vi "mainIRTesting.vi"() -> ()   [LabVIEW 2024]
doc: "Main VI for FLS imaging system."
uses:
  <userlib>/_OpenG.lib/file/file.llb/openg_file.lvlib
  <vilib>/event_ctls.llb/usereventprio.ctl
  <instrlib>/niScope/Acquire/Fetch/niScope Multi Fetch Binary 16.vi
  <instrlib>/niScope/Controls/niScope trigger source.ctl
  <userlib>/_OpenG.lib/time/time.llb/openg_time.lvlib
  LaguerreDeconLib/DeconEngineClass/LaguerreDeconEngineClass.lvclass
  SubVI/GlobalVariables.vi
  SubVI/LabJack/LJ Pin Setting.ctl
  <vilib>/Utility/error.llb/DialogType.ctl
  <vilib>/Analysis/NI_AALBase.lvlib
  <vilib>/Utility/miscctls.llb/LVMinMaxIncTypeDef.ctl
  <vilib>/Analysis/baseanly.llb/Mean (DBL).vi
  <vilib>/Utility/miscctls.llb/LVPointTypeDef.ctl
  <vilib>/addons/_JKI.lib/Serialization/JSON/JKI JSON Serialization.lvlib
  SubVI/APD/APDClass.lvclass
  ConfigFiles/AimingBeamVideoConfig.ctl
  <vilib>/addons/control/pid/NI_PID_pid.lvlib
  <vilib>/addons/control/pid/pid.llb/PID (DBL).vi
  <vilib>/Instr/_visa.llb/VISA Configure Serial Port (Instr).vi
  SubVI/DigitizerConfiguration/FLImDAQ.ctl
panel:
  in  "Square Wave?":bool
  in  "aimplitude":dbl=0.5 format="%#_13g"
  in  "aplitude":dbl=0.5 format="%#_13g"
  in  "amplitude":dbl=0.4
  in  "Modulation?":bool
  in  "f (Hz)":dbl=1.0
  in  "Gain DC 3":dbl
  in  "f (Hz)":dbl=1.0
  in  "Gain DC":dbl
  in  "Modulation?":bool
  in  "f (Hz)":dbl=1.0
  out "Peak3":dbl
  out "Peak2":dbl
  out "Peak1":dbl
  out "DC3":dbl format="%0.2f"
  out "DC2":dbl format="%0.2f"
  out "DC1":dbl format="%0.2f"
  in  "Gain DC":dbl
  in  "Modulation?":bool
  in  "V target(1.0)":dbl=1.0 caption="V target(1.5)" min=0.3 max=1.5 step=0.1 format="%#_4g"
  out "SNR3":dbl format="%#_3g"
  out "SNR2":dbl format="%#_3g"
  out "SNR1":dbl format="%#_3g"
  in  "Show BG removed?":bool
  out "IntR3":dbl format="%#_2g"
  out "IntR2":dbl format="%#_2g"
  out "IntR1":dbl format="%#_2g"
  in  "Video Display":bool
  out "Gain3":dbl
  out "Gain2":dbl
  out "Gain1":dbl
  in  "Skip Data Save?":bool
  out "Aq Loop?":bool
  out "ML?":bool
  out "aquisition loop Error Out":errorcluster
  out "Laser f (Hz)":dbl
  out "remote address":string
  out "Record Backlog":i32
  out "Fetch Record #":i32
  out "Sync Success?":bool
  out "Disclamer":picture
  out "Calibration #":i8
  out "BG #":i8
  in  "TCP Connect":bool
  out "Help":string
  in  "355nm Laser toggle":bool caption="355nm 460Hz"
  in  "Cali&iRF alignment":bool
  in  "Background":bool
  in  "Aiming beam toggle":bool caption="445nm 2Hz 22mA"
  out "Lifetime 3":dbl
  out "Lifetime 2":dbl
  in  "Auto gain ch3":bool=TRUE
  in  "Auto gain ch2":bool=TRUE
  in  "Auto gain ch1":bool=TRUE
  out "Run #":i8
  in  "StopButton":bool caption="Stop"
  out "Aquisition Status:":bool
  in  "StartButton":bool caption="Start"
  in  "V 3":dbl caption="Gain 3" min=0.0 max=4.65 step=0.1
  in  "V 2":dbl caption="Gain 2" min=0.0 max=4.59 step=0.1
  out "Lifetime 1":dbl
  in  "V 1":dbl caption="Gain 1" min=0.0 max=4.63 step=0.1 format="%#_4g"
  in  "Video Source":enum32{"Camera", "FrameGrabber"}(radio)
  out "Case #":string
  out "System Hardware Connection Status":T1
  out "Channel 3":dbl[][](graph)
  out "Channel 2":dbl[][](graph)
  out "Channel 1":dbl[][](graph)
  in  "Tab Control":T2(tab)
  out "display loop timing(ms)":u32
  out "Aquisition loop timing(ms)":u32 format="%.2f"
  out "DisplayLoop":i32
  out "PID loop":i32 caption="processing loop"
  out "PID loop timing(ms)":u32 caption="processing loop timing(ms)"
  out "Communication loop(ms)":u32
  out "laser EM lamp V":dbl format="%0.6f"
  out "Decon Loop timing (ms)":dbl
  in  "Show BG":bool
  out "iRF length":i32
  out "data length":i32
  out "BG length":i32
  out "SysConfigCluster":T3
  out "LJ Pinout":T4={"Ch1 Bias"="DAC0", "Ch2 Bias"="DAC1", "Ch3 Bias"="DAC2", "Ch4 Bias"="DAC0", "355 PWM"="FIO0", "AimingBeam PWM"="FIO2", "Laser Ready"="FIO3", "Interlock"="FIO1", "Laser Start/Stop"="FIO1", "Red LED"="FIO1", "Green LED"="DIO3", "Foot Pedal"="DIO15"}
  out "FLImDAQ":T5={"Digitizer 1"="", "Digitizer 2"="", "Channel"=enum."Channel 0", "trigger source"="VAL_EXTERNAL", "trigger level"=0.5, "trigger delay"=1.35e-07, "min sample rate"=12500000000.0, "min record length"=2500, "vertical range"=1.0, "vertical offset"=-0.25, "Waveform to Avg"=2000} caption="FLIm DAQ Configuration" {"trigger delay" format="%^#.4e"; "trigger level" min=0.0 max=3.5 step=0.5 format="%.2f"; "vertical offset" format="%.4f"; "vertical range" format="%.2f"; "min sample rate" format="%#.2p"}
  out "Dig1 Temp":dbl
  out "Dig2 Temp":dbl
  in  "Sys Reconfig":bool
  out "data out(communcation loop)":string
  out "syctimer data out":string
  out "PID loop error out":errorcluster caption="processing Error Out"
  out "decon error out":errorcluster
  out "Laser Rep Rate":dbl
  in  "Data Class":enum16{"Data", "BG", "Cali"}(ring)
  out "V1 Size":i32
  out "V2 Size":i32
  out "V3 Size":i32
  out "data Size":i32[](array[numeric])
  out "State log":string
  in  "Ch3 PID gains":T7={"proportional gain (Kc)"=30.0, "integral time (Ti, min)"=0.0003, "derivative time (Td, min)"=1e-05}
  in  "Ch2 PID gains":T7={"proportional gain (Kc)"=30.0, "integral time (Ti, min)"=0.0003, "derivative time (Td, min)"=1e-05}
  in  "Ch1 PID gains":T7={"proportional gain (Kc)"=30.0, "integral time (Ti, min)"=0.0003, "derivative time (Td, min)"=1e-05}
  in  "Quit":bool
  in  "Radio Buttons":enum32{"No Selection", "Ch1", "Ch2", "Ch3"}(radio)=enum."Ch1" caption="DeCon Chan"
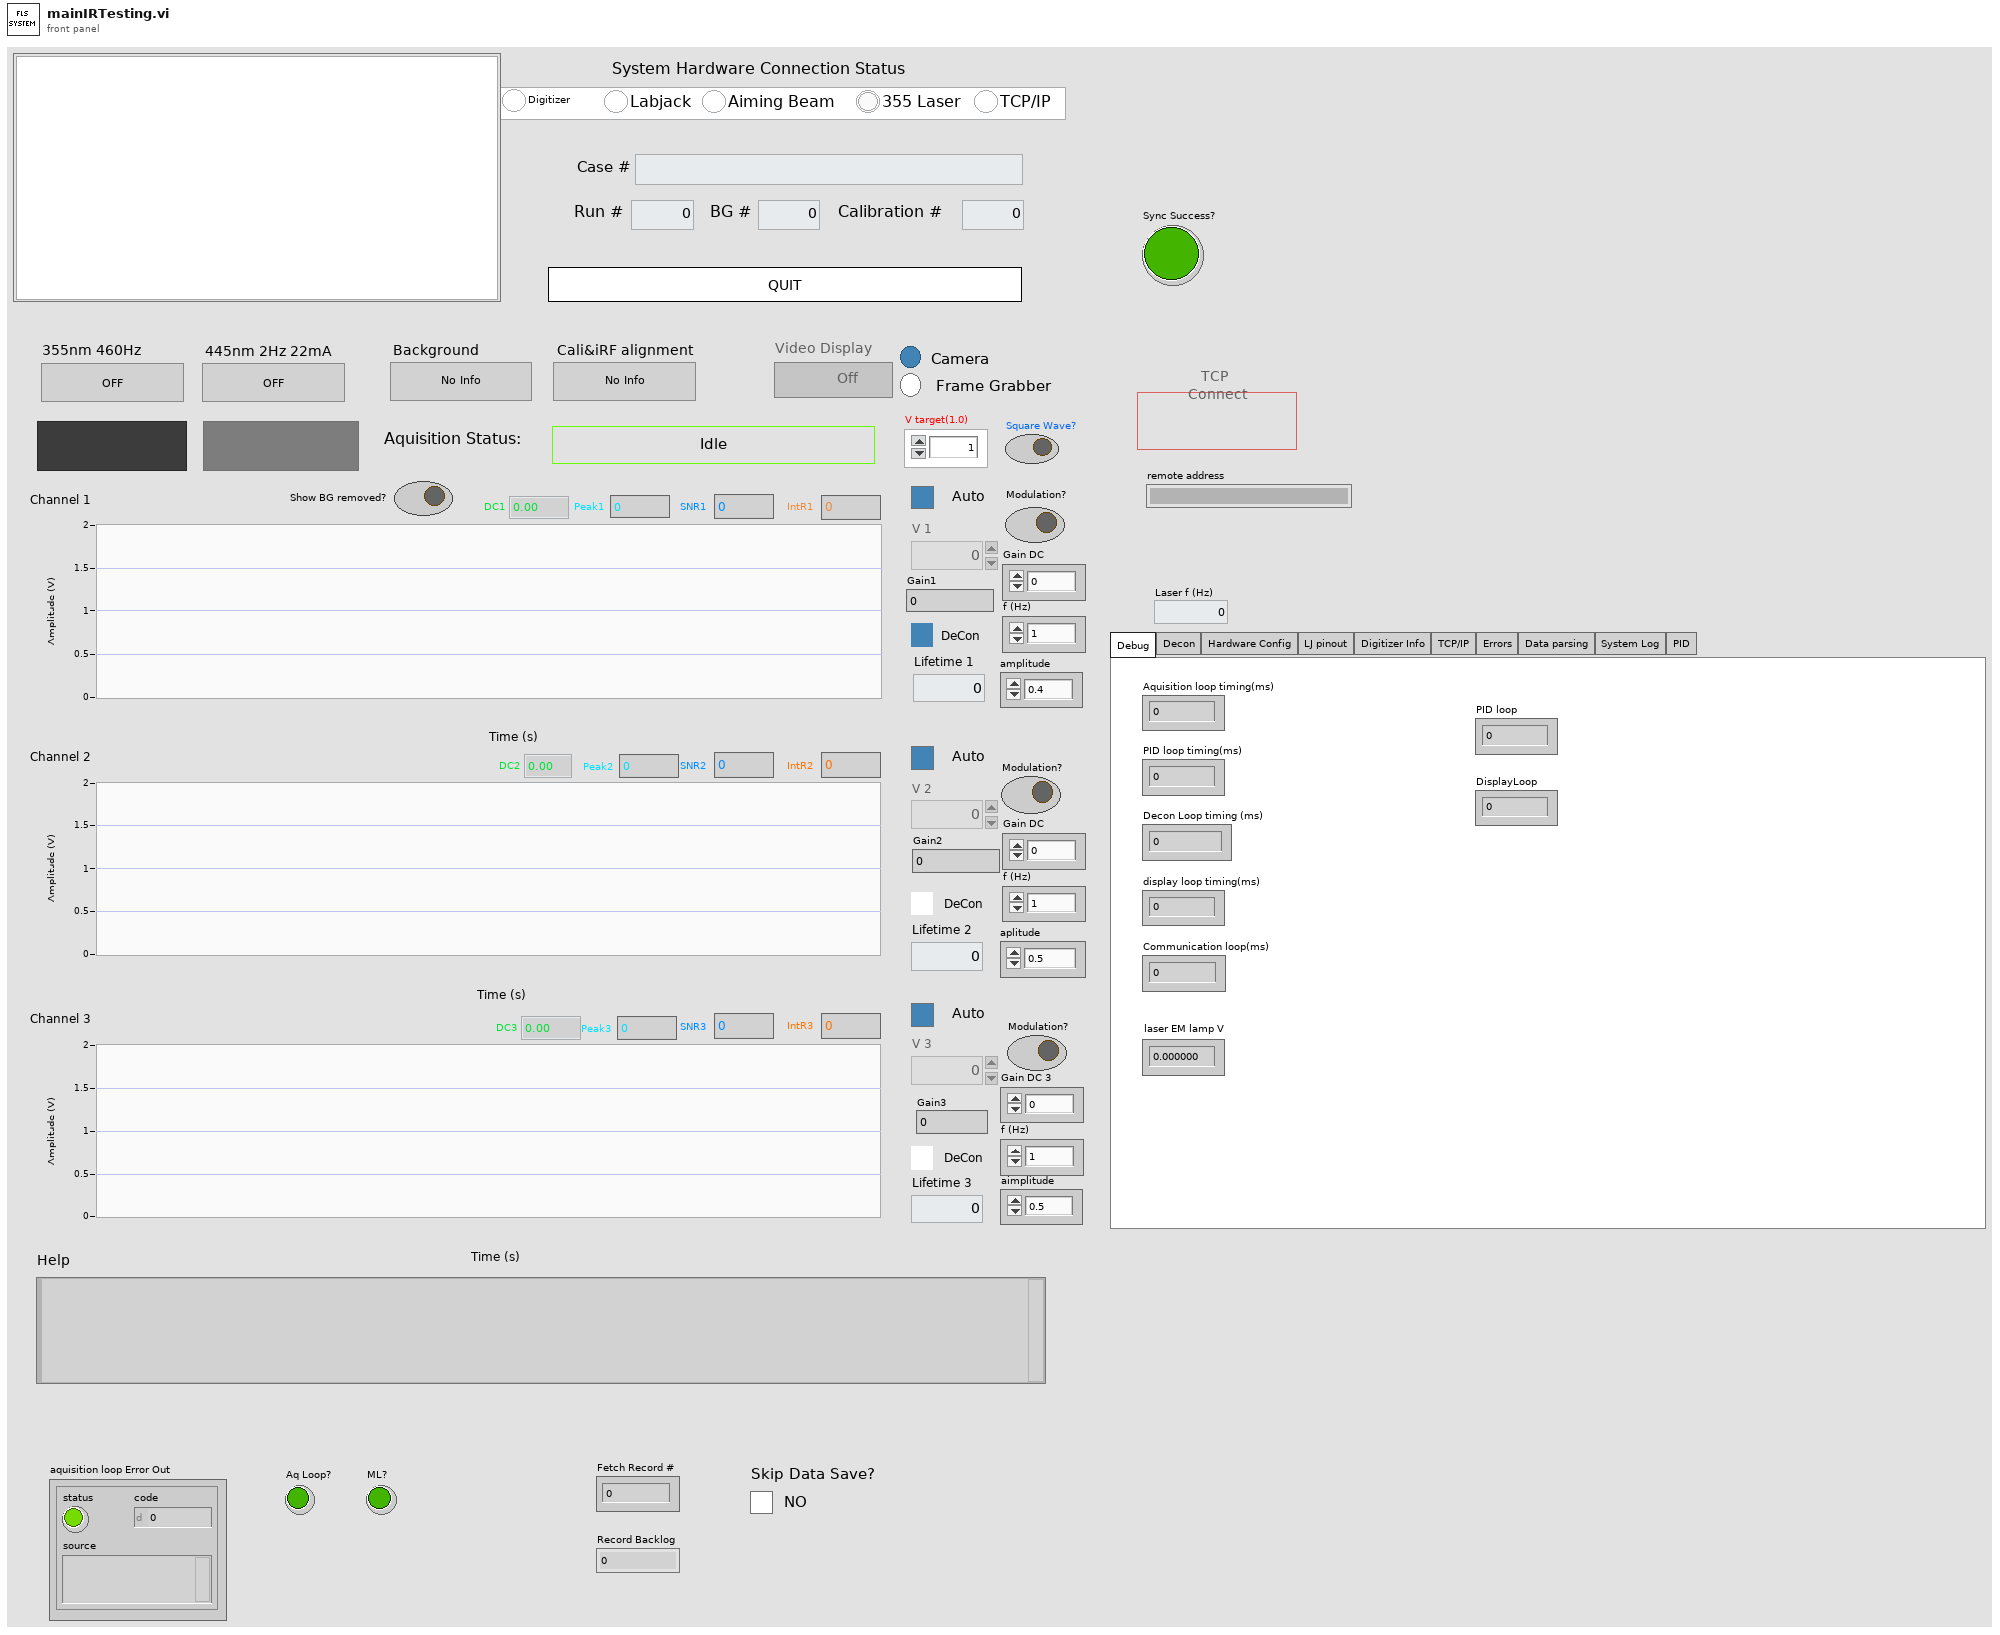
[diagram p1: front panel]
types:
  T1 = cluster{"Digitizer":bool, "Labjack":bool, "Aiming Beam":bool, "355 Laser":bool, "TCP/IP":bool}
  T2 = enum32{"Debug", "Decon", "Hardware Config", "LJ pinout", "Digitizer Info", "TCP/IP", "Errors", "Data parsing", "System Log", "PID"}
  T3 = cluster{"Ch1Enable?":bool, "Ch2Enable?":bool, "Ch3Enable?":bool, "Ch1AutoGain?":bool, "Ch2AutoGain?":bool, "Ch3AutoGain?":bool, "AimingBeamEnable?":bool}
  T4 = typedef "LJ Pin Setting.ctl" = cluster{"Ch1 Bias":string, "Ch2 Bias":string, "Ch3 Bias":string, "Ch4 Bias":string, "355 PWM":string, "AimingBeam PWM":string, "Laser Ready":string, "Interlock":string, "Laser Start/Stop":string, "Red LED":string, "Green LED":string, "Foot Pedal":string}
  T5 = typedef "FLImDAQ.ctl" = cluster{"Digitizer 1":refnum<k15>, "Digitizer 2":refnum<k15>, "Channel":enum16{"Channel 0", "Channel 1", "Channel 0&1"}, "trigger source":T6, "trigger level":dbl, "trigger delay":dbl, "min sample rate":dbl, "min record length":i32, "vertical range":dbl, "vertical offset":dbl, "Waveform to Avg":i16}
  T6 = typedef "niScope trigger source.ctl" = string
  T7 = cluster{"proportional gain (Kc)":dbl, "integral time (Ti, min)":dbl, "derivative time (Td, min)":dbl}
  T8 = enum8{"Enabled", "Disabled", "Disabled and Grayed Out"}
  T9 = enum16{"open", "replace", "create", "open or create", "replace or create", "replace or create with confirmation"}
  T10 = cluster{"CH1":dbl[][], "CH2":dbl[][], "CH3":dbl[][], "Gain cluster":cluster{"V1":dbl, "V2":dbl, "V3":dbl}}
  T11 = cluster{"idx":i32, "CH1&2":dbl[][], "CH3":dbl[][], "V cluster":cluster{"V1":dbl, "V2":dbl, "V3":dbl}}
  T12 = cluster{"Ch1 WF":dbl[], "Ch2 WF":dbl[], "Ch3 WF":dbl[], "V1":dbl, "V2":dbl, "V3":dbl}
  T13 = enum16{"open", "open or create", "create or replace", "create", "open (read-only)"}
  T14 = enum32{"Invalid", "Standard", "Closed", "Hidden", "Minimized", "Maximized"}
  T15 = enum32{"invalid app kind", "Development System", "Run Time System", "Student Edition", "Embedded LabVIEW", "Evaluation", "Custom"}
  T16 = typedef "usereventprio.ctl" = enum32{"high priority", "normal priority"}
  T17 = enum32{"Bad", "Idle", "Run top level", "Running"}
  T18 = enum16{"Standard", "Buffered", "CRLF", "Immediate"}
  T19 = typedef "AimingBeamVideoConfig.ctl" = cluster{"DeCon Channel":enum16{"1", "2", "3"}, "Scale Bar":bool, "Scale Low":dbl, "Scale High":dbl, "ANSI":dbl, "Radius":dbl, "3D?":bool, "Firefly?":bool, "Pentero?":bool}
  T20 = cluster{"Core":cluster{"Current VI Reference":refnum<vi>, "Close Panel on Exit?":bool}, "SysConfigCluster":cluster{"Ch1Enable?":bool, "Ch2Enable?":bool, "Ch3Enable?":bool, "Ch1AutoGain?":bool, "Ch2AutoGain?":bool, "Ch3AutoGain?":bool, "AimingBeamEnable?":bool}, "System Status":cluster{"Digitizer":bool, "Labjack":bool, "Aiming Beam":bool, "355 Laser":bool, "TCP/IP":bool}, "IDs":cluster{"RunID":i8, "BG ID":i8, "Cali ID":i8}, "CaseID":string, "DefaultPath":path, "Pathes":cluster{"DataPath":path, "BG Path":path, "iRFPath":path, "CaliPath":path}, "FLImDAQ":cluster{"resource name":refnum<k15>, "resource name 2":refnum<k15>, "Channel":enum16{"Channel 0", "Channel 1", "Channel 0&1"}, "trigger source":T6, "trigger level":dbl, "trigger delay":dbl, "min sample rate":dbl, "min record length":i32, "vertical range":dbl, "vertical offset":dbl, "Waveform to Avg":i32}, "SysRunning?":bool, "AB Cluster":cluster{"Aiming Beam COM Port":refnum<visa-resource-name>, "Min Current":dbl, "Max Current":dbl, "Default Current":dbl, "Freq":i32}, "LJ Pinout":T4, "355 PWM setting":cluster{"DIO_EF_CLOCK1_DIVISOR":i16, "DIO_EF_CLOCK1_ROLL_VALUE":i32, "DIO#_EF_INDEX":i16, "DIO#_EF_OPTIONS":i16, "DIO#_EF_CONFIG_A":i32}, "AB PWM setting":cluster{"DIO_EF_CLOCK1_DIVISOR":i16, "DIO_EF_CLOCK1_ROLL_VALUE":i32, "DIO#_EF_INDEX":i16, "DIO#_EF_OPTIONS":i16, "DIO#_EF_CONFIG_A":i32}, "Last Trigger":u32, "niTClk sessions":refnum<k20>[], "Laser start tic":u32, "TCP attempt count":i32, "Ch1Data":dbl[][], "Ch2Data":dbl[][], "Ch3Data":dbl[][], "V1":dbl[], "V2":dbl[], "V3":dbl[], "SlowTimer":u32, "FastTimer":u32, "listener ID":refnum<k5>, "TempPath":path, "LED vi reference":refnum<vi>, "Aquisition Timer":u32, "APDSerialNum":cluster{"Ch1APDSerial#":string, "Ch2APDSerial#":string, "Ch3APDSerial#":string}, "VideoConfig":T19, "CaliPath":path}
  T21 = typedef "LVCursorListTypeDef.ctl" = cluster{"Name":string, "Color":u32, "Style":u8, "Point Style":u8, "Name Visible":bool, "Allow Drag":bool, "Cursor Mode":u32, "Plot":i32, "Index":i32, "Position":cluster{"X":dbl, "Y":dbl}, "X Scale":u32, "Y Scale":u32, "Watch Plots":i32[], "Watch All Plots":bool, "Plot Area":i32, "Label Offset":cluster{"X":dbl, "Y":dbl}}[]
  T22 = cluster{"Name":string, "Color":u32, "Style":u8, "Point Style":u8, "Name Visible":bool, "Allow Drag":bool, "Cursor Mode":u32, "Plot":i32, "Index":i32, "Position":cluster{"X":dbl, "Y":dbl}, "X Scale":u32, "Y Scale":u32, "Watch Plots":i32[], "Watch All Plots":bool, "Plot Area":i32, "Label Offset":cluster{"X":dbl, "Y":dbl}}
  T23 = cluster{"Ch1APDSerial#":string, "Ch2APDSerial#":string, "Ch3APDSerial#":string}
  T24 = cluster{"DataPath":path, "BG Path":path, "iRFPath":path, "CaliPath":path}
  T25 = cluster{"DIO_EF_CLOCK1_DIVISOR":i16, "DIO_EF_CLOCK1_ROLL_VALUE":i32, "DIO#_EF_INDEX":i16, "DIO#_EF_OPTIONS":i16, "DIO#_EF_CONFIG_A":i32}
  T26 = cluster{"Aiming Beam COM Port":refnum<visa-resource-name>, "Min Current":dbl, "Max Current":dbl, "Default Current":dbl, "Freq":i32}
  T27 = cluster{"resource name":refnum<k15>, "resource name 2":refnum<k15>, "Channel":enum16{"Channel 0", "Channel 1", "Channel 0&1"}, "trigger source":T6, "trigger level":dbl, "trigger delay":dbl, "min sample rate":dbl, "min record length":i32, "vertical range":dbl, "vertical offset":dbl, "Waveform to Avg":i32}
  T28 = cluster{"Current VI Reference":refnum<vi>, "Close Panel on Exit?":bool}
  T29 = typedef "iRFData.ctl" = cluster{"dt":dbl, "NumOfWFs":i32, "WFLength":i32, "iRFCtrlV":dbl[], "iRFWFsAvg":dbl[][], "iRFRaw":dbl[][]}
  T30 = cluster{"iRFWFsAvg":dbl[], "iRFWFsAvg":dbl[], "iRFWFsAvg":dbl[]}
  T31 = cluster{"V 1":dbl[], "V 2":dbl[], "V 3":dbl[], "V 4":dbl[]}
  T32 = cluster{"Channel 1":dbl[], "Channel 2":dbl[], "Channel 3":dbl[], "Channel 4":dbl[]}
  T33 = cluster{"DataPath":path, "CaseID":string, "RunID":i16, "Ch1Data":dbl[][], "Ch2Data":dbl[][], "Ch3Data":dbl[][], "V1":dbl[], "V2":dbl[], "V3":dbl[], "LaserRepRate":i16, "WFAverage":i16}
  T34 = typedef "DialogType.ctl" = u16
  T35 = cluster{"Ch1 iRF":dbl[], "Ch2 iRF":dbl[], "Ch3 iRF":dbl[], "Ch4 iRF":dbl[]}
  T36 = typedef "LJ PWM Setting.ctl" = cluster{"DIO_EF_CLOCK1_DIVISOR":i16, "DIO_EF_CLOCK1_ROLL_VALUE":i32, "DIO#_EF_INDEX":i16, "DIO#_EF_OPTIONS":i16, "DIO#_EF_CONFIG_A":i32}
  T37 = typedef "AimingBeam.ctl" = cluster{"Aiming Beam COM Port":refnum<visa-resource-name>, "Min Current":dbl, "Max Current":dbl, "Default Current":dbl, "Frequency(Hz)":u32}
  T38 = cluster{"DC1":i32, "DC2":i32, "BG1":i32, "BG2":i32}
  T39 = typedef "LVMinMaxIncTypeDef.ctl" = cluster{"Minimum":dbl, "Maximum":dbl, "Increment":dbl}
  T40 = typedef "LVBoundsTypeDef.ctl" = cluster{"Width":u32, "Height":u32}
  T41 = typedef "imagedata.ctl" = cluster{"image type":i32, "image depth":i32, "image":u8[], "mask":u8[], "colors":u32[], "Rectangle":cluster{"left":i16, "top":i16, "right":i16, "bottom":i16}}
  T42 = enum32{"No Selection", "Ch1", "Ch2", "Ch3", "Ch4"}
  T43 = cluster{"DC Idx1":i32, "DC Idx2":i32, "BG Idx1":i32, "BG Idx2":i32}
  T44 = cluster{"Ch1APDSerial#":string, "Ch2APDSerial#":string, "Ch3APDSerial#":string, "Ch4APDSerial#":string}
  T45 = cluster{dbl[][], dbl[][], dbl[][], "V cluster":cluster{"V1":dbl, "V2":dbl, "V3":dbl}}
  T46 = typedef "LVPointTypeDef.ctl" = cluster{"Horizontal":i16, "Vertical":i16}
  T47 = cluster{"actualSamples":i32, "absoluteInitialX":dbl, "relativeInitialX":dbl, "xIncrement":dbl, "offset":dbl, "gain":dbl, "reserved1":dbl, "reserved2":dbl}[]
  T48 = cluster{"V1 out":dbl, "V2 out":dbl, "V3 out":dbl}
  T49 = cluster{i32, dbl[][], dbl[][], cluster{"V1 out":dbl, "V2 out":dbl, "V3 out":dbl}}
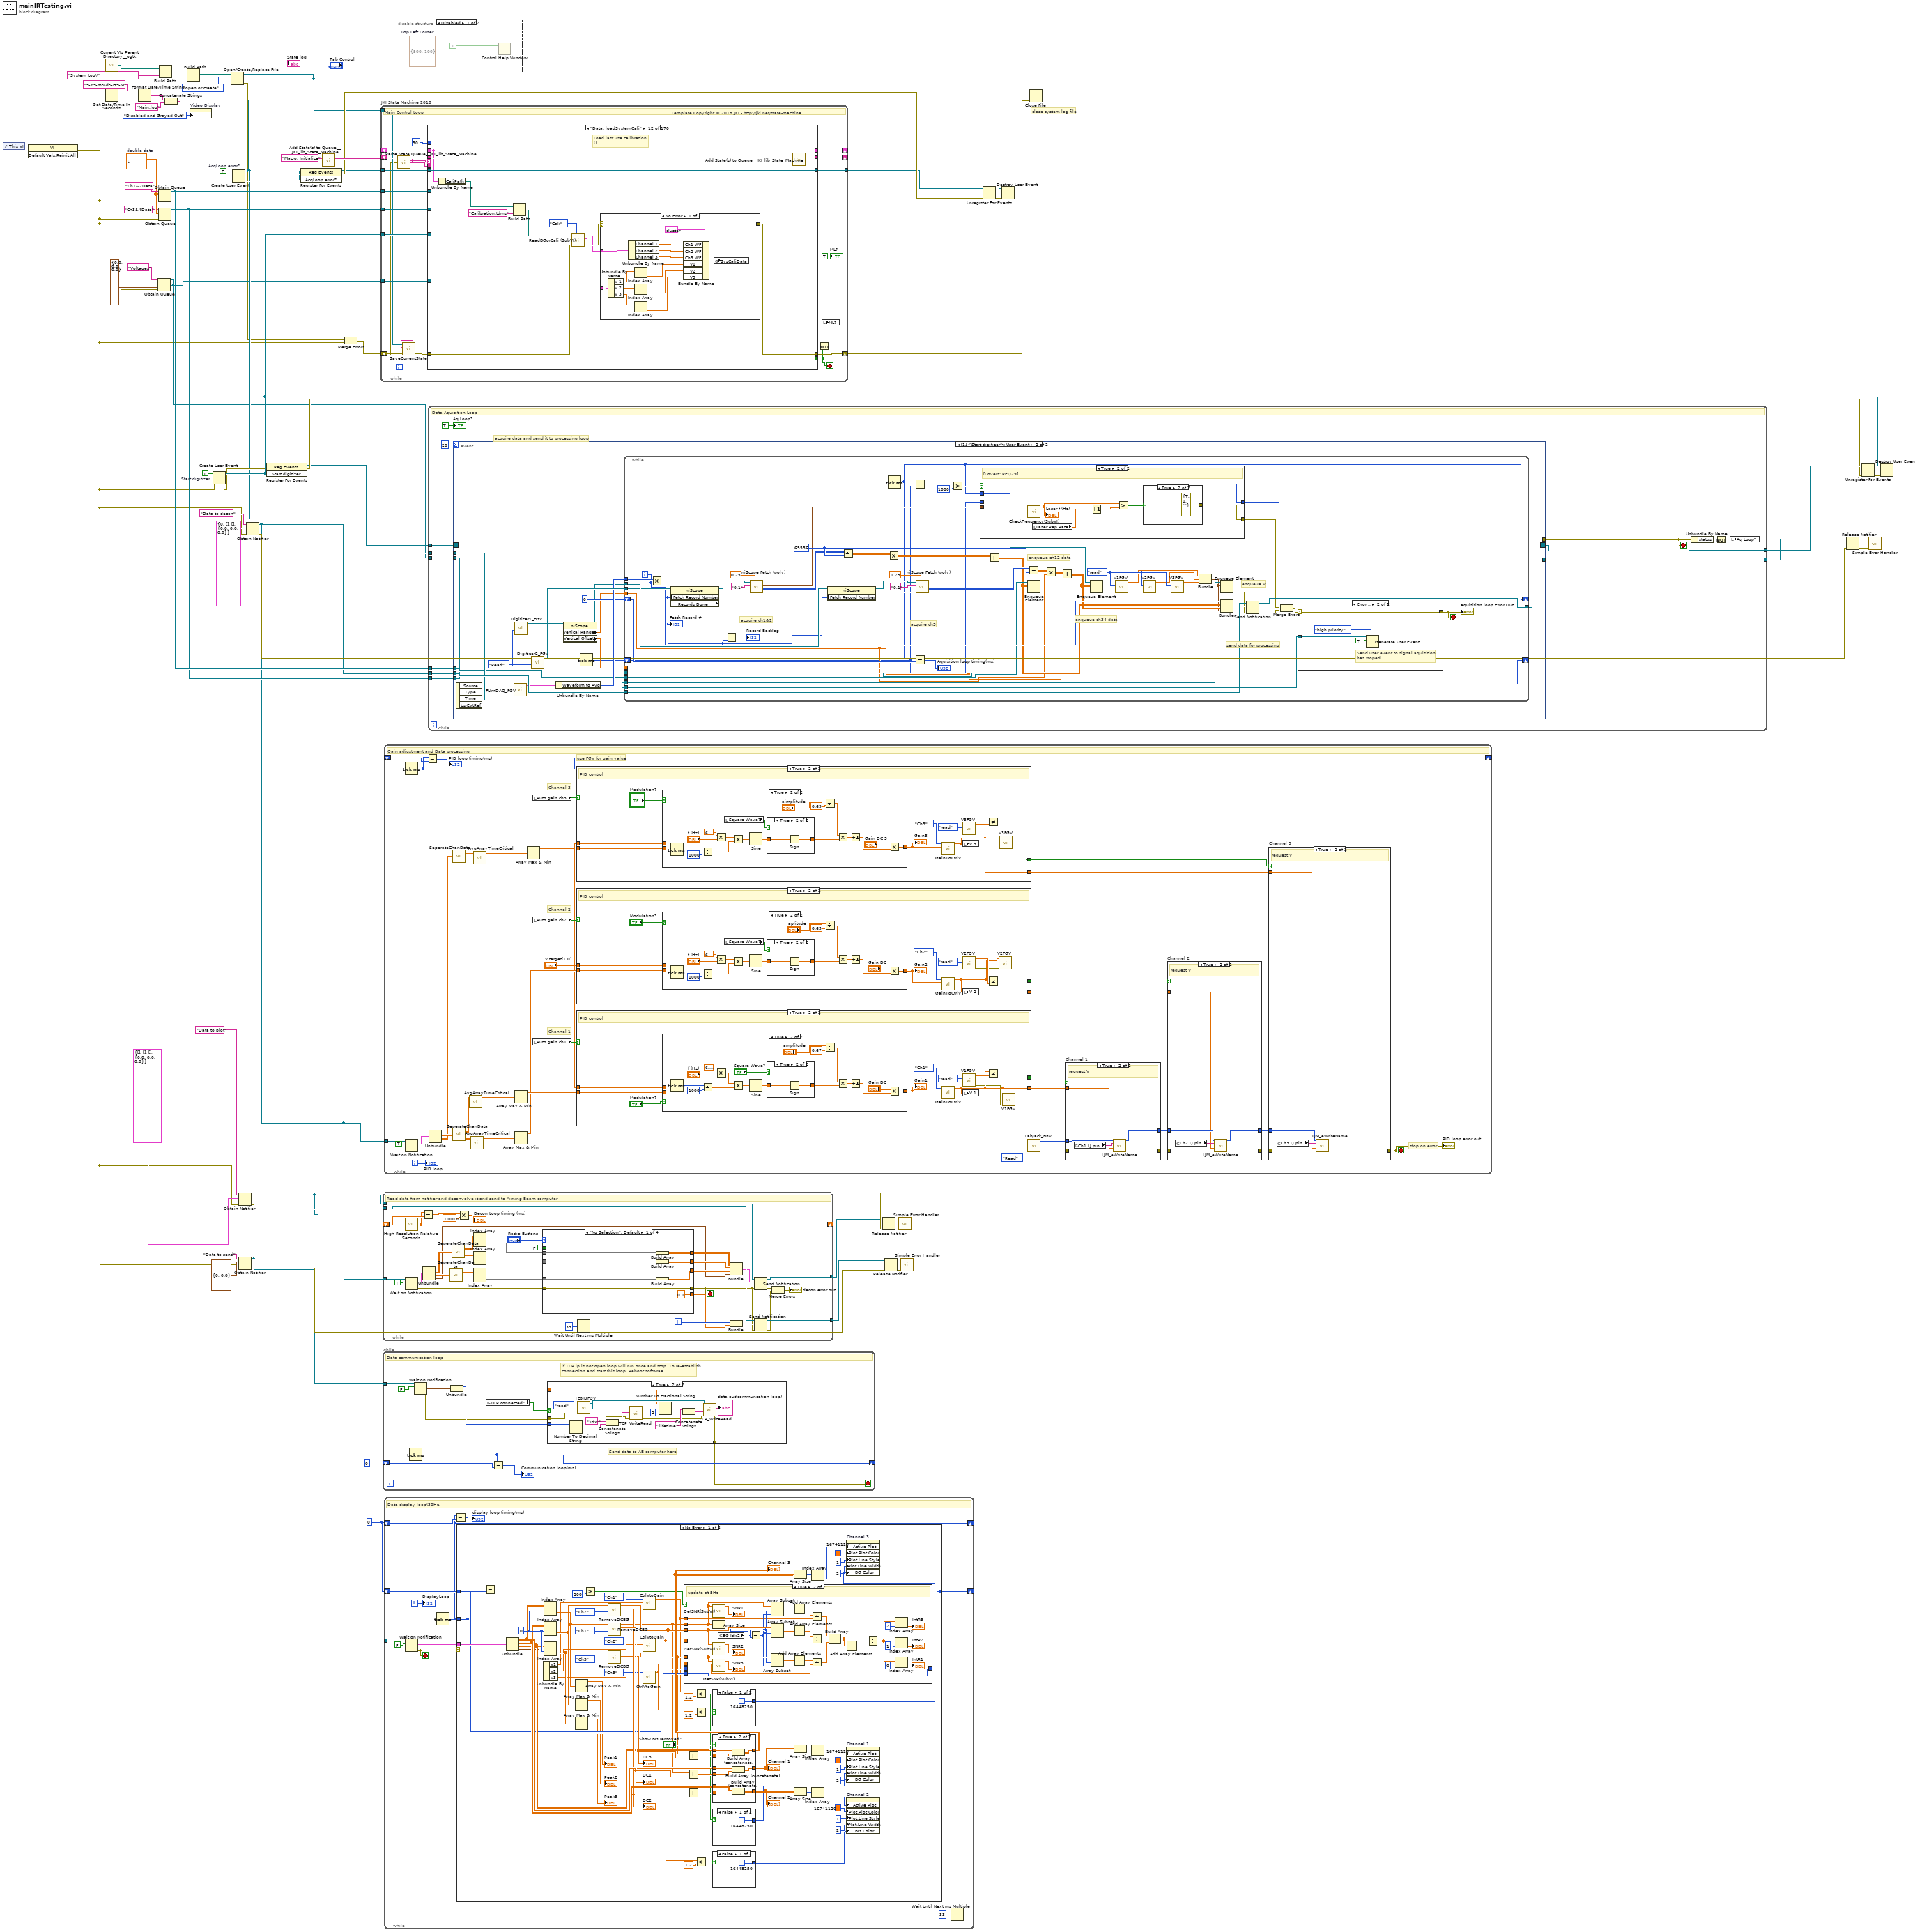
[diagram p0: block diagram]
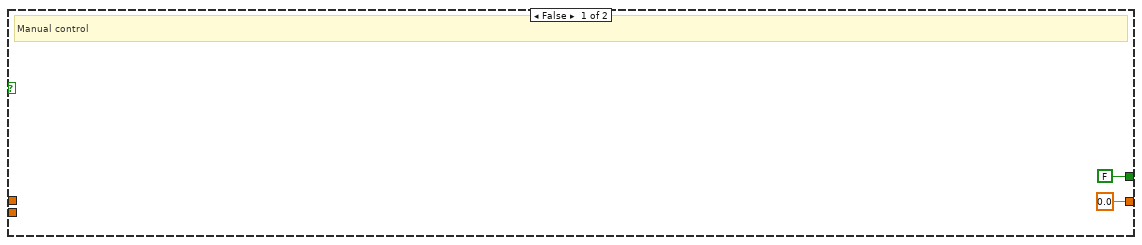
[diagram p2: hidden frame]
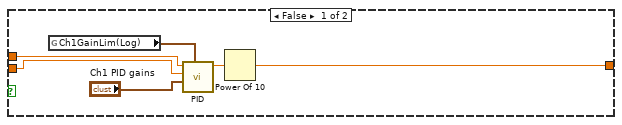
[diagram p3: hidden frame]
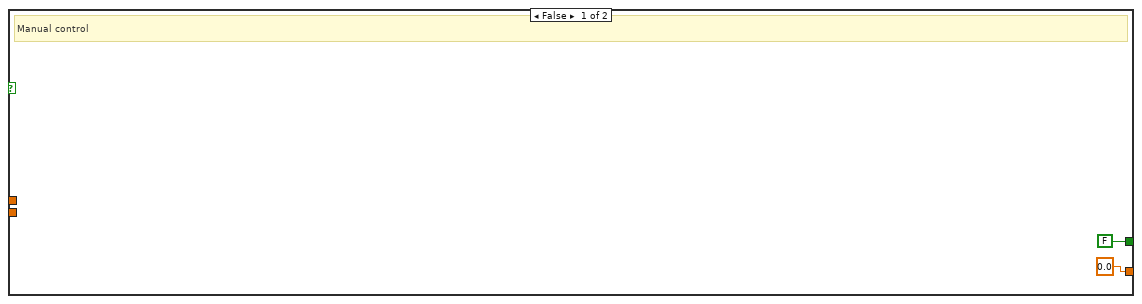
[diagram p8: hidden frame]
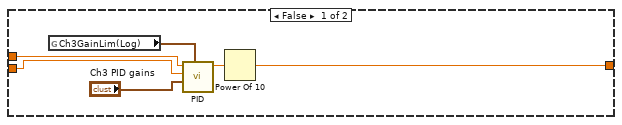
[diagram p9: hidden frame]
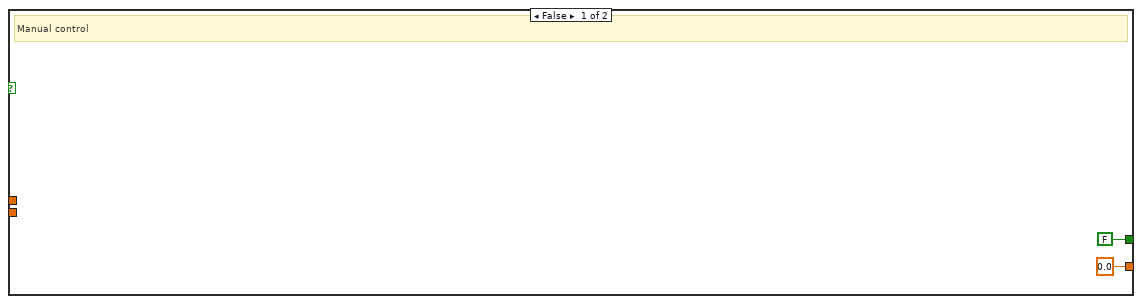
[diagram p11: hidden frame]
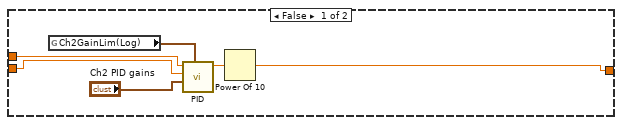
[diagram p12: hidden frame]
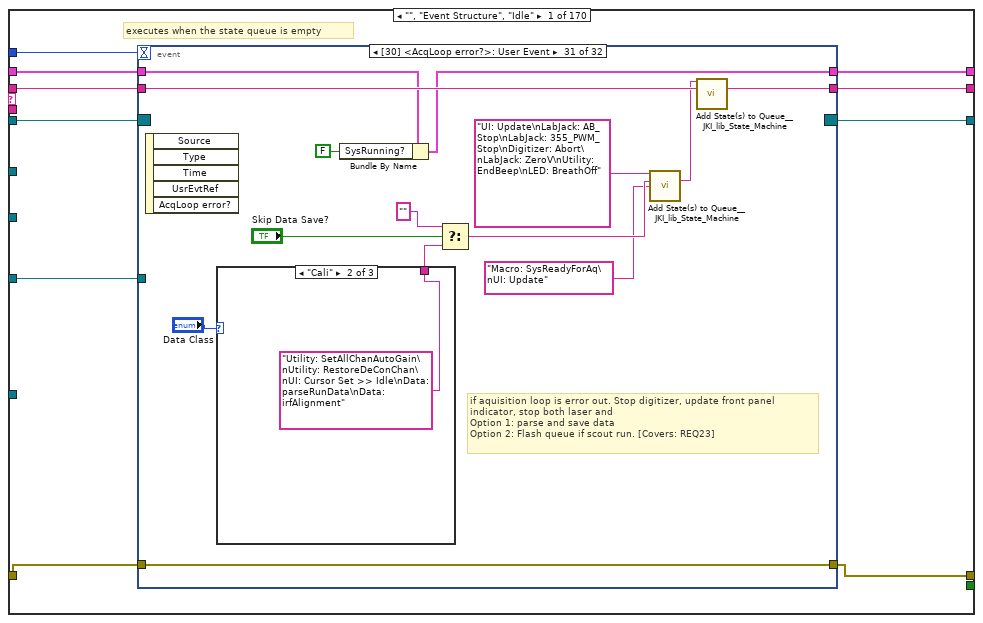
[diagram p14: hidden frame]
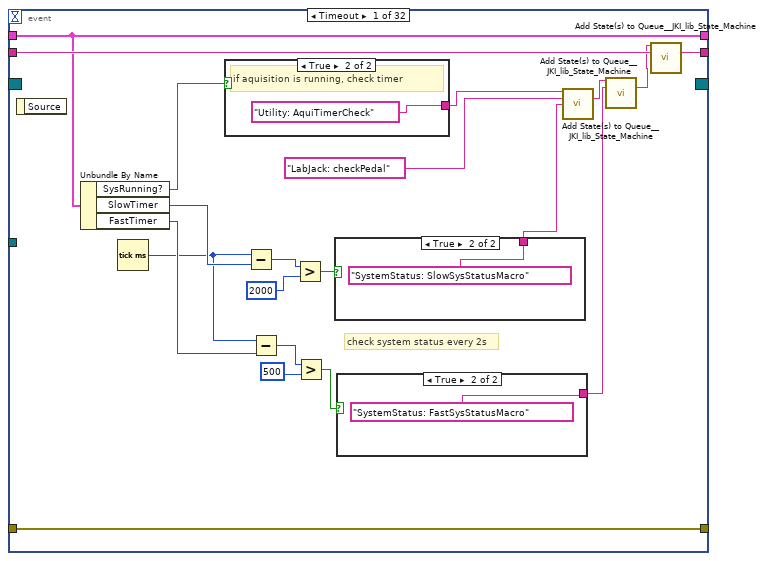
[diagram p15: hidden frame]
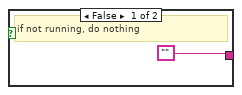
[diagram p16: hidden frame]
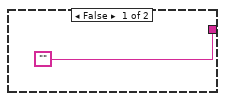
[diagram p17: hidden frame]
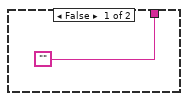
[diagram p18: hidden frame]
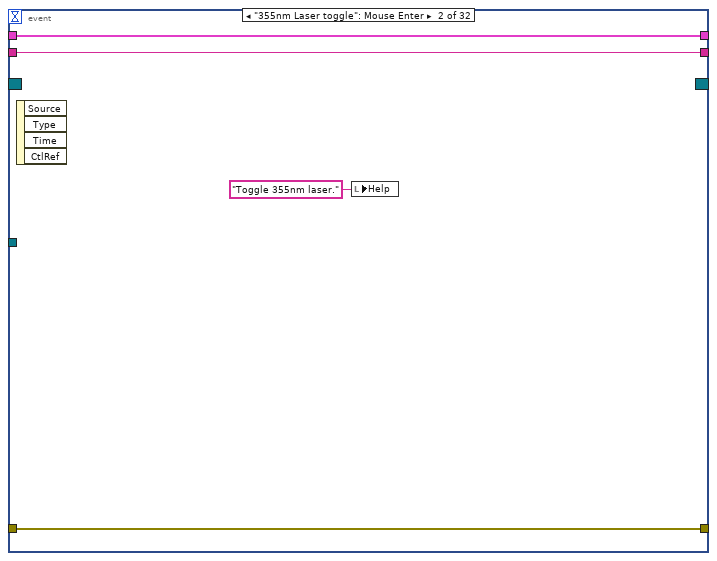
[diagram p19: hidden frame]
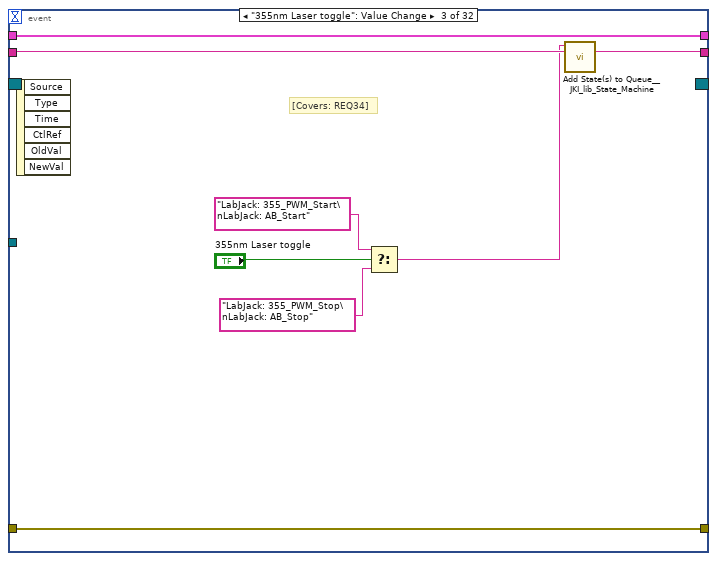
[diagram p20: hidden frame]
diagram:
  w1 = u32 0 ("millisecond timer value")
  w44 = FALSE  # AcqLoop error?
  w54 = TRUE  # Start digitizer
  w57 = dbl[][] []  # double data
  # "close system log file"
  n1 = control-ref of="This VI"() -> (w59:refnum<vi>)
  n2 = invoke on="Invoke Node" class="VI" method="Default Vals.Reinit All"(reference=w59) -> (error out=w11:errorcluster)  [unwired: 2 in, 2 out]
  n3 = call <userlib>:"Current VIs Parent Directory__ogtk.vi"() -> ("Parent Directory (+ Relative)"=w22:path)  [unwired: 5 in]
  n4 = Get Date/Time In Seconds() -> (seconds since 1Jan1904=w20:timestamp)
  n5 = Format Date/Time String(time format string (%c)="%Y%m%d%H%M", seconds (now)=w20) -> (date/time string=w17:string)  [unwired: 1 in]
  n6 = Obtain Queue(name (unnamed)="Voltages", element data type=cluster{"V1":dbl, "V2":dbl, "V3":dbl} {"V1"=0.0, "V2"=0.0, "V3"=0.0}, error in (no error)=w11) -> (queue out=w23:refnum<queue>)  [unwired: 2 in, 2 out]
  n7 = Obtain Queue(name (unnamed)="Ch3&4Data", element data type=w57, error in (no error)=w11) -> (queue out=w36:refnum<queue>)  [unwired: 2 in, 2 out]
  n8 = Obtain Queue(name (unnamed)="Ch1&2Data", element data type=w57, error in (no error)=w11) -> (queue out=w55:refnum<queue>)  [unwired: 2 in, 2 out]
  n9 = Build Path(base path=w22, name or relative path="System Log\\") -> (appended path=w13:path)
  n10 = Concatenate Strings(w17, "Main.log" ("string")) -> (w15:string)
  n11 = Build Path(base path=w13, name or relative path=w15) -> (appended path=w18:path)
  n12 = property on="Video Display" class="Bool (strict)"("DisabledEnum"=T8."Disabled and Grayed Out" ("Disabled")) -> ()  [unwired: 2 in, 2 out]
  n13 = Create User Event(user event datatype=w54, error in=w11) -> (user event=w43:refnum<user-event>, error out=w28:errorcluster)
  n14 = Open/Create/Replace File(file path (use dialog)=w18, operation (0:open)=T9."open or create") -> (refnum out=w9:refnum<file>, error out=w10:errorcluster)  [unwired: 4 in, 1 out]
  n15 = Create User Event(user event datatype=w44) -> (user event=w27:refnum<user-event>, error out=w29:errorcluster)  [unwired: 1 in]
  n16 = Obtain Notifier(name (unnamed)="Data to plot", notification data type=T10 {"CH1"=[], "CH2"=[], "CH3"=[], "Gain cluster"={"V1"=0.0, "V2"=0.0, "V3"=0.0}}, error in (no error)=w11) -> (notifier out=w3:refnum<notifier>, error out=w37:errorcluster)  [unwired: 1 in, 1 out]
  n17 = Obtain Notifier(name (unnamed)="Data to send", notification data type=cluster{"idx":i32, "lifetime":dbl} {"idx"=0, "lifetime"=0.0}, error in (no error)=w11) -> (notifier out=w5:refnum<notifier>, error out=w26:errorcluster)  [unwired: 1 in, 1 out]
  n18 = Obtain Notifier(name (unnamed)="Data to decon", notification data type=T11 {"idx"=0, "CH1&2"=[], "CH3"=[], "V cluster"={"V1"=0.0, "V2"=0.0, "V3"=0.0}}, error in (no error)=w11) -> (notifier out=w6:refnum<notifier>, error out=w48:errorcluster)  [unwired: 1 in, 1 out]
  n19 = register-events(error in=w28, w43) -> (reference out=w45:refnum<event-registration>, error out=w51:errorcluster)  [unwired: 1 in]
  n20 = register-events(error in=w29, w27) -> (reference out=w35:refnum<event-registration>, error out=w41:errorcluster)  [unwired: 1 in]
  n21 = call <vilib>:"Add State(s) to Queue__JKI_lib_State_Machine.vi"("State(s) in (\"\")"="Macro: Initialize") -> ("States Out"=w61:string)  [unwired: 14 in]
  n22 = Merge Errors(w10, w11) -> (w12:errorcluster)
  n23 = while "JKI State Machine 2018" {
    shift-right: [w77] -> _
    shift-left: _ -> [w76]
    shift-right: [w79] -> w8
    shift-left: w12 -> [w63]
    shift-right: [w78] -> _
    shift-left: w61 -> [w80]
    tunnel: w55 -> [w74]
    tunnel: w36 -> [w73]
    tunnel: w43 -> [w72]
    tunnel: w35 -> [w71]
    tunnel: [w70] -> w34
    tunnel: w23 -> [w66]
    tunnel: w9 -> [w65]
    stop <- w69 stop-if-true
    # "Template Copyright © 2018 JKI - http://jki.net/state-machine"
    # "Main Control Loop"
    n24 = call <vilib>:"Parse State Queue__JKI_lib_State_Machine.vi"("State Queue"=w80, "Error In (no error)"=w63) -> ("Remaining States"=w82:string, "Current State"=w64:string, "Arguments"=w81:string)  [unwired: 11 in]
    n25 = call "SaveCurrentState.vi"("error in (no error)"=w63, "Current State"=w64, "Byte Stream File in"=w65) -> ("error out"=w62:errorcluster)  [unwired: 8 in]
    n26 = case shown="\"Data: loadSystemCali\"" w64 {
      selector: w64 -> [_ _ _ _ _ _ _ _ _ _ _ _ _ _ _ _ _ _ _ _ _ _ _ w890 _ _ _ _ _ _ _ _ _ _ _ _ _ _ _ _ _ _ _ _ _ _ _ _ _ _ _ _ _ _ _ _ _ _ _ _ _ _ _ _ _ _ _ _ _ _ _ _ _ _ _ _ _ _ _ _ _ _ _ _ _ _ _ _ _ _ _ _ _ _ _ _ _ _ _ _ _ _ _ _ _ _ _ _ _ _ _ _ _ _ _ _ _ _ _ _ _ _ _ _ _ _ _ _ _ _ _ _ _ _ _ _ _ _ _ _ _ _ _ _ _ _ _ _ _ _ _ _ _ _ _ _ _ _ _ _ _ _ _ _ _ _ _ _ _ _]
      tunnel: w82 -> [w92 w411 w420 w426 w432 w455 w470 w507 w541 w572 w598 w622 w662 w674 w698 w726 w738 w764 w777 w844 w870 w883 w888 w894 w921 w929 w952 w957 w969 w978 w995 w1004 w1027 w1044 w1057 w1076 w1102 w1128 w1166 w1171 w1177 w1203 w1229 w1255 w1260 w1277 w1325 w1347 w1363 w1375 w1391 w1396 w1408 w1437 w1461 w1472 w1510 w1521 w1527 w1538 w1550 w1581 w1594 w1608 w1623 w1642 w1677 w1682 w1695 w1702 w1714 w1726 w1738 w1766 w1781 w1786 w1797 w1809 w1814 w1822 w1830 w1838 w1846 w1851 w1867 w1876 w1894 w1910 w1930 w1941 w1963 w1976 w1987 w1992 w2000 w2008 w2013 w2021 w2028 w2035 w2045 w2073 w2081 w2088 w2096 w2101 w2108 w2114 w2120 w2128 w2142 w2149 w2161 w2231 w2242 w2255 w2280 w2303 w2309 w2325 w2347 w2355 w2361 w2366 w2373 w2383 w2395 w2404 w2409 w2421 w2426 w2436 w2444 w2452 w2457 w2462 w2467 w2477 w2499 w2518 w2523 w2534 w2555 w2574 w2593 w2598 w2626 w2655 w2700 w2710 w2728 w2748 w2762 w2782 w2802 w2812 w2824 w2841 w2862 w2886 w2905 w2923 w2941 w2959 w2973 w2987 w3001 w3013 w3022 w3027]
      tunnel: w81 -> [_ _ _ _ _ _ _ _ _ _ _ _ _ _ _ _ _ _ _ _ _ _ _ _ _ _ _ _ _ _ _ w1001 _ _ _ _ _ _ _ _ _ _ _ _ _ _ _ _ _ _ _ _ _ _ _ _ _ _ _ _ w1548 _ _ _ _ _ _ _ _ _ _ _ _ _ _ _ _ _ _ _ _ _ _ _ _ _ _ _ _ _ _ _ _ _ _ _ _ _ _ _ w2036 _ _ _ _ _ _ _ _ _ _ w2144 w2155 _ _ _ _ w2299 _ _ _ _ _ _ w2368 _ _ _ _ _ _ w2432 _ _ _ _ _ _ _ _ _ _ _ _ _ _ _ _ _ _ _ _ _ _ _ _ _ _ _ _ _ _ _ _ _ _ _ _ _ _]
      tunnel: w76 -> [w90 w408 w416 w423 w429 w452 w467 _ w538 w564 w588 w618 w658 w670 w689 w716 w735 w741 w774 w803 w856 w878 w885 w892 w914 w926 w950 w954 w959 w972 w993 w1002 w1017 w1041 w1045 w1066 w1092 w1120 w1162 w1168 w1174 w1181 w1208 w1234 w1257 w1270 w1315 w1344 w1348 w1372 w1388 w1393 w1397 w1426 w1451 w1465 w1489 w1519 w1524 w1531 w1546 w1564 w1589 w1600 w1618 w1635 w1660 w1679 w1691 w1696 w1711 w1723 w1735 w1754 w1770 w1783 w1795 w1807 w1811 w1816 w1823 w1833 w1841 w1848 w1854 w1873 w1881 w1897 w1925 w1931 w1960 w1969 w1985 w1989 w1993 w2001 w2010 w2019 w2025 w2032 w2042 w2070 w2078 w2085 w2093 w2098 w2106 w2112 w2117 w2122 w2139 w2147 w2157 w2228 w2239 w2249 w2273 w2300 w2306 w2318 w2343 w2352 w2358 w2363 w2370 w2377 w2391 w2401 w2406 w2418 w2423 w2429 w2441 w2449 w2454 w2459 w2464 w2474 w2497 w2516 w2520 w2532 w2553 w2572 w2591 w2595 w2607 w2651 w2697 w2706 w2723 w2743 w2757 w2780 w2798 w2804 w2818 w2836 w2857 w2881 w2900 w2918 w2936 w2954 w2968 w2982 w2996 w3010 w3020 w3024]
      tunnel: [w89 w409 w418 w424 w430 w453 w468 w505 w536 w561 w596 w610 w640 w672 w679 w703 w727 w739 w775 w838 w855 w879 w886 w896 w918 errorcluster {"status"=FALSE, "code"=0, "source"=""} ("error out") w949 w955 w963 w975 w985 w998 w1018 w1042 w1055 w1074 w1100 w1119 w1164 w1169 w1175 w1182 w1209 w1235 w1258 w1267 w1307 w1338 w1352 w1373 w1379 w1394 w1400 w1424 w1447 w1464 w1477 w1513 w1525 w1536 w1540 w1555 w1584 w1596 w1614 w1634 w1651 w1680 w1689 w1698 w1709 w1721 w1733 w1756 w1771 w1784 w1787 w1804 w1812 w1820 w1828 w1836 w1844 w1849 w1853 w1869 w1884 w1905 w1924 w1935 w1953 w1973 w1983 w1990 w1998 w2006 w2011 w2018 w2026 w2033 w2043 w2071 w2079 w2086 w2094 w2099 w2105 w2111 w2118 w2125 w2140 w2145 w2158 w2229 w2238 w2251 w2275 w2301 w2307 w2310 w2337 w2353 w2359 w2364 w2371 w2381 w2393 w2402 w2407 w2419 w2424 w2434 w2442 w2450 w2455 w2460 w2465 w2475 w2487 w2509 w2521 w2525 w2539 w2562 w2583 w2596 w2609 w2652 w2698 w2705 w2725 w2745 w2759 w2770 w2800 w2803 w2820 w2838 w2859 w2883 w2902 w2920 w2938 w2956 w2970 w2984 w2998 w3011 w3018 w3025] -> w79
      tunnel: w62 -> [w88 w409 w418 w424 w430 w453 w468 w505 w536 w562 w596 w615 w641 w672 w680 w712 w727 w740 w775 w838 w848 w880 w886 w895 w918 w922 w949 w955 w964 w974 w981 w997 w1019 w1042 w1055 w1074 w1100 w1118 w1164 w1169 w1175 w1186 w1213 w1239 w1258 w1266 w1310 w1337 w1351 w1373 w1381 w1394 w1399 w1425 w1450 w1470 w1482 w1512 w1525 w1533 w1543 w1554 w1583 w1599 w1613 w1633 w1650 w1680 w1688 w1699 w1708 w1720 w1732 w1755 w1772 w1784 w1791 w1799 w1812 w1820 w1828 w1836 w1844 w1849 w1852 w1870 w1889 w1904 w1923 w1934 w1959 w1972 w1982 w1990 w1998 w2006 w2011 w2018 w2026 w2033 w2043 w2071 w2079 w2086 w2094 w2099 w2105 w2111 w2118 w2125 w2140 w2146 w2159 w2229 w2238 w2246 w2278 w2301 w2307 w2320 w2336 w2353 w2359 w2364 w2371 w2381 w2393 w2402 w2407 w2419 w2424 w2434 w2442 w2450 w2455 w2460 w2465 w2475 w2486 w2508 w2521 w2524 w2538 w2567 w2588 w2596 w2624 w2652 w2698 w2704 w2724 w2744 w2758 w2775 w2800 w2807 w2819 w2837 w2858 w2882 w2901 w2919 w2937 w2955 w2969 w2983 w2997 w3011 w3017 w3025]
      tunnel: [w91 w410 w419 w425 w431 w454 w469 w506 w540 w571 w597 w621 w661 w673 w697 w725 w737 w763 w776 w843 w869 w882 w887 w893 w920 w928 w951 w956 w968 w977 w994 w1003 w1026 w1043 w1056 w1075 w1101 w1127 w1165 w1170 w1176 w1202 w1228 w1254 w1259 w1276 w1324 w1346 w1362 w1374 w1390 w1395 w1407 w1436 w1460 w1471 w1509 w1520 w1526 w1537 w1549 w1580 w1593 w1607 w1622 w1641 w1676 w1681 w1694 w1701 w1713 w1725 w1737 w1765 w1780 w1785 w1796 w1808 w1813 w1821 w1829 w1837 w1845 w1850 w1866 w1875 w1893 w1909 w1929 w1940 w1962 w1975 w1986 w1991 w1999 w2007 w2012 w2020 w2027 w2034 w2044 w2072 w2080 w2087 w2095 w2100 w2107 w2113 w2119 w2127 w2141 w2148 w2160 w2230 w2241 w2254 w2279 w2302 w2308 w2324 w2346 w2354 w2360 w2365 w2372 w2382 w2394 w2403 w2408 w2420 w2425 w2435 w2443 w2451 w2456 w2461 w2466 w2476 w2498 w2517 w2522 w2533 w2554 w2573 w2592 w2597 w2625 w2654 w2699 w2709 w2727 w2747 w2761 w2781 w2801 w2811 w2823 w2840 w2861 w2885 w2904 w2922 w2940 w2958 w2972 w2986 w3000 w3012 w3021 w3026] -> w78
      tunnel: [_ _ _ _ _ _ _ _ _ _ _ _ _ _ _ _ _ _ _ _ _ _ _ _ _ _ TRUE _ _ _ _ _ _ _ _ _ _ _ _ _ _ _ _ _ _ _ _ _ _ _ _ _ _ _ _ _ _ _ _ _ _ _ _ _ _ _ _ _ _ _ _ _ _ _ _ _ _ _ _ _ _ _ _ _ _ _ _ _ _ _ _ _ _ _ _ _ _ _ _ _ _ _ _ _ _ _ _ _ _ _ _ _ _ _ _ _ _ _ _ _ _ _ _ _ _ _ _ _ _ _ _ _ _ _ _ _ _ _ _ _ _ _ _ _ _ _ _ _ _ _ _ _ _ _ _ _ _ _ _ _ _ _ _ _ _ _ _ _ _ _] -> w69
      tunnel: [w87 w408 w416 w423 w429 w452 w467 w479 w538 w565 w588 w618 w658 w670 w689 w716 w735 w741 w774 w803 w857 w878 w885 w892 w919 w926 w950 w954 w960 w973 w993 w1002 w1017 w1041 w1046 w1067 w1093 w1121 w1163 w1168 w1174 w1181 w1208 w1234 w1257 w1270 w1316 w1344 w1349 w1372 w1389 w1393 w1398 w1426 w1451 w1469 w1489 w1519 w1524 w1534 w1546 w1564 w1589 w1600 w1618 w1635 w1660 w1679 w1692 w1696 w1711 w1723 w1735 w1754 w1770 w1783 w1795 w1807 w1811 w1817 w1824 w1834 w1842 w1848 w1855 w1874 w1882 w1903 w1912 w1936 w1961 w1970 w1985 w1989 w1994 w2002 w2010 w2019 w2025 w2032 w2042 w2070 w2078 w2085 w2093 w2098 w2106 w2112 w2117 w2122 w2139 w2147 w2157 w2228 w2239 w2250 w2274 w2300 w2306 w2319 w2343 w2352 w2358 w2363 w2370 w2378 w2391 w2401 w2406 w2418 w2423 w2429 w2441 w2449 w2454 w2459 w2464 w2474 w2497 w2516 w2520 w2532 w2553 w2572 w2591 w2595 w2608 w2651 w2697 w2706 w2723 w2743 w2757 w2780 w2798 w2805 w2818 w2836 w2857 w2881 w2900 w2918 w2936 w2954 w2968 w2982 w2996 w3010 w3020 w3024] -> w77
      tunnel: 30 ("Timeout") -> [w86 _ _ _ _ _ _ _ _ _ _ _ _ _ _ _ _ _ _ _ _ _ _ _ _ _ _ _ _ _ _ _ _ _ _ _ _ _ _ _ _ _ _ _ _ _ _ _ _ _ _ _ _ _ _ _ _ _ _ _ _ _ _ _ _ _ _ _ _ _ _ _ _ _ _ _ _ _ _ _ _ _ _ _ _ _ _ _ _ _ _ _ _ _ _ _ _ _ _ _ _ _ _ _ _ _ _ _ _ _ _ _ _ _ _ _ _ _ _ _ _ _ _ _ _ _ _ _ _ _ _ _ _ _ _ _ _ _ _ _ _ _ _ _ _ _ _ _ _ _ _ _ _ _ _ _ _ _ _ _ _ _ _ _ _ _ _ _ _ _]
      tunnel: w74 -> [_ _ _ _ _ _ _ _ _ w569 _ _ _ _ _ _ _ _ _ _ _ _ _ _ _ _ _ _ _ _ _ _ _ _ _ _ _ _ _ _ _ _ _ _ _ _ _ _ _ _ _ _ _ _ _ _ _ _ _ _ _ _ _ _ _ _ _ _ _ _ _ _ _ _ _ _ w1792 w1803 _ _ _ _ _ _ _ _ _ _ _ _ _ _ _ _ _ _ _ _ _ _ _ _ _ _ _ _ _ _ _ _ _ _ _ _ _ _ _ _ _ _ _ _ _ _ _ _ _ _ _ _ _ _ _ _ _ _ _ _ _ _ _ _ _ _ _ _ _ _ _ _ _ _ _ _ _ _ _ _ _ _ _ _ _ _ _ _ _ _ _ _]
      tunnel: w73 -> [_ _ _ _ _ _ _ _ _ w568 _ _ _ _ _ _ _ _ _ _ _ _ _ _ _ _ _ _ _ _ _ _ _ _ _ _ _ _ _ _ _ _ _ _ _ _ _ _ _ _ _ _ _ _ _ _ _ _ _ _ _ _ _ _ _ _ _ _ _ _ _ _ _ _ _ _ w1793 w1802 _ _ _ _ _ _ _ _ _ _ _ _ _ _ _ _ _ _ _ _ _ _ _ _ _ _ _ _ _ _ _ _ _ _ _ _ _ _ _ _ _ _ _ _ _ _ _ _ _ _ _ _ _ _ _ _ _ _ _ _ _ _ _ _ _ _ _ _ _ _ _ _ _ _ _ _ _ _ _ _ _ _ _ _ _ _ _ _ _ _ _ _]
      tunnel: w72 -> [w85 _ _ _ _ _ _ _ _ _ _ _ _ _ _ _ _ _ _ _ _ _ _ _ _ _ _ _ _ _ _ _ _ _ _ _ _ _ _ _ _ _ _ _ _ _ _ w1340 _ _ _ _ _ _ _ _ _ _ _ _ _ _ _ _ _ _ _ _ _ _ _ _ _ _ _ _ _ _ _ _ _ _ _ _ _ _ _ _ _ _ _ _ _ _ _ _ _ _ _ _ _ _ _ _ _ _ _ _ _ _ _ _ _ _ _ _ _ _ _ _ _ _ _ _ _ _ _ _ _ _ _ _ _ _ _ _ _ _ _ _ _ _ _ _ _ _ _ _ _ _ _ _ _ _ _ _ _ _ _ _ _ _ _ _ _ _ _ _ _ _]
      tunnel: w71 -> [w84 w407 w417 w422 w428 w444 w466 w490 w539 w570 w595 w620 w660 w671 w696 w724 w736 w762 w773 w842 w868 w877 w884 w889 w906 w925 w948 w953 w958 w970 w980 w996 w1025 w1040 w1054 w1073 w1099 w1117 w1161 w1167 w1173 w1180 w1207 w1233 w1256 w1261 w1289 w1345 w1361 w1371 w1376 w1392 w1406 w1435 w1459 w1463 w1508 w1511 w1523 w1530 w1539 w1551 w1582 w1598 w1612 w1632 w1647 w1678 w1693 w1700 w1712 w1724 w1736 w1764 w1767 w1782 w1794 w1801 w1810 w1819 w1827 w1831 w1839 w1847 w1865 w1868 w1880 w1898 w1913 w1932 w1958 w1974 w1984 w1988 w1996 w2004 w2009 w2017 w2024 w2031 w2041 w2069 w2077 w2084 w2089 w2097 w2104 w2110 w2116 w2124 w2134 w2143 w2154 w2227 w2240 w2252 w2276 w2296 w2304 w2317 w2345 w2350 w2356 w2362 w2369 w2380 w2392 w2400 w2405 w2417 w2422 w2433 w2440 w2448 w2453 w2458 w2463 w2473 w2496 w2515 w2519 w2531 w2552 w2571 w2590 w2594 w2605 w2653 w2694 w2708 w2726 w2746 w2760 w2779 w2799 w2806 w2822 w2839 w2860 w2884 w2903 w2921 w2939 w2957 w2971 w2985 w2999 w3009 w3019 w3023]
      tunnel: [w83 w407 w417 w422 w428 w444 w466 w490 w539 w570 w595 w620 w660 w671 w696 w724 w736 w762 w773 w842 w868 w877 w884 w889 w906 w925 w948 w953 w958 w970 w980 w996 w1025 w1040 w1054 w1073 w1099 w1117 w1161 w1167 w1173 w1180 w1207 w1233 w1256 w1261 w1289 w1345 w1361 w1371 w1376 w1392 w1406 w1435 w1459 w1463 w1508 w1511 w1523 w1530 w1539 w1551 w1582 w1598 w1612 w1632 w1647 w1678 w1693 w1700 w1712 w1724 w1736 w1764 w1767 w1782 w1794 w1801 w1810 w1819 w1827 w1831 w1839 w1847 w1865 w1868 w1880 w1898 w1913 w1932 w1958 w1974 w1984 w1988 w1996 w2004 w2009 w2017 w2024 w2031 w2041 w2069 w2077 w2084 w2089 w2097 w2104 w2110 w2116 w2124 w2134 w2143 w2154 w2227 w2240 w2252 w2276 w2296 w2304 w2317 w2345 w2350 w2356 w2362 w2369 w2380 w2392 w2400 w2405 w2417 w2422 w2433 w2440 w2448 w2453 w2458 w2463 w2473 w2496 w2515 w2519 w2531 w2552 w2571 w2590 w2594 w2605 w2653 w2694 w2708 w2726 w2746 w2760 w2779 w2799 w2806 w2822 w2839 w2860 w2884 w2903 w2921 w2939 w2957 w2971 w2985 w2999 w3009 w3019 w3023] -> w70
      tunnel: w66 -> [_ _ _ _ _ _ _ _ _ w563 _ _ _ _ _ _ _ _ _ _ _ _ _ _ _ _ _ _ _ _ _ _ _ _ _ _ _ _ _ _ _ _ _ _ _ _ _ _ _ _ _ _ _ _ _ _ _ _ _ _ _ _ _ _ _ _ _ _ _ _ _ _ _ _ _ _ w1789 w1800 _ _ _ _ _ _ _ _ _ _ _ _ _ _ _ _ _ _ _ _ _ _ _ _ _ _ _ _ _ _ _ _ _ _ _ _ _ _ _ _ _ _ _ _ _ _ _ _ _ _ _ _ _ _ _ _ _ _ _ _ _ _ _ _ _ _ _ _ _ _ _ _ _ _ _ _ _ _ _ _ _ _ _ _ _ _ _ _ _ _ _ _]
      frame "", "Event Structure", "Idle" {
        # "executes when the state queue is empty"
        n27 = event shown="[30] <AcqLoop error?>: User Event" {
          selector: w84 -> [_ _ _ _ _ _ _ _ _ _ _ _ _ _ _ _ _ _ _ _ _ _ _ _ _ _ _ _ _ _ _ _]
          dyn-events: [_ _ _ _ _ _ _ _ _ _ _ _ _ _ _ _ _ _ _ _ _ _ _ _ _ _ _ _ _ _ _ _] -> w83
          timeout: w86 -> [_ _ _ _ _ _ _ _ _ _ _ _ _ _ _ _ _ _ _ _ _ _ _ _ _ _ _ _ _ _ _ _]
          tunnel: w92 -> [w111 w122 w130 w134 w138 w146 w152 w160 w170 w177 w201 w217 w233 w237 w244 w265 w280 w295 w300 w303 w309 w316 w322 w329 w336 w347 w359 w366 w370 w374 w390 w406]
          tunnel: [w112 w122 w129 w134 w137 w146 w152 w160 w170 w176 w201 w217 w233 w237 w243 w265 w280 w295 w299 w302 w309 w317 w321 w329 w337 w347 w360 w366 w370 w373 w391 w405] -> w91
          tunnel: w90 -> [w93 w120 w124 w132 w139 w145 w153 w161 w168 w172 w199 w215 w231 w235 w239 w260 w279 w294 w296 w304 w307 w312 w324 w327 w331 w345 w355 w364 w368 w375 w388 w403]
          tunnel: [w110 w121 w125 w133 w140 w144 w151 w159 w169 w178 w200 w216 w232 w236 w245 w263 w268 w283 w298 w305 w308 w313 w325 w328 w335 w346 w356 w365 w369 w376 w392 w404] -> w89
          tunnel: w88 -> [w110 w121 w125 w133 w140 w144 w151 w159 w169 w178 w200 w216 w232 w236 w245 w258 w274 w288 w298 w305 w308 w313 w325 w328 w335 w346 w358 w365 w369 w376 w392 w404]
          tunnel: [w93 w120 w124 w132 w139 w145 w153 w161 w168 w173 w199 w215 w231 w235 w240 w260 w279 w294 w296 w304 w307 w314 w324 w327 w332 w345 w361 w364 w368 w375 w389 w403] -> w87
          tunnel: w85 -> [_ _ _ _ _ _ _ _ _ _ _ _ _ _ _ _ _ _ _ _ _ _ _ _ _ _ _ _ _ _ _ _]
          event Timeout {
            # "check system status every 2s"
            n28 = event-data() -> ()  [unwired: 1 in, 1 out]
            n29 = Unbundle By Name(w93) -> ("SysRunning?"=w100:bool, "SlowTimer"=w109:u32, "FastTimer"=w102:u32)
            n30 = Tick Count (ms)() -> (millisecond timer value=w94:u32)
            n31 = case shown="True" w100 {
              tunnel: ["" "Utility: AquiTimerCheck" ("State(s) in Front (\"\")")] -> w99
              frame False {
                # "if not running, do nothing"
              }
              frame True {
                # "if aquisition is running, check timer"
              }
            }
            n32 = Subtract(x=w94, y=w109) -> (x-y=w106:u32)
            n33 = Subtract(x=w94, y=w102) -> (x-y=w103:u32)
            n34 = Greater?(x=w106, y=u32 2000) -> (0:w107:bool)
            n35 = Greater?(x=w103, y=u32 500) -> (0:w104:bool)
            n36 = case shown="True" w107 {
              tunnel: ["" ("Empty String Constant") "SystemStatus: SlowSysStatusMacro" ("State(s) in Front (\"\")")] -> w97
              frame False {
              }
              frame True {
              }
            }
            n37 = case shown="True" w104 {
              tunnel: ["" ("Empty String Constant") "SystemStatus: FastSysStatusMacro" ("State(s) in Front (\"\")")] -> w95
              frame False {
              }
              frame True {
              }
            }
            n38 = call <vilib>:"Add State(s) to Queue__JKI_lib_State_Machine.vi"("State(s) in Front (\"\")"=w99, "State(s) in (\"\")"="LabJack: checkPedal" ("State(s) in Front (\"\")"), "State(s) at Back (\"\")"=w97) -> ("States Out"=w96:string)  [unwired: 12 in]
            n39 = call <vilib>:"Add State(s) to Queue__JKI_lib_State_Machine.vi"("State(s) in Front (\"\")"=w96, "State(s) in (\"\")"=w95) -> ("States Out"=w101:string)  [unwired: 13 in]
            n40 = call <vilib>:"Add State(s) to Queue__JKI_lib_State_Machine.vi"("State(s) in Front (\"\")"=w101, "State(s) in (\"\")"=w111) -> ("States Out"=w112:string)  [unwired: 13 in]
          }
          event "355nm Laser toggle": Mouse Enter {
            n41 = event-data() -> ()  [unwired: 1 in, 4 out]
            n42 = local write "Help"("Toggle 355nm laser." ("Help")) -> ()
          }
          event "355nm Laser toggle": Value Change {
            # "[Covers: REQ34]"
            n43 = event-data() -> ()  [unwired: 1 in, 6 out]
            n44 = Select(t="LabJack: 355_PWM_Start\nLabJack: AB_Start", s="355nm Laser toggle", f="LabJack: 355_PWM_Stop\nLabJack: AB_Stop") -> (s? t:f=w127:string)
            n45 = call <vilib>:"Add State(s) to Queue__JKI_lib_State_Machine.vi"("State(s) in Front (\"\")"=w127, "State(s) in (\"\")"=w130) -> ("States Out"=w129:string)  [unwired: 13 in]
          }
          event "Aiming beam toggle": Mouse Enter {
            n46 = event-data() -> ()  [unwired: 1 in, 4 out]
            n47 = local write "Help"("Toggle aiming beam laser." ("Help")) -> ()
          }
          event "Aiming beam toggle": Value Change {
            # "[Covers: REQ33]"
            n48 = event-data() -> ()  [unwired: 1 in, 6 out]
            n49 = case shown="True" "Aiming beam toggle" {
              tunnel: ["LabJack: AB_Stop" ("State(s) in Front (\"\")") "LabJack: AB_Start" ("State(s) in Front (\"\")")] -> w136
              frame False {
              }
              frame True {
              }
            }
            n50 = call <vilib>:"Add State(s) to Queue__JKI_lib_State_Machine.vi"("State(s) in Front (\"\")"=w136, "State(s) in (\"\")"=w138) -> ("States Out"=w137:string)  [unwired: 13 in]
          }
          event "Auto gain ch1": Value Change {
            n51 = event-data() -> ("NewVal"=w143:bool)  [unwired: 1 in, 5 out]
            n52 = case shown="True" w143 {
              frame False {
                n53 = local read "V 1"() -> (w147:dbl)
                n54 = call "V1FGV.vi"("action (write)"=enum16{"write", "read"}."write" ("action"), "V1 in"=w147) -> ()  [unwired: 8 in, 2 out]
                n55 = property on="V 1" class="DigNum (strict)"("DisabledEnum"=T8."Enabled" ("Disabled")) -> ()  [unwired: 2 in, 2 out]
              }
              frame True {
                n56 = property on="V 1" class="DigNum (strict)"("DisabledEnum"=T8."Disabled and Grayed Out" ("Disabled")) -> ()  [unwired: 2 in, 2 out]
              }
            }
          }
          event "Auto gain ch2": Value Change {
            n57 = event-data() -> ("NewVal"=w154:bool)  [unwired: 1 in, 5 out]
            n58 = case shown="False" w154 {
              frame False {
                n59 = local read "V 2"() -> (w155:dbl)
                n60 = property on="V 2" class="DigNum (strict)"("DisabledEnum"=T8."Enabled" ("Disabled")) -> ()  [unwired: 2 in, 2 out]
                n61 = call "V2FGV.vi"("action(write)"=enum16{"write", "read"}."write" ("action"), "V2 in"=w155) -> ()  [unwired: 8 in, 2 out]
              }
              frame True {
                n62 = property on="V 2" class="DigNum (strict)"("DisabledEnum"=T8."Disabled and Grayed Out" ("Disabled")) -> ()  [unwired: 2 in, 2 out]
              }
            }
          }
          event "Auto gain ch3": Value Change {
            n63 = event-data() -> ("NewVal"=w162:bool)  [unwired: 1 in, 5 out]
            n64 = case shown="False" w162 {
              frame False {
                n65 = local read "V 3"() -> (w163:dbl)
                n66 = property on="V 3" class="DigNum (strict)"("DisabledEnum"=T8."Enabled" ("Disabled")) -> ()  [unwired: 2 in, 2 out]
                n67 = call "V3FGV.vi"("action(write)"=enum16{"write", "read"}."write" ("action"), "V3 in"=w163) -> ()  [unwired: 8 in, 2 out]
              }
              frame True {
                n68 = property on="V 3" class="DigNum (strict)"("DisabledEnum"=T8."Disabled and Grayed Out" ("Disabled")) -> ()  [unwired: 2 in, 2 out]
              }
            }
          }
          event "Background": Mouse Enter {
            n69 = event-data() -> ()  [unwired: 1 in, 4 out]
            n70 = local write "Help"("Click to record a background." ("Help")) -> ()
          }
          event "Background": Value Change {
            n71 = event-data() -> ("NewVal"=w174:bool)  [unwired: 1 in, 5 out]
            n72 = case shown="False" w174 {
              tunnel: ["UI: Cursor Set >> Busy\nUtility: SetAllChanManualGain\nQueue: Flash\nUtility: Dewelling >> 2500\nLabJack: 355_PWM_Stop\nLabJack: AB_Stop" "Utility: SetDataClass >> Bg\nUI: Update\nLabJack: 355_PWM_Start\nLabJack: AB_Start\nUtility: SaveDeconChan\nUtility: Dewelling >> 50\nLabJack: SetV\nDigitizer: Start\nUtility: AquiTimerReset\nLED: BreathGreen\nUI: duringBGAcquire"] -> w175
              tunnel: [FALSE TRUE] -> w171
              frame False {
                n73 = property on="Background" class="Bool (strict)"("BoolText.Text"="Done!" ("Boolean Text.Text")) -> ()  [unwired: 2 in, 2 out]
              }
              frame True {
                # "[Covers: REQ6]"
                n74 = property on="Background" class="Bool (strict)"("BoolText.Text"="Running" ("Boolean Text.Text"), "Colors [4]"=cluster{u32, u32}[] [{6618880, 6618880}, {16711680, 16711680}]) -> ()  [unwired: 2 in, 2 out]
              }
            }
            n75 = Bundle By Name(cluster=w172, "SysRunning?"=w171) -> (w173:T20)
            n76 = call <vilib>:"Add State(s) to Queue__JKI_lib_State_Machine.vi"("State(s) in Front (\"\")"=w175, "State(s) in (\"\")"=w177) -> ("States Out"=w176:string)  [unwired: 13 in]
          }
          event "Channel 1": Cursor Move {
            n77 = event-data() -> ("CursIdx"=w190:i32, "CursLoc"=w197:cluster{"X":dbl, "Y":dbl})  [unwired: 1 in, 7 out]
            n78 = Unbundle By Name(w197) -> ("X"=w195:dbl)
            n79 = property on="Channel 2" class="WFGraph (strict)"() -> ("CrsrList"=w194:T21)  [unwired: 2 in, 2 out]
            n80 = property on="Channel 3" class="WFGraph (strict)"() -> ("CrsrList"=w191:T21)  [unwired: 2 in, 2 out]
            n81 = Index Array(array=w194, index=w190) -> (element=w198:T22)
            n82 = Index Array(array=w191, index=w190) -> (element=w196:T22)
            n83 = Bundle By Name(cluster=w196, "Position.X"=w195) -> (w189:T22)
            n84 = Bundle By Name(cluster=w198, "Position.X"=w195) -> (w193:T22)
            n85 = control-ref of="Channel 1"() -> (w186:refnum<vi>)
            n86 = Replace Array Subset(array=w194, new element=w193, index=w190) -> (w192:T21)
            n87 = Replace Array Subset(array=w191, new element=w189, index=w190) -> (w188:T21)
            n88 = property on="Channel 2" class="WFGraph (strict)"("CrsrList"=w192) -> ()  [unwired: 2 in, 2 out]
            n89 = property on="Channel 3" class="WFGraph (strict)"("CrsrList"=w188) -> (error out=w187:errorcluster)  [unwired: 2 in, 1 out]
            n90 = call "UpdateCurserIdx(SubVI).vi"("error in (no error)"=w187, "WaveformGraph in"=w186) -> ()  [unwired: 9 in, 1 out]
          }
          event "Channel 2": Cursor Move {
            n91 = event-data() -> ("CursIdx"=w208:i32, "CursLoc"=w214:cluster{"X":dbl, "Y":dbl})  [unwired: 1 in, 7 out]
            n92 = Unbundle By Name(w214) -> ("X"=w211:dbl)
            n93 = property on="Channel 1" class="WFGraph (strict)"() -> ("CrsrList"=w206:T21)  [unwired: 2 in, 2 out]
            n94 = property on="Channel 3" class="WFGraph (strict)"() -> ("CrsrList"=w209:T21)  [unwired: 2 in, 2 out]
            n95 = Index Array(array=w206, index=w208) -> (element=w213:T22)
            n96 = Index Array(array=w209, index=w208) -> (element=w212:T22)
            n97 = Bundle By Name(cluster=w213, "Position.X"=w211) -> (w210:T22)
            n98 = Bundle By Name(cluster=w212, "Position.X"=w211) -> (w207:T22)
            n99 = Replace Array Subset(array=w206, new element=w210, index=w208) -> (w205:T21)
            n100 = Replace Array Subset(array=w209, new element=w207, index=w208) -> (w204:T21)
            n101 = control-ref of="Channel 1"() -> (w203:refnum<vi>)
            n102 = property on="Channel 1" class="WFGraph (strict)"("CrsrList"=w205) -> ()  [unwired: 2 in, 2 out]
            n103 = property on="Channel 3" class="WFGraph (strict)"("CrsrList"=w204) -> (error out=w202:errorcluster)  [unwired: 2 in, 1 out]
            n104 = call "UpdateCurserIdx(SubVI).vi"("error in (no error)"=w202, "WaveformGraph in"=w203) -> ()  [unwired: 9 in, 1 out]
          }
          event "Channel 3": Cursor Move {
            n105 = event-data() -> ("CursIdx"=w223:i32, "CursLoc"=w230:cluster{"X":dbl, "Y":dbl})  [unwired: 1 in, 7 out]
            n106 = Unbundle By Name(w230) -> ("X"=w227:dbl)
            n107 = property on="Channel 1" class="WFGraph (strict)"() -> ("CrsrList"=w226:T21)  [unwired: 2 in, 2 out]
            n108 = property on="Channel 2" class="WFGraph (strict)"() -> ("CrsrList"=w224:T21)  [unwired: 2 in, 2 out]
            n109 = Index Array(array=w226, index=w223) -> (element=w229:T22)
            n110 = Index Array(array=w224, index=w223) -> (element=w228:T22)
            n111 = Bundle By Name(cluster=w229, "Position.X"=w227) -> (w225:T22)
            n112 = Bundle By Name(cluster=w228, "Position.X"=w227) -> (w222:T22)
            n113 = Replace Array Subset(array=w226, new element=w225, index=w223) -> (w221:T21)
            n114 = Replace Array Subset(array=w224, new element=w222, index=w223) -> (w220:T21)
            n115 = control-ref of="Channel 1"() -> (w218:refnum<vi>)
            n116 = property on="Channel 1" class="WFGraph (strict)"("CrsrList"=w221) -> ()  [unwired: 2 in, 2 out]
            n117 = property on="Channel 2" class="WFGraph (strict)"("CrsrList"=w220) -> (error out=w219:errorcluster)  [unwired: 2 in, 1 out]
            n118 = call "UpdateCurserIdx(SubVI).vi"("error in (no error)"=w219, "WaveformGraph in"=w218) -> ()  [unwired: 9 in, 1 out]
          }
          event "Cali&iRF alignment": Mouse Enter {
            n119 = event-data() -> ()  [unwired: 1 in, 4 out]
            n120 = local write "Help"("Click to run system intensity calibration and irf alignment" ("Help")) -> ()
          }
          event "Cali&iRF alignment": Value Change {
            n121 = event-data() -> ("NewVal"=w241:bool)  [unwired: 1 in, 5 out]
            n122 = case shown="False" w241 {
              tunnel: ["UI: Cursor Set >> Busy\nUtility: SetAllChanManualGain\nQueue: Flash\nUtility: Dewelling >> 1500\nLabJack: 355_PWM_Stop\nLabJack: AB_Stop" "Utility: SetDataClass >> Cali\nUI: Update\nUtility: SaveDeconChan\nLabJack: 355_PWM_Start\nLabJack: AB_Start\nLabJack: SetV\nDigitizer: Start\nUtility: AquiTimerReset\nLED: BreathGreen\nUI: duringIRFAlign"] -> w242
              tunnel: [FALSE TRUE] -> w238
              frame False {
                n123 = property on="Cali&iRF alignment" class="Bool (strict)"("BoolText.Text"="Done!" ("Boolean Text.Text")) -> ()  [unwired: 2 in, 2 out]
              }
              frame True {
                n124 = property on="Cali&iRF alignment" class="Bool (strict)"("BoolText.Text"="Running" ("Boolean Text.Text"), "Colors [4]"=cluster{u32, u32}[] [{6618880, 6618880}, {16711680, 16711680}]) -> ()  [unwired: 2 in, 2 out]
              }
            }
            n125 = Bundle By Name(cluster=w239, "SysRunning?"=w238) -> (w240:T20)
            n126 = call <vilib>:"Add State(s) to Queue__JKI_lib_State_Machine.vi"("State(s) in Front (\"\")"=w242, "State(s) in (\"\")"=w244) -> ("States Out"=w243:string)  [unwired: 13 in]
          }
          event "V 1": Value Change {
            n127 = event-data() -> ()  [unwired: 1 in, 6 out]
            n128 = call "LabJack_FGV.vi"("Operation(Read)"=enum16{"Write", "Read"}."Read" ("Operation"), "error in (no error)"=w258) -> ("error out"=w254:errorcluster, "Read data"=w255:i32)  [unwired: 8 in]
            n129 = global read "GlobalVariables.vi" "Ch1 LJ pin"() -> (w257:string)
            n130 = call "LJM_eWriteName.vi"("Handle In"=w255, "Name"=w257, "Value"="V 1", "error in"=w254) -> ("error out"=w253:errorcluster)  [unwired: 10 in, 1 out]
            n131 = call "V1FGV.vi"("Error In"=w253, "action (write)"=enum16{"write", "read"}."write" ("action"), "V1 in"="V 1") -> ()  [unwired: 7 in, 2 out]
            n132 = call "CtrlVtoGain.vi"("error in (no error)"=w253, "CtrlV(V)"="V 1", "Channel"=enum16{"Ch1", "Ch2", "Ch3"}."Ch1" ("Enum")) -> ("error out"=w263:errorcluster, "Gain"=w262:dbl)  [unwired: 7 in]
            n133 = local write "Gain1"(w262) -> ()
          }
          event "V 2": Value Change {
            n134 = event-data() -> ()  [unwired: 1 in, 6 out]
            n135 = call "LabJack_FGV.vi"("Operation(Read)"=enum16{"Write", "Read"}."Read" ("Operation"), "error in (no error)"=w274) -> ("error out"=w270:errorcluster, "Read data"=w272:i32)  [unwired: 8 in]
            n136 = global read "GlobalVariables.vi" "Ch2 LJ pin"() -> (w273:string)
            n137 = call "LJM_eWriteName.vi"("Handle In"=w272, "Name"=w273, "Value"="V 2", "error in"=w270) -> ("error out"=w269:errorcluster)  [unwired: 10 in, 1 out]
            n138 = call "V2FGV.vi"("Error In"=w269, "action(write)"=enum16{"write", "read"}."write" ("action"), "V2 in"="V 2") -> ("Error Out"=w267:errorcluster)  [unwired: 7 in, 1 out]
            n139 = call "CtrlVtoGain.vi"("error in (no error)"=w269, "CtrlV(V)"="V 2", "Channel"=enum16{"Ch1", "Ch2", "Ch3"}."Ch2" ("Enum")) -> ("error out"=w266:errorcluster, "Gain"=w276:dbl)  [unwired: 7 in]
            n140 = local write "Gain2"(w276) -> ()
            n141 = Merge Errors(w267, w266) -> (w268:errorcluster)
          }
          event "V 3": Value Change {
            n142 = event-data() -> ()  [unwired: 1 in, 6 out]
            n143 = call "LabJack_FGV.vi"("Operation(Read)"=enum16{"Write", "Read"}."Read" ("Operation"), "error in (no error)"=w288) -> ("error out"=w289:errorcluster, "Read data"=w286:i32)  [unwired: 8 in]
            n144 = global read "GlobalVariables.vi" "Ch3 LJ pin"() -> (w287:string)
            n145 = call "LJM_eWriteName.vi"("Handle In"=w286, "Name"=w287, "Value"="V 3", "error in"=w289) -> ("error out"=w284:errorcluster)  [unwired: 10 in, 1 out]
            n146 = call "V3FGV.vi"("Error In"=w284, "action(write)"=enum16{"write", "read"}."write" ("action"), "V3 in"="V 3") -> ("Error Out"=w282:errorcluster)  [unwired: 7 in, 1 out]
            n147 = call "CtrlVtoGain.vi"("error in (no error)"=w284, "CtrlV(V)"="V 3", "Channel"=enum16{"Ch1", "Ch2", "Ch3"}."Ch3" ("Enum")) -> ("error out"=w281:errorcluster, "Gain"=w291:dbl)  [unwired: 7 in]
            n148 = local write "Gain3"(w291) -> ()
            n149 = Merge Errors(w282, w281) -> (w283:errorcluster)
          }
          event "Quit": Value Change {
            # "Exit Button Value Change (pressed) Event\n(when pressed.  quite)"
            n150 = event-data() -> ()  [unwired: 1 in, 1 out]
            n151 = call <vilib>:"Add State(s) to Queue__JKI_lib_State_Machine.vi"("State(s) in Front (\"\")"="LED: Off\nMacro: Exit", "State(s) in (\"\")"=w300) -> ("States Out"=w299:string)  [unwired: 13 in]
          }
          event "Show BG": Value Change {
            n152 = event-data() -> ()  [unwired: 1 in, 6 out]
            n153 = call <vilib>:"Add State(s) to Queue__JKI_lib_State_Machine.vi"("State(s) in Front (\"\")"="Data: showBG" ("State(s) in Front (\"\")"), "State(s) in (\"\")"=w303) -> ("States Out"=w302:string)  [unwired: 13 in]
          }
          event "StartButton": Mouse Enter {
            n154 = event-data() -> ()  [unwired: 1 in, 4 out]
            n155 = local write "Help"("Press to start aquisition." ("Help")) -> ()
          }
          event "StartButton": Value Change {
            # "[Covers: REQ32]"
            # "start PWM before acquisition"
            # "Initialize both digitizer aquisition and\n send user event to trigger aquisition loop"
            n156 = event-data() -> ()  [unwired: 1 in, 6 out]
            n157 = local write "StartButton"(FALSE ("StartButton")) -> ()
            n158 = Bundle By Name(cluster=w312, "SysRunning?"=TRUE) -> (w314:T20)
            n159 = call <vilib>:"Add State(s) to Queue__JKI_lib_State_Machine.vi"("State(s) in Front (\"\")"="TCP: stopCam\nUtility: SetDataClass >> Data\nQueue: Flash\nUI: Update\nUtility: StartBeep\nLabJack: 355_PWM_Start\nLabJack: AB_Start\nLabJack: SetV\nDigitizer: Start\nUtility: AquiTimerReset\nUI: DuringAquisition\nLED: BreathGreen\nTCP: sendRunNum\nTCP: sendVideoSource\nTCP: startRun", "State(s) in (\"\")"=w316) -> ("States Out"=w317:string)  [unwired: 13 in]
          }
          event "Video Display": Value Change {
            n160 = event-data() -> ("NewVal"=w323:bool)  [unwired: 1 in, 5 out]
            n161 = Select(t="TCP: startCam", s=w323, f="TCP: stopCam") -> (s? t:f=w320:string)
            n162 = call <vilib>:"Add State(s) to Queue__JKI_lib_State_Machine.vi"("State(s) in (\"\")"=w322, "State(s) at Back (\"\")"=w320) -> ("States Out"=w321:string)  [unwired: 13 in]
          }
          event "StopButton": Mouse Enter {
            n163 = event-data() -> ()  [unwired: 1 in, 4 out]
            n164 = local write "Help"("Press to stop data aquisition." ("Help")) -> ()
          }
          event "StopButton": Value Change {
            # "if system is running, send stop command, if not do nothing."
            # "stop aquisition\nupdate UI"
            n165 = event-data() -> ()  [unwired: 1 in, 6 out]
            n166 = Unbundle By Name(w331) -> ("SysRunning?"=w333:bool)
            n167 = case shown="True" w333 {
              tunnel: ["" ("Empty String Constant") "LabJack: AB_Stop\nLabJack: 355_PWM_Stop\n/*Digitizer: Abort"] -> w334
              tunnel: w331 -> [w338 w342]
              tunnel: [w338 w341] -> w332
              frame False {
              }
              frame True {
                n168 = Bundle By Name(cluster=w342, "SysRunning?"=FALSE) -> (w341:T20)
              }
            }
            n169 = call <vilib>:"Add State(s) to Queue__JKI_lib_State_Machine.vi"("State(s) in Front (\"\")"=w334, "State(s) in (\"\")"=w336) -> ("States Out"=w337:string)  [unwired: 13 in]
            n170 = local write "StopButton"(FALSE ("StopButton")) -> ()
          }
          event "Sys Reconfig": Mouse Enter {
            n171 = event-data() -> ()  [unwired: 1 in, 4 out]
            n172 = local write "Help"("Click to reconfig digitizer settings." ("Help")) -> ()
          }
          event "Sys Reconfig": Value Change {
            # "everytime the user change data aquisition setting, need to reinitilize decon engine and realign iRF.\ncheck whether data length has changed, if changed, reinitialize Decon engine\nreset BG ready, need a new BG"
            # "update DAQ FGV"
            n173 = event-data() -> ()  [unwired: 1 in, 6 out]
            n174 = call "SystemConfigEditorV6.vi"("error in"=w358) -> ("error out"=w357:errorcluster, "FLImDAQ out"=w352:T5)  [unwired: 1 in]
            n175 = Unbundle By Name(w355) -> ("FLImDAQ.min record length"=w354:i32)
            n176 = Unbundle By Name(w352) -> ("min record length"=w353:i32)
            n177 = call "FLImDAQ_FGV.vi"("error in (no error)"=w357, "Operation (Read)"=enum16{"Write", "Read"}."Write" ("Operation"), "Write data"=w352) -> ("error out"=w356:errorcluster, "Read data"=w351:T5)  [unwired: 7 in]
            n178 = Equal?(x=w354, y=w353) -> (x = y?=w350:bool)
            n179 = case shown="False" w350 {
              tunnel: ["UI: Cursor Set >> Busy\nDigitizer: Config\nDeconEngine: InitializeCh1\nDeconEngine: InitializeCh2\nDeconEngine: InitializeCh3\nUI: CaliAndiRFNotReady\n/*UI iRF not ready\nUI: Update\nUI: Cursor Set >> Idle" "UI: Cursor Set >> Busy\nDigitizer: Config\nUI: Update\nUI: Cursor Set >> Idle"] -> w349
              frame False {
              }
              frame True {
              }
            }
            n180 = Bundle By Name(cluster=w355, "FLImDAQ"=w351) -> (w361:T20)
            n181 = call <vilib>:"Add State(s) to Queue__JKI_lib_State_Machine.vi"("State(s) in Front (\"\")"=w349, "State(s) in (\"\")"=w359) -> ("States Out"=w360:string)  [unwired: 13 in]
          }
          event "System Hardware Connection Status", "StartButton", "StopButton", "355nm Laser toggle", "Aiming beam toggle", "Cali&iRF alignment", "Background", "Sys Reconfig": Mouse Leave {
            n182 = event-data() -> ()  [unwired: 1 in, 4 out]
            n183 = invoke on="Help" class="Str" method="Reinit To Default"() -> ()  [unwired: 3 in, 3 out]
          }
          event "System Hardware Connection Status.Digitizer": Mouse Enter {
            n184 = event-data() -> ()  [unwired: 1 in, 4 out]
            n185 = local write "Help"("Status of hardware connections. TCP/IP is optional." ("Help")) -> ()
          }
          event "TCP Connect": Value Change {
            n186 = event-data() -> ("NewVal"=w371:bool)  [unwired: 1 in, 5 out]
            n187 = case shown="True" w371 {
              tunnel: ["TCP: Close\nUI: Update" ("State(s) in Front (\"\")") "TCP: Initialize\nTCP: SendSettingMacro\nUI: Update" ("State(s) in Front (\"\")")] -> w372
              frame False {
              }
              frame True {
              }
            }
            n188 = call <vilib>:"Add State(s) to Queue__JKI_lib_State_Machine.vi"("State(s) in Front (\"\")"=w372, "State(s) in (\"\")"=w374) -> ("States Out"=w373:string)  [unwired: 13 in]
          }
          event User Event {
            # "if aquisition loop is error out. Stop digitizer, update front panel indicator, stop both laser and \nOption 1: parse and save data\nOption 2: Flash queue if scout run. [Covers: REQ23]"
            n189 = event-data() -> ()  [unwired: 1 in, 5 out]
            n190 = case shown="\"Cali\"" "Data Class" {
              tunnel: [w396 "Utility: SetAllChanAutoGain\nUtility: RestoreDeConChan\nUI: Cursor Set >> Idle\nData: parseRunData\nData: irfAlignment" "Utility: SetAllChanAutoGain\nUtility: RestoreDeConChan\nUI: Cursor Set >> Idle\nData: parseRunData\nData: saveBGtoFGV\nData: saveBGtoFile\nData: showBG\nRun: BGIncrement"] -> w386
              frame "Data", Default {
                n191 = local read "Video Display"() -> (w398:bool)
                n192 = Select(t="TCP: startCam", s=w398, f="") -> (s? t:f=w394:string)
                n193 = call <vilib>:"Add State(s) to Queue__JKI_lib_State_Machine.vi"("State(s) in Front (\"\")"="TCP: stopRun\nUI: Cursor Set >> Busy\nData: parseRunData\nData: saveRunData\nUI: Cursor Set>>Idle" ("State(s) in Front (\"\")"), "State(s) in (\"\")"=w394) -> ("States Out"=w396:string)  [unwired: 13 in]
              }
              frame "Cali" {
              }
              frame "BG" {
              }
            }
            n194 = Bundle By Name(cluster=w388, "SysRunning?"=FALSE) -> (w389:T20)
            n195 = Select(t="" ("State(s) in Front (\"\")"), s="Skip Data Save?", f=w386) -> (s? t:f=w383:string)
            n196 = call <vilib>:"Add State(s) to Queue__JKI_lib_State_Machine.vi"("State(s) in Front (\"\")"="UI: Update\nLabJack: AB_Stop\nLabJack: 355_PWM_Stop\nDigitizer: Abort\nLabJack: ZeroV\nUtility: EndBeep\nLED: BreathOff" ("State(s) in Front (\"\")"), "State(s) in (\"\")"=w383, "State(s) at Back (\"\")"="Macro: SysReadyForAq\nUI: Update" ("State(s) in Front (\"\")")) -> ("States Out"=w381:string)  [unwired: 12 in]
            n197 = call <vilib>:"Add State(s) to Queue__JKI_lib_State_Machine.vi"("State(s) in Front (\"\")"=w381, "State(s) in (\"\")"=w390) -> ("States Out"=w391:string)  [unwired: 13 in]
          }
          event Panel Close? {
            # "Discard the event because we'll close the front panel ourselves in Macro: Exit"
            # "Close Panel button (pressed) Event\n(this executes Macro: Exit to terminate the VI)"
            n198 = event-data() -> ()  [unwired: 1 in, 1 out]
            n199 = event-data ("Event Filter Node")("Discard?"=TRUE) -> ()  [unwired: 1 in, 1 out]
            n200 = call <vilib>:"Add State(s) to Queue__JKI_lib_State_Machine.vi"("State(s) in Front (\"\")"="Macro: Exit", "State(s) in (\"\")"=w406) -> ("States Out"=w405:string)  [unwired: 13 in]
          }
        }
      }
      frame "---------- Macro ----------" {
        # "Do not put any code in this frame.\n(It is a separator no-op. You can make a copy of this frame to create a new Macro frame)"
        n201 = call <vilib>:"Add State(s) to Queue__JKI_lib_State_Machine.vi"("State(s) in (\"\")"=w411) -> ("States Out"=w410:string)  [unwired: 14 in]
      }
      frame "Macro: Initialize" {
        # "load Labjack setting 1st as it contaisn laser pin infortmation"
        # "start laser 1st, need 7.5s for laser to get ready"
        # "Initialization Macro\n(This is called once, when the VI starts)"
        n202 = call <vilib>:"Add State(s) to Queue__JKI_lib_State_Machine.vi"("State(s) in Front (\"\")"="UI: showDisclaimer\nUI: Cursor Set >> Busy\nData: Initialize\nInitialize Core Data\nUI: Initialize\nUI: Front Panel State >> Open\nUI: Update\nMacro: LoadSysConfig\nLabJack: Open\nLabJack: SetDefaultSub\nLED: OpenVIRef\nLED: BreathOrange\nUI: Update\n355 Laser: CheckControllerStatus\n355 Laser: Laser enable\n355 Laser: Dewelling>>500\n355 Laser: CheckControllerStatus\nUI: Update\nLabJack: 355_PWM_Config\nLabJack: AB_PWM_Config\n/*TCP: Initialize\n/*TCP: SyncTime\nUI: Update\n", "State(s) in (\"\")"="Digitizer: Initialize\nDigitizer: Config\nUI: Update\nAimingBeam: Initialize\nAimingBeam: Set Status>>Enable\nAimingBeam: Set Current\nUI: Update\n355 Laser: Check Dewelling\nUI: Cursor Set >> Idle\nCase: GetID\nUI: Update\nTCP: SendSettingMacro\nCase: CreatFileStruct\nUI: Update\nData: loadLastUseMacro\nDeconEngine: InitilizeMacro\nGraph: SetXMultiplier\nGraph: AddCursors\nAPD: Initialize\nAPD: LoadFromSerial\nAPD: UpdateCtrlVLimit\nAPD: GetGainLimits\nPID: loadPID\nLED: BreathOff\nMacro: SysReadyForAq") -> ("States Out"=w412:string)  [unwired: 13 in]
        n203 = call <vilib>:"Add State(s) to Queue__JKI_lib_State_Machine.vi"("State(s) in Front (\"\")"=w412, "State(s) in (\"\")"=w420) -> ("States Out"=w419:string)  [unwired: 13 in]
        "Help" <- "Hover over controls to see help!" ("Help")
      }
      frame "Macro: LoadSysConfig" {
        # "System configuration Macro. [Covers: REQ15]\n(Load configurations for different component of the system)"
        n204 = call <vilib>:"Add State(s) to Queue__JKI_lib_State_Machine.vi"("State(s) in Front (\"\")"="SysConfig: Load Sys Config\nSysConfig: Load Digitizer Setting\nSysConfig: Load AB setting\nSysConfig: Load LJ Pinout\nSysConfig: Load 355 PWM\nSysConfig: LoadAPDSerialNumber\nSysConfig: LoadABVideoSetting\nSysConfig: LoadCursorLocation", "State(s) in (\"\")"=w426) -> ("States Out"=w425:string)  [unwired: 13 in]
      }
      frame "Macro: SysReadyForAq" {
        # "Macro for system ready\n(It is a separator no-op. You can make a copy of this frame to create a new Macro frame)"
        n205 = call <vilib>:"Add State(s) to Queue__JKI_lib_State_Machine.vi"("State(s) in Front (\"\")"="UI: ReadyForAquisition\nLED: Green" ("State(s) in Front (\"\")"), "State(s) in (\"\")"=w432) -> ("States Out"=w431:string)  [unwired: 13 in]
      }
      frame "Macro: Exit" {
        # "close LJ last"
        # "check whether hardware is initilized, if so close, if not do nothing"
        # "Exit Macro, close all hardware\n(This is called once, when the VI exits)"
        n206 = Unbundle By Name(w452) -> ("System Status.TCP/IP"=w440:bool, "System Status.Digitizer"=w448:bool, "System Status.Aiming Beam"=w447:bool, "System Status.355 Laser"=w446:bool, "System Status.Labjack"=w436:bool, "Core.Close Panel on Exit?"=w441:bool)
        n207 = case shown="True" w448 {
          tunnel: ["" ("Empty String Constant") "Digitizer: Close"] -> w443
          frame False {
          }
          frame True {
          }
        }
        n208 = case shown="True" w440 {
          tunnel: ["" ("Empty String Constant") "TCP: Close"] -> w442
          frame False {
          }
          frame True {
          }
        }
        n209 = case shown="True" w436 {
          tunnel: ["" ("Empty String Constant") "LabJack: SetDefaultAndClose"] -> w433
          frame False {
          }
          frame True {
          }
        }
        n210 = case shown="True" w447 {
          tunnel: ["" ("Empty String Constant") "AimingBeam: Set Status >> Disable\nAimingBeam: Close"] -> w435
          frame False {
          }
          frame True {
          }
        }
        n211 = case shown="True" w446 {
          tunnel: ["" ("Empty String Constant") "355 Laser: Close\n355 Laser: CheckControllerStatus"] -> w434
          frame False {
          }
          frame True {
          }
        }
        n212 = Select(t="UI: Front Panel State >> Close", s=w441, f="" ("Empty String Constant")) -> (s? t:f=w437:string)
        n213 = call <vilib>:"Add State(s) to Queue__JKI_lib_State_Machine.vi"("State(s) in Front (\"\")"=w442, "State(s) in (\"\")"=w443, "State(s) at Back (\"\")"=w435) -> ("States Out"=w445:string)  [unwired: 12 in]
        n214 = call <vilib>:"Add State(s) to Queue__JKI_lib_State_Machine.vi"("State(s) in Front (\"\")"=w445, "State(s) in (\"\")"=w434, "State(s) at Back (\"\")"=w433) -> ("States Out"=w439:string)  [unwired: 12 in]
        n215 = call <vilib>:"Add State(s) to Queue__JKI_lib_State_Machine.vi"("State(s) in Front (\"\")"=w439, "State(s) in (\"\")"="UI: Update\nUI: Reset\nGraph: SaveCursorLoc\nLED: CloseVIRef\nQueue: Destory\nData: Cleanup\nExit", "State(s) at Back (\"\")"=w437) -> ("States Out"=w449:string)  [unwired: 12 in]
        n216 = call <vilib>:"Add State(s) to Queue__JKI_lib_State_Machine.vi"("State(s) in Front (\"\")"=w449, "State(s) in (\"\")"=w455) -> ("States Out"=w454:string)  [unwired: 13 in]
      }
      frame "---------- Data ----------" {
        # "Do not put any code in this frame.\n(It is a separator no-op. You can make a copy of this frame to create a new Data frame)"
        n217 = call <vilib>:"Add State(s) to Queue__JKI_lib_State_Machine.vi"("State(s) in (\"\")"=w470) -> ("States Out"=w469:string)  [unwired: 14 in]
      }
      frame "Data: Initialize" {
        w471 = path ""  # CaliPath
        w472 = T19 {"DeCon Channel"=enum."1", "Scale Bar"=FALSE, "Scale Low"=3.0, "Scale High"=8.0, "ANSI"=20.0, "Radius"=1.0, "3D?"=FALSE, "Firefly?"=FALSE, "Pentero?"=FALSE}  # VideoConfig
        w473 = T23 {"Ch1APDSerial#"="", "Ch2APDSerial#"="", "Ch3APDSerial#"=""}  # APDSerialNum
        w474 = u32 0  # Aquisition Timer
        w475 = cluster{"RunID":i8, "BG ID":i8, "Cali ID":i8} {"RunID"=1, "BG ID"=1, "Cali ID"=1}  # IDs
        w476 = refnum<vi> refnum  # LED vi reference
        w477 = path ""  # TempPath
        w478 = T24 {"DataPath"=path "", "BG Path"=path "", "iRFPath"=path "", "CaliPath"=path ""}  # Pathes
        w480 = dbl[] []  # V3
        w481 = dbl[] []  # V2
        w482 = dbl[] []  # V1
        w484 = u32 0  # FastTimer
        w485 = u32 0  # SlowTimer
        w486 = dbl[][] []  # Ch3Data
        w487 = dbl[][] []  # Ch2Data
        w488 = dbl[][] []  # Ch1Data
        w491 = T1 {"Digitizer"=FALSE, "Labjack"=FALSE, "Aiming Beam"=FALSE, "355 Laser"=FALSE, "TCP/IP"=FALSE}  # System Status
        w492 = T25 {"DIO_EF_CLOCK1_DIVISOR"=16, "DIO_EF_CLOCK1_ROLL_VALUE"=25000, "DIO#_EF_INDEX"=0, "DIO#_EF_OPTIONS"=1, "DIO#_EF_CONFIG_A"=6250}  # AB PWM setting
        w493 = T4 {"Ch1 Bias"="TDA11", "Ch2 Bias"="DAC10", "Ch3 Bias"="DAC0", "Ch4 Bias"="DAC0", "355 PWM"="FIO0", "AimingBeam PWM"="FIO2", "Laser Ready"="FIO3", "Interlock"="FIO1", "Laser Start/Stop"="FIO1", "Red LED"="FIO1", "Green LED"="FIO1", "Foot Pedal"="DIO15"}  # LJ Pinout
        w494 = 0  # TCP attempt count
        w495 = u32 0  # Laser start tic
        w496 = refnum<k20>[] []  # niTClk sessions
        w497 = u32 0  # Last Trigger
        w498 = T25 {"DIO_EF_CLOCK1_DIVISOR"=16, "DIO_EF_CLOCK1_ROLL_VALUE"=25000, "DIO#_EF_INDEX"=0, "DIO#_EF_OPTIONS"=1, "DIO#_EF_CONFIG_A"=6250}  # 355 PWM setting
        w499 = T26 {"Aiming Beam COM Port"="COM3", "Min Current"=0.0, "Max Current"=63.0, "Default Current"=20.0, "Freq"=0}  # AB Cluster
        w500 = T27 {"resource name"="", "resource name 2"="", "Channel"=enum."Channel 0", "trigger source"="VAL_EXTERNAL", "trigger level"=0.5, "trigger delay"=1.35e-07, "min sample rate"=12500000000.0, "min record length"=2500, "vertical range"=1.0, "vertical offset"=-0.25, "Waveform to Avg"=2000}  # FLImDAQ
        w501 = FALSE  # SysRunning?
        w489 = path ""  # DefaultPath
        w502 = ""  # CaseID
        w503 = T3 {"Ch1Enable?"=FALSE, "Ch2Enable?"=FALSE, "Ch3Enable?"=FALSE, "Ch1AutoGain?"=FALSE, "Ch2AutoGain?"=FALSE, "Ch3AutoGain?"=FALSE, "AimingBeamEnable?"=FALSE}  # SysConfigCluster
        w504 = T28 {"Current VI Reference"=refnum, "Close Panel on Exit?"=FALSE}  # Core
        # "Initialize the shift-register data, here.\n(data names are defined by what you wire into the bundle function)"
        n218 = Bundle("Core"=w504, "SysConfigCluster"=w503, "System Status"=w491, "IDs"=w475, "CaseID"=w502, "DefaultPath"=w489, "Pathes"=w478, "FLImDAQ"=w500, "SysRunning?"=w501, "AB Cluster"=w499, "LJ Pinout"=w493, "355 PWM setting"=w498, "AB PWM setting"=w492, "Last Trigger"=w497, "niTClk sessions"=w496, "Laser start tic"=w495, "TCP attempt count"=w494, "Ch1Data"=w488, "Ch2Data"=w487, "Ch3Data"=w486, "V1"=w482, "V2"=w481, "V3"=w480, "SlowTimer"=w485, "FastTimer"=w484, "listener ID"=refnum<k5> refnum, "TempPath"=w477, "LED vi reference"=w476, "Aquisition Timer"=w474, "APDSerialNum"=w473, "VideoConfig"=w472, "CaliPath"=w471) -> (w479:T20)  [unwired: 1 in]
        n219 = call <vilib>:"Add State(s) to Queue__JKI_lib_State_Machine.vi"("State(s) in (\"\")"=w507) -> ("States Out"=w506:string)  [unwired: 14 in]
      }
      frame "Data: LoadAPDData" {
        # "only load the last iRF for the moment"
        # "Load APD detector data\n(It is a separator no-op. You can make a copy of this frame to create a new Data frame)"
        n220 = Unbundle By Name(w538) -> ("APDSerialNum.Ch1APDSerial#"=w537:string, "APDSerialNum.Ch2APDSerial#"=w509:string, "APDSerialNum.Ch3APDSerial#"=w508:string)
        n221 = call "CreatFromSerialNumNoRaw.vi"("error in (no error)"=w536, "APD Serial #"=w537) -> ("error out"=w534:errorcluster, "APDClass out"=w535:refnum<class "APDClass.lvclass">)  [unwired: 8 in]
        n222 = call "CreatFromSerialNumNoRaw.vi"("error in (no error)"=w536, "APD Serial #"=w509) -> ("error out"=w523:errorcluster, "APDClass out"=w524:refnum<class "APDClass.lvclass">)  [unwired: 8 in]
        n223 = call "CreatFromSerialNumNoRaw.vi"("error in (no error)"=w536, "APD Serial #"=w508) -> ("error out"=w516:errorcluster, "APDClass out"=w517:refnum<class "APDClass.lvclass">)  [unwired: 8 in]
        n224 = call-dynamic "Read iRFData.vi"("error in (no error)"=w534, "APDClass in"=w535) -> ("iRFData"=w533:T29)  [unwired: 7 in, 2 out]
        n225 = call-dynamic "Read iRFData.vi"("error in (no error)"=w523, "APDClass in"=w524) -> ("iRFData"=w528:T29)  [unwired: 7 in, 2 out]
        n226 = call-dynamic "Read iRFData.vi"("error in (no error)"=w516, "APDClass in"=w517) -> ("iRFData"=w521:T29)  [unwired: 7 in, 2 out]
        n227 = Unbundle By Name(w533) -> ("iRFWFsAvg"=w532:dbl[][])
        n228 = Unbundle By Name(w528) -> ("iRFWFsAvg"=w527:dbl[][])
        n229 = Unbundle By Name(w521) -> ("iRFWFsAvg"=w520:dbl[][])
        n230 = Array Size(array=w532) -> (size(s)=w531:i32[])
        n231 = Array Size(array=w527) -> (size(s)=w522:i32[])
        n232 = Array Size(array=w520) -> (size(s)=w515:i32[])
        n233 = Index Array(array=w531, index=1) -> (element=w529:i32)
        n234 = Index Array(array=w522, index=1) -> (element=w525:i32)
        n235 = Index Array(array=w515, index=1) -> (element=w518:i32)
        n236 = Index Array(array=w532, index (row)=w529) -> (element=w514:dbl[])  [unwired: 1 in]
        n237 = Index Array(array=w527, index (row)=w525) -> (element=w513:dbl[])  [unwired: 1 in]
        n238 = Index Array(array=w520, index (row)=w518) -> (element=w512:dbl[])  [unwired: 1 in]
        n239 = Bundle("iRFWFsAvg"=w514, "iRFWFsAvg"=w513, "iRFWFsAvg"=w512) -> (w511:T30)  [unwired: 1 in]
        n240 = global write "GlobalVariables.vi" "LastUseiRF"(w511) -> ()
        n241 = call <vilib>:"Add State(s) to Queue__JKI_lib_State_Machine.vi"("State(s) in Front (\"\")"="UI: CaliAndiRFLoaded" ("State(s) in Front (\"\")"), "State(s) in (\"\")"=w541) -> ("States Out"=w540:string)  [unwired: 13 in]
      }
      frame "Data: parseRunData" {
        # "All APD bias"
        # "flash queue"
        # "Ch3&4"
        # "Ch1&2"
        # "Flash data from queue and save it in structure\n()"
        n242 = Flush Queue(queue=w569, error in (no error)=w562) -> (remaining elements=w567:cluster{"double data":dbl[][]}[], error out=w560:errorcluster)  [unwired: 1 out]
        n243 = Flush Queue(queue=w563, error in (no error)=w562) -> (remaining elements=w557:cluster{"V1":dbl, "V2":dbl, "V3":dbl}[], error out=w558:errorcluster)  [unwired: 1 out]
        n244 = Flush Queue(queue=w568, error in (no error)=w562) -> (remaining elements=w566:cluster{"double data":dbl[][]}[], error out=w559:errorcluster)  [unwired: 1 out]
        n245 = for {
          tunnel: w566 -> [w579] mode=indexing
          tunnel: [w578] -> w552 mode=concatenating
          n246 = Unbundle By Name(w579) -> ("double data"=w577:dbl[][])
          n247 = call "SeperateChanData.vi"("Input (Ch1&2)"=w577) -> ("Ch1"=w578:dbl[][])  [unwired: 1 out]
        }
        n248 = call "FLImDAQ_FGV.vi"() -> ("Read data"=w548:T5)  [unwired: 10 in, 1 out]
        n249 = Unbundle By Name(w548) -> ("Waveform to Avg"=w545:i16)
        n250 = for {
          tunnel: w557 -> [w576] mode=indexing
          tunnel: [w575] -> w549 mode=indexing
          tunnel: [w574] -> w547 mode=indexing
          tunnel: [w573] -> w546 mode=indexing
          n251 = Unbundle By Name(w576) -> ("V1"=w575:dbl, "V2"=w574:dbl, "V3"=w573:dbl)
        }
        n252 = for {
          tunnel: w567 -> [w583] mode=indexing
          tunnel: [w581] -> w551 mode=concatenating
          tunnel: [w580] -> w553 mode=concatenating
          n253 = Unbundle By Name(w583) -> ("double data"=w582:dbl[][])
          n254 = call "SeperateChanData.vi"("Input (Ch1&2)"=w582) -> ("Ch1"=w581:dbl[][], "Ch2"=w580:dbl[][])
        }
        n255 = call "DuplicateV(SubVI).vi"("Averaging"=w545, "V in"=w549) -> ("V out"=w544:dbl[])  [unwired: 9 in]
        n256 = call "DuplicateV(SubVI).vi"("Averaging"=w545, "V in"=w547) -> ("V out"=w543:dbl[])  [unwired: 9 in]
        n257 = call "DuplicateV(SubVI).vi"("Averaging"=w545, "V in"=w546) -> ("V out"=w542:dbl[])  [unwired: 9 in]
        n258 = Array Size(array=w544) -> (size(s)=→"V1 Size":i32)
        n259 = Array Size(array=w543) -> (size(s)=→"V2 Size":i32)
        n260 = Array Size(array=w542) -> (size(s)=→"V3 Size":i32)
        n261 = Bundle By Name(cluster=w564, "Ch1Data"=w551, "Ch2Data"=w553, "Ch3Data"=w552, "V1"=w544, "V2"=w543, "V3"=w542) -> (w565:T20)
        n262 = Array Size(array=w552) -> (size(s)=→"data Size":i32[])
        n263 = Merge Errors(w560, w559, w558) -> (w561:errorcluster)
        n264 = call <vilib>:"Add State(s) to Queue__JKI_lib_State_Machine.vi"("State(s) in (\"\")"=w572) -> ("States Out"=w571:string)  [unwired: 14 in]
      }
      frame "Data: loadLastUseiRF" {
        # "Load last use iRF.\n()"
        n265 = Unbundle By Name(w588) -> ("TempPath"=w587:path)
        n266 = Build Path(base path=w587, name or relative path="iRF.tdms") -> (appended path=w593:path)
        n267 = TDMS Open(11:w593) -> (0:w591:errorcluster, 3:w592:refnum<k34>)  [unwired: 6 in]
        n268 = TDMS Read(0:w592, 11:w591, 12:dbl[][] []) -> (4:w585:refnum<k34>, 10:w589:dbl[][], 15:w584:errorcluster)  [unwired: 5 in, 3 out]
        n269 = TDMS Close(8:w584, 11:w585) -> ()  [unwired: 2 out]
        n270 = case shown="No Error" w584 {
          tunnel: w589 -> [w603 _]
          tunnel: ["UI: CaliAndiRFLoaded" ("State(s) in Front (\"\")") "" ("Empty String Constant")] -> w586
          frame No Error {
            n271 = Index Array(array=w603, index (row)=0) -> (element=w600:dbl[])  [unwired: 1 in]
            n272 = Index Array(array=w603, index (row)=1) -> (element=w605:dbl[])  [unwired: 1 in]
            n273 = Index Array(array=w603, index (row)=2) -> (element=w604:dbl[])  [unwired: 1 in]
            n274 = Array Size(array=w600) -> (size(s)=→"iRF length":i32)
            n275 = Bundle(w600, w605, w604) -> (w602:cluster{dbl[], dbl[], dbl[]})  [unwired: 1 in]
            n276 = global write "GlobalVariables.vi" "LastUseiRF"(w602) -> ()
          }
          frame Error {
          }
        }
        n277 = call <vilib>:"Add State(s) to Queue__JKI_lib_State_Machine.vi"("State(s) in Front (\"\")"=w586, "State(s) in (\"\")"=w598) -> ("States Out"=w597:string)  [unwired: 13 in]
      }
      frame "Data: loadSystemCali" {
        # "Load last use calibration.\n()"
        n278 = Unbundle By Name(w618) -> ("CaliPath"=w617:path)
        n279 = Build Path(base path=w617, name or relative path="Calibration.tdms") -> (appended path=w616:path)
        n280 = call "ReadBGorCali (SubVI).vi"("DataType"=enum16{"BG", "Cali"}."Cali", "error in (no error)"=w615, "file path in"=w616) -> ("error out"=w613:errorcluster, "CtrlVCluster"=w611:T31, "AvgDataCluster"=w612:T32)  [unwired: 6 in]
        n281 = case shown="No Error" w613 {
          selector: w613 -> [w623 w637]
          tunnel: w612 -> [w634 _]
          tunnel: w611 -> [w630 _]
          tunnel: [w623 w637] -> w610
          frame No Error {
            n282 = Unbundle By Name(w630) -> ("V 1"=w629:dbl[], "V 2"=w627:dbl[], "V 3"=w626:dbl[])
            n283 = Unbundle By Name(w634) -> ("Channel 1"=w633:dbl[], "Channel 2"=w632:dbl[], "Channel 3"=w631:dbl[])
            n284 = Index Array(array=w629) -> (element=w628:dbl)  [unwired: 1 in]
            n285 = Index Array(array=w627) -> (element=w625:dbl)  [unwired: 1 in]
            n286 = Index Array(array=w626) -> (element=w624:dbl)  [unwired: 1 in]
            n287 = Bundle By Name(cluster=T12 {"Ch1 WF"=array[400 elements], "Ch2 WF"=array[400 elements], "Ch3 WF"=array[400 elements], "V1"=0.0, "V2"=0.0, "V3"=0.0} ("LastUseCaliData"), "Ch1 WF"=w633, "Ch2 WF"=w632, "Ch3 WF"=w631, "V1"=w628, "V2"=w625, "V3"=w624) -> (w635:T12)
            n288 = global write "GlobalVariables.vi" "SysCaliData"(w635) -> ()
          }
          frame Error {
          }
        }
        n289 = call <vilib>:"Add State(s) to Queue__JKI_lib_State_Machine.vi"("State(s) in (\"\")"=w622) -> ("States Out"=w621:string)  [unwired: 14 in]
      }
      frame "Data: loadLastUseBG" {
        w648 = enum16{"write", "read"}."write" ("action")
        # "check data size here. If not the same as current setting, return error."
        # "Load last use BG.\n()"
        n290 = Unbundle By Name(w658) -> ("TempPath"=w657:path)
        n291 = Build Path(base path=w657, name or relative path="Background.tdms") -> (appended path=w642:path)
        n292 = call "ReadBGorCali (SubVI).vi"("DataType"=enum16{"BG", "Cali"}."BG", "error in (no error)"=w641, "file path in"=w642) -> ("error out"=w640:errorcluster, "AvgDataCluster"=w653:T32)  [unwired: 6 in, 1 out]
        n293 = Unbundle By Name(w653) -> ("Channel 1"=w644:dbl[], "Channel 2"=w652:dbl[], "Channel 3"=w643:dbl[])
        n294 = call "FLImDAQ_FGV.vi"() -> ("Read data"=w656:T5)  [unwired: 10 in, 1 out]
        n295 = Unbundle By Name(w656) -> ("min record length"=w649:i32)
        n296 = Array Size(array=w643) -> (size(s)=w651:i32)
        "BG length" <- w651
        n297 = Equal?(x=w651, y=w649) -> (x = y?=w650:bool)
        n298 = Select(t="UI: BGLoaded" ("State(s) in Front (\"\")"), s=w650, f="UI: BGSizeError" ("State(s) in Front (\"\")")) -> (s? t:f=w639:string)
        n299 = case shown="True" w650 {
          tunnel: w644 -> [_ w668]
          tunnel: w652 -> [_ w667]
          tunnel: w643 -> [_ w666]
          tunnel: w649 -> [w664 _]
          tunnel: [w663 w668] -> w647
          tunnel: [w663 w667] -> w646
          tunnel: [w663 w666] -> w645
          frame False {
            # "If error set BG all 0, update UI"
            n300 = for {
              N: w664 -> [_]
              tunnel: [0.0] -> w663 mode=indexing
            }
          }
          frame True {
            # "If no error, check size match"
          }
        }
        n301 = call "BG3FGV.vi"("action"=w648, "BG3 in"=w645) -> ()  [unwired: 8 in, 2 out]
        n302 = call "BG1FGV.vi"("action"=w648, "BG1 in"=w647) -> ()  [unwired: 8 in, 2 out]
        n303 = call "BG2FGV.vi"("action"=w648, "BG2 in"=w646) -> ()  [unwired: 8 in, 2 out]
        n304 = call <vilib>:"Add State(s) to Queue__JKI_lib_State_Machine.vi"("State(s) in Front (\"\")"=w639, "State(s) in (\"\")"=w662) -> ("States Out"=w661:string)  [unwired: 13 in]
      }
      frame "Data: loadLastUseMacro" {
        # "Load last use BG and Cali and iRF.\n(It is a separator no-op. You can make a copy of this frame to create a new Data frame)"
        n305 = call <vilib>:"Add State(s) to Queue__JKI_lib_State_Machine.vi"("State(s) in Front (\"\")"="Data: loadLastUseBG\nData: loadSystemCali\nData: loadLastUseiRF\n/*Data: LoadAPDData" ("State(s) in Front (\"\")"), "State(s) in (\"\")"=w674) -> ("States Out"=w673:string)  [unwired: 13 in]
      }
      frame "Data: saveCalibration" {
        # "Average data and save calibration file. [Covers: REQ11]\n(It is a separator no-op. You can make a copy of this frame to create a new Data frame)"
        n306 = Unbundle By Name(w689) -> ("Ch1Data"=w688:dbl[][], "V1"=w687:dbl[], "Ch2Data"=w686:dbl[][], "V2"=w685:dbl[], "Ch3Data"=w684:dbl[][], "V3"=w683:dbl[], "Pathes.CaliPath"=w693:path, "IDs.Cali ID"=w692:i8)
        n307 = Increment(x=w692) -> (x+1=w690:i8)
        n308 = Bundle("Ch1Data"=w688, "V1"=w687) -> (w675:cluster{"Ch1Data":dbl[][], "V1":dbl[]})  [unwired: 1 in]
        n309 = Bundle("Ch2Data"=w686, "V2"=w685) -> (w678:cluster{"Ch2Data":dbl[][], "V2":dbl[]})  [unwired: 1 in]
        n310 = Bundle("Ch3Data"=w684, "V3"=w683) -> (w677:cluster{"Ch3Data":dbl[][], "V3":dbl[]})  [unwired: 1 in]
        n311 = Format Value(string ("")="Calibration" ("default name"), format string="%02d", value (0)=w690) -> (output string=w695:string)
        n312 = Build Path(base path=w693, name or relative path=w695) -> (appended path=w682:path)
        n313 = call "SaveBGorCali (SubVI).vi"("DataType"=enum16{"BG", "Cali"}."Cali", "SytemID"="UCDMC" ("System ID"), "BG path"=w682, "error in (no error)"=w680, "Channel 3"=w677, "Channel 2"=w678, "Channel1"=w675) -> ("error out"=w679:errorcluster)  [unwired: 4 in]
        n314 = call <vilib>:"Add State(s) to Queue__JKI_lib_State_Machine.vi"("State(s) in (\"\")"=w698) -> ("States Out"=w697:string)  [unwired: 14 in]
      }
      frame "Data: saveiRF" {
        w723 = enum16{"write", "read"}."read" ("action")
        # "Get iRF from decon stracture and save it on disk.\n(It is a separator no-op. You can make a copy of this frame to create a new Data frame)"
        n315 = Unbundle By Name(w716) -> ("TempPath"=w715:path)
        n316 = call "Ch1DeconEngineFGV.vi"("action(read)"=w723) -> ("Error Out"=w721:errorcluster, "Ch1DeconEngine out"=w722:refnum<class "LaguerreDeconEngineClass.lvclass">)  [unwired: 9 in]
        n317 = call "Ch2DeconEngineFGV.vi"("action(read)"=w723) -> ("Error Out"=w719:errorcluster, "Ch2DeconEngine out"=w720:refnum<class "LaguerreDeconEngineClass.lvclass">)  [unwired: 9 in]
        n318 = call "Ch3DeconEngineFGV.vi"("action(read)"=w723) -> ("Error Out"=w717:errorcluster, "Ch3DeconEngine out"=w718:refnum<class "LaguerreDeconEngineClass.lvclass">)  [unwired: 9 in]
        n319 = Build Path(base path=w715, name or relative path="iRF" ("default name")) -> (appended path=w713:path)
        n320 = call "getIRF.vi"("error in (no error)"=w721, "LaguerreDeconEngineClass in"=w722) -> ("iRF"=w702:dbl[])  [unwired: 7 in, 2 out]
        n321 = call "getIRF.vi"("error in (no error)"=w719, "LaguerreDeconEngineClass in"=w720) -> ("iRF"=w701:dbl[])  [unwired: 7 in, 2 out]
        n322 = call "getIRF.vi"("error in (no error)"=w717, "LaguerreDeconEngineClass in"=w718) -> ("iRF"=w700:dbl[])  [unwired: 7 in, 2 out]
        n323 = Build Array(w702, w701, w700) -> (w708:dbl[][])
        n324 = TDMS Open(8:w712, 10:T13."create or replace" ("operation (0:open)"), 11:w713) -> (0:w709:errorcluster, 3:w710:refnum<k34>)  [unwired: 4 in]
        n325 = Bundle("iRF"=w702, "iRF"=w701, "iRF"=w700) -> (w699:cluster{"iRF":dbl[], "iRF":dbl[], "iRF":dbl[]})  [unwired: 1 in]
        n326 = global write "GlobalVariables.vi" "LastUseiRF"(w699) -> ()
        n327 = TDMS Write(0:w710, 5:"iRF" ("group name in (Untitled)"), 7:string[] ["Ch1", "Ch2", "Ch3"] ("channel name(s) in (Untitled)"), 9:w708, 11:w709) -> (4:w705:refnum<k34>, 15:w704:errorcluster)  [unwired: 1 in, 2 out]
        n328 = TDMS Close(8:w704, 11:w705) -> (0:w703:errorcluster)  [unwired: 1 out]
        n329 = call <vilib>:"Add State(s) to Queue__JKI_lib_State_Machine.vi"("State(s) in (\"\")"=w726) -> ("States Out"=w725:string)  [unwired: 14 in]
      }
      frame "Data: saveBGtoFGV" {
        w732 = enum16{"write", "read"}."write" ("action")
        # "Save BG and pass it to FGV.\n(save BG to disk and set it to FGV)"
        n330 = Unbundle By Name(w735) -> ("Ch1Data"=w734:dbl[][], "Ch2Data"=w733:dbl[][], "Ch3Data"=w731:dbl[][])
        n331 = call "AvgArray.vi"("2D array in"=w734) -> ("1D Avg out"=w730:dbl[])  [unwired: 10 in]
        n332 = call "AvgArray.vi"("2D array in"=w733) -> ("1D Avg out"=w729:dbl[])  [unwired: 10 in]
        n333 = call "AvgArray.vi"("2D array in"=w731) -> ("1D Avg out"=w728:dbl[])  [unwired: 10 in]
        n334 = call "BG1FGV.vi"("action"=w732, "BG1 in"=w730) -> ()  [unwired: 8 in, 2 out]
        n335 = call "BG2FGV.vi"("action"=w732, "BG2 in"=w729) -> ()  [unwired: 8 in, 2 out]
        n336 = call "BG3FGV.vi"("action"=w732, "BG3 in"=w728) -> ()  [unwired: 8 in, 2 out]
        n337 = call <vilib>:"Add State(s) to Queue__JKI_lib_State_Machine.vi"("State(s) in (\"\")"=w738) -> ("States Out"=w737:string)  [unwired: 14 in]
      }
      frame "Data: saveBGtoFile" {
        w758 = "Background" ("name or relative path")
        # "Save BG and pass it to FGV.\n(save BG to disk and set it to FGV)"
        n338 = Unbundle By Name(w741) -> ("Pathes.BG Path"=w755:path, "IDs.BG ID"=w754:i8, "Ch1Data"=w753:dbl[][], "V1"=w752:dbl[], "Ch2Data"=w751:dbl[][], "V2"=w750:dbl[], "Ch3Data"=w749:dbl[][], "V3"=w748:dbl[], "TempPath"=w760:path)
        n339 = Increment(x=w754) -> (x+1=w759:i8)
        n340 = Format Value(string ("")=w758, format string="%02d", value (0)=w759) -> (output string=w757:string)
        n341 = Build Path(base path=w760, name or relative path=w758) -> (appended path=w743:path)
        n342 = call "File Dialog"("start path"=w755, "prompt"="Please select BG name, DO NOT CANCEL!", "default name"=w757) -> ("selected path"=w744:path)  [unwired: 9 in, 3 out]
        n343 = Bundle("Ch1Data"=w753, "V1"=w752) -> (w747:cluster{"Ch1Data":dbl[][], "V1":dbl[]})  [unwired: 1 in]
        n344 = Bundle("Ch2Data"=w751, "V2"=w750) -> (w746:cluster{"Ch2Data":dbl[][], "V2":dbl[]})  [unwired: 1 in]
        n345 = Bundle("Ch3Data"=w749, "V3"=w748) -> (w745:cluster{"Ch3Data":dbl[][], "V3":dbl[]})  [unwired: 1 in]
        n346 = Build Array(w744, w743) -> (w742:path[])
        n347 = for {
          tunnel: w747 -> [w771]
          tunnel: w746 -> [w770]
          tunnel: w745 -> [w769]
          shift-right: [w772] -> w739
          shift-left: w740 -> [w768]
          tunnel: w742 -> [w767] mode=indexing
          n348 = call "SaveBGorCali (SubVI).vi"("DataType"=enum16{"BG", "Cali"}."BG", "SytemID"="UCDMC", "BG path"=w767, "error in (no error)"=w768, "Channel 3"=w769, "Channel 2"=w770, "Channel1"=w771) -> ("error out"=w772:errorcluster)  [unwired: 4 in]
        }
        n349 = call <vilib>:"Add State(s) to Queue__JKI_lib_State_Machine.vi"("State(s) in (\"\")"=w764) -> ("States Out"=w763:string)  [unwired: 14 in]
      }
      frame "Data: showBG" {
        # "Show BG in seperate window.\n()"
        n350 = call "showBG.vi"() -> ()  [unwired: 12 in]
        n351 = call <vilib>:"Add State(s) to Queue__JKI_lib_State_Machine.vi"("State(s) in (\"\")"=w777) -> ("States Out"=w776:string)  [unwired: 14 in]
      }
      frame "Data: irfAlignment" {
        w825 = enum16{"write", "read"}."write" ("action")
        w778 = enum16{"write", "read"}."read" ("action")
        # "do iRF alignment in this state\n(It is a separator no-op. You can make a copy of this frame to create a new Data frame)"
        n352 = Unbundle By Name(w803) -> ("Ch1Data"=w841:dbl[][], "Ch2Data"=w840:dbl[][], "Ch3Data"=w839:dbl[][])
        n353 = call "AvgArray.vi"("2D array in"=w840) -> ("1D Avg out"=w780:dbl[])  [unwired: 10 in]
        n354 = call "AvgArray.vi"("2D array in"=w839) -> ("1D Avg out"=w779:dbl[])  [unwired: 10 in]
        n355 = call "AvgArray.vi"("2D array in"=w841) -> ("1D Avg out"=w781:dbl[])  [unwired: 10 in]
        n356 = call "Ch3DeconEngineFGV.vi"("Error In"=w838, "action(read)"=w778) -> ("Error Out"=w832:errorcluster, "Ch3DeconEngine out"=w833:refnum<class "LaguerreDeconEngineClass.lvclass">)  [unwired: 8 in]
        n357 = call "Ch1DeconEngineFGV.vi"("Error In"=w838, "action(read)"=w778) -> ("Error Out"=w836:errorcluster, "Ch1DeconEngine out"=w837:refnum<class "LaguerreDeconEngineClass.lvclass">)  [unwired: 8 in]
        n358 = call "Ch2DeconEngineFGV.vi"("Error In"=w838, "action(read)"=w778) -> ("Error Out"=w834:errorcluster, "Ch2DeconEngine out"=w835:refnum<class "LaguerreDeconEngineClass.lvclass">)  [unwired: 8 in]
        n359 = call "RemoveDCBG.vi"("WF in"=w779) -> ("DC"=w784:dbl, "WF out"=w791:dbl[])  [unwired: 8 in, 1 out]
        n360 = call "RemoveDCBG.vi"("WF in"=w780) -> ("DC"=w786:dbl, "WF out"=w792:dbl[])  [unwired: 8 in, 1 out]
        n361 = call "RemoveDCBG.vi"("WF in"=w781) -> ("DC"=w789:dbl, "WF out"=w793:dbl[])  [unwired: 8 in, 1 out]
        n362 = call "computeIRFAlignment.vi"("error in (no error)"=w832, "fIRF temp"=w791, "LaguerreDeconEngineClass in"=w833) -> ("error out"=w830:errorcluster, "LaguerreDeconEngineClass out"=w831:refnum<class "LaguerreDeconEngineClass.lvclass">)  [unwired: 6 in, 1 out]
        n363 = call "computeIRFAlignment.vi"("error in (no error)"=w834, "fIRF temp"=w792, "LaguerreDeconEngineClass in"=w835) -> ("error out"=w826:errorcluster, "LaguerreDeconEngineClass out"=w827:refnum<class "LaguerreDeconEngineClass.lvclass">)  [unwired: 6 in, 1 out]
        n364 = call "computeIRFAlignment.vi"("error in (no error)"=w836, "fIRF temp"=w793, "LaguerreDeconEngineClass in"=w837) -> ("error out"=w828:errorcluster, "LaguerreDeconEngineClass out"=w829:refnum<class "LaguerreDeconEngineClass.lvclass">)  [unwired: 6 in, 1 out]
        n365 = call "Ch1DeconEngineFGV.vi"("Error In"=w828, "action(read)"=w825, "Ch1DeconEngine in"=w829) -> ("Error Out"=w823:errorcluster, "Ch1DeconEngine out"=w824:refnum<class "LaguerreDeconEngineClass.lvclass">)  [unwired: 7 in]
        n366 = call "Ch2DeconEngineFGV.vi"("Error In"=w826, "action(read)"=w825, "Ch2DeconEngine in"=w827) -> ("Error Out"=w813:errorcluster, "Ch2DeconEngine out"=w814:refnum<class "LaguerreDeconEngineClass.lvclass">)  [unwired: 7 in]
        n367 = call "Ch3DeconEngineFGV.vi"("Error In"=w830, "action(read)"=w825, "Ch3DeconEngine in"=w831) -> ("Error Out"=w807:errorcluster, "Ch3DeconEngine out"=w808:refnum<class "LaguerreDeconEngineClass.lvclass">)  [unwired: 7 in]
        n368 = call "setfIRF.vi"("error in (no error)"=w807, "fIRF"=w791, "LaguerreDeconEngineClass in"=w808) -> ("error out"=w811:errorcluster, "LaguerreDeconEngineClass out"=w812:refnum<class "LaguerreDeconEngineClass.lvclass">)  [unwired: 7 in]
        n369 = call "setfIRF.vi"("error in (no error)"=w813, "fIRF"=w792, "LaguerreDeconEngineClass in"=w814) -> ("error out"=w817:errorcluster, "LaguerreDeconEngineClass out"=w818:refnum<class "LaguerreDeconEngineClass.lvclass">)  [unwired: 7 in]
        n370 = call "setfIRF.vi"("error in (no error)"=w823, "fIRF"=w793, "LaguerreDeconEngineClass in"=w824) -> ("error out"=w821:errorcluster, "LaguerreDeconEngineClass out"=w822:refnum<class "LaguerreDeconEngineClass.lvclass">)  [unwired: 7 in]
        n371 = call "computeLCs.vi"("error in (no error)"=w811, "LaguerreDeconClass in"=w812) -> ("error out"=w809:errorcluster, "LaguerreDeconClass out"=w810:refnum<class "LaguerreDeconEngineClass.lvclass">)  [unwired: 8 in]
        n372 = call "computeLCs.vi"("error in (no error)"=w817, "LaguerreDeconClass in"=w818) -> ("error out"=w815:errorcluster, "LaguerreDeconClass out"=w816:refnum<class "LaguerreDeconEngineClass.lvclass">)  [unwired: 8 in]
        n373 = call "computeLCs.vi"("error in (no error)"=w821, "LaguerreDeconClass in"=w822) -> ("error out"=w819:errorcluster, "LaguerreDeconClass out"=w820:refnum<class "LaguerreDeconEngineClass.lvclass">)  [unwired: 8 in]
        n374 = Unbundle By Name(w803) -> ("V1"=w802:dbl[], "V2"=w801:dbl[], "V3"=w800:dbl[])
        n375 = call-poly <vilib>:"Mean.vi"("X"=w802) -> ("mean"=w799:dbl)  [unwired: 1 out]
        n376 = call "getFitting.vi"("error in (no error)"=w809, "LaguerreDeconEngineClass in"=w810) -> ("Fitting"=w782:dbl[])  [unwired: 7 in, 2 out]
        n377 = call "getFitting.vi"("error in (no error)"=w815, "LaguerreDeconEngineClass in"=w816) -> ("Fitting"=w785:dbl[])  [unwired: 7 in, 2 out]
        n378 = Add(x=w786, y=w785) -> (x+y=w787:dbl[])
        n379 = call "getFitting.vi"("error in (no error)"=w819, "LaguerreDeconEngineClass in"=w820) -> ("Fitting"=w788:dbl[])  [unwired: 7 in, 2 out]
        n380 = Add(x=w789, y=w788) -> (x+y=w790:dbl[])
        n381 = call-poly <vilib>:"Mean.vi"("X"=w801) -> ("mean"=w798:dbl)  [unwired: 1 out]
        n382 = Add(x=w784, y=w782) -> (x+y=w783:dbl[])
        n383 = Build Array(w781, w790) -> (w806:dbl[][])
        n384 = Build Array(w780, w787) -> (w805:dbl[][])
        n385 = call-poly <vilib>:"Mean.vi"("X"=w800) -> ("mean"=w797:dbl)  [unwired: 1 out]
        n386 = Build Array(w779, w783) -> (w804:dbl[][])
        n387 = Bundle("mean"=w799, "mean"=w798, "mean"=w797) -> (w796:cluster{"mean":dbl, "mean":dbl, "mean":dbl})  [unwired: 1 in]
        n388 = call "Calib_and_iRFAlign_confirm.vi"("Ch4 Data"=w796, "Ch3 Data"=w804, "Ch2 Data"=w805, "Ch1 Data"=w806) -> ("Save?"=w795:bool)  [unwired: 7 in]
        n389 = case shown="True" w795 {
          tunnel: ["" ("Empty String Constant") "Data: saveCalibration\nData: saveiRF\nRun: CaliIncrement"] -> w794
          frame False {
          }
          frame True {
            # "[Covers: REQ2]"
          }
        }
        n390 = call <vilib>:"Add State(s) to Queue__JKI_lib_State_Machine.vi"("State(s) in Front (\"\")"=w794, "State(s) in (\"\")"=w844) -> ("States Out"=w843:string)  [unwired: 13 in]
      }
      frame "Data: saveRunData" {
        w852 = T33 {"DataPath"=path "", "CaseID"="", "RunID"=0, "Ch1Data"=[], "Ch2Data"=[], "Ch3Data"=[], "V1"=[], "V2"=[], "V3"=[], "LaserRepRate"=0, "WFAverage"=0}  # Data cluster
        # "Save FLIm data to disk.\n(Save to LV tdms file format)"
        n391 = Unbundle By Name(w856) -> ("Pathes.DataPath"=w866:path, "CaseID"=w865:string, "IDs.RunID"=w854:i8, "Ch1Data"=w864:dbl[][], "Ch2Data"=w863:dbl[][], "Ch3Data"=w862:dbl[][], "V1"=w861:dbl[], "V2"=w860:dbl[], "V3"=w859:dbl[])
        n392 = local read "Laser Rep Rate"() -> (w851:dbl)
        n393 = call "FLImDAQ_FGV.vi"("error in (no error)"=w848) -> ("error out"=w847:errorcluster, "Read data"=w850:T5)  [unwired: 9 in]
        n394 = Unbundle By Name(w850) -> ("Waveform to Avg"=w849:i16)
        n395 = Increment(x=w854) -> (x+1=w853:i8)
        n396 = Bundle By Name(cluster=w852, "DataPath"=w866, "CaseID"=w865, "RunID"=w853, "Ch1Data"=w864, "Ch2Data"=w863, "Ch3Data"=w862, "V1"=w861, "V2"=w860, "V3"=w859, "LaserRepRate"=w851, "WFAverage"=w849) -> (w858:T33)
        n397 = call "SaveRunData(SubVI).vi"("Data cluster"=w858, "error in (no error)"=w847) -> ("error out"=w855:errorcluster)  [unwired: 13 in]
        n398 = flat-sequence {
          tunnel: w856 -> [w874]
          tunnel: [w871] -> w857
          tunnel: w855 -> [_]
          frame #0 {
            w872 = dbl[][] [] ("Ch1Data")
            w873 = dbl[] [] ("V1")
            n399 = Bundle By Name(cluster=w874, "Ch1Data"=w872, "Ch2Data"=w872, "Ch3Data"=w872, "V1"=w873, "V2"=w873, "V3"=w873) -> (w871:T20)
          }
        }
        n400 = case shown="No Error" w855 {
          tunnel: ["Run: Increment" "" ("Empty String Constant")] -> w867
          frame No Error {
          }
          frame Error {
          }
        }
        n401 = call <vilib>:"Add State(s) to Queue__JKI_lib_State_Machine.vi"("State(s) in Front (\"\")"=w867, "State(s) in (\"\")"=w870) -> ("States Out"=w869:string)  [unwired: 13 in]
      }
      frame "Data: Cleanup" {
        # "Cleanup any data and references, here.\n(this is called automatically, by the Macro: Exit)"
        n402 = Unbundle By Name(w878) -> ("Core.Current VI Reference"=w881:refnum<vi>)
        n403 = Close Reference(reference=w881, error in (no error)=w880) -> (error out=w879:errorcluster)
        n404 = call <vilib>:"Add State(s) to Queue__JKI_lib_State_Machine.vi"("State(s) in (\"\")"=w883) -> ("States Out"=w882:string)  [unwired: 14 in]
      }
      frame "---------- Core ----------" {
        # "Do not put any code in this frame.\n(it is a separator no-op)"
        n405 = call <vilib>:"Add State(s) to Queue__JKI_lib_State_Machine.vi"("State(s) in (\"\")"=w888) -> ("States Out"=w887:string)  [unwired: 14 in]
      }
      frame Default {
        w899 = 42 items=["No error", "Argument error", "Memory is full", "Out of zone", "End of file", "File already open", "Generic file I/O error", "File not found", "File permission error", "Disk is full", "Duplicate path", "Too many files open", "System feature not enabled", "Resource file not found", "Cannot add resource", "Resource not found", "Image not found", "Image memory error", "Pen does not exist", "Config type invalid", "Config token not found", "Config parse error", "Config memory error", "Bad external code format", "Bad external code offset", "External code not present", "Null window", "Destroy window error", "Null menu", "Print aborted", "Bad print record", "Print driver error", "Windows error during printing", "Memory error during printing", "Print dialog error", "Generic print error", "Invalid device refnum", "Device not found", "Device parameter error", "Device unit error", "Cannot open device", "Device call aborted", "Generic error", "Cancelled by user", "Object ID too low", "Object ID too high", "Object not in heap", "Unknown heap", "Unknown object (invalid DefProc)", "Unknown object (DefProc not in table)", "Message out of range", "Invalid (null) method", "Unknown message", "Manager call not supported", "Bad address", "Network operation in progress", "Network operation timed out", "Connection is busy", "Network attribute not supported", "Network error", "Address in use", "System out of memory", "Connection aborted", "Connection refused", "Not connected", "Already connected", "Connection closed", "Initialization error (interapplication manager)", "Bad occurrence", "Wait on unbound occurrence handler", "Occurrence queue overflow", "Datalog type conflict", "Unused", "Unrecognized type (interapplication manager)", "Memory corrupt", "Failed to make temporary DLL", "Old CIN version", "Drag socket not found", "Failed to load drop-object", "Failed to register OLE object", "Failed to release OLE object", "Format specifier type mismatch", "Unknown format specifier", "Too few format specifiers", "Too many format specifiers", "Scan failed", "Newer CIN version", "Error converting to variant", "Runtime menu error", "Password tampered", "Variant attribute not found", "Incompatible variant data type", "Event data is not available", "Event Store is not present", "Occurrence is not found", "Event Queue is not created", "Event info is not available", "Refnum passed is NULL", "Error retrieving Class GUID", "Error retrieving CoClass GUID", "Error retrieving TypeLib GUID.", "Bad built application magic bytes.", "Specific driver is different from the specific driver associated with the Logical Name.", "There is no session opened to the class driver.", "Max Error", "MAX - Error with config objects", "MAX - Error loading configuration", "MAX - Group not supported"]
        # "Current State"
        # "Do not delete, rename, or modify this frame.\n(this is used to capture unhandled states and typos)"
        # "Handle mistyped state name (developer tool)"
        n406 = Format Into String(format string="Software Exception: Unhandled State \"%s\"." ("message"), error in=w895, w890) -> (resulting string=w898:string, error out=w897:errorcluster)  [unwired: 1 in]
        n407 = call <vilib>:"Error Cluster From Error Code.vi"("show call chain? (False)"=TRUE, "error in (no error)"=w897, "error message (\"\")"=w898, "error code (0)"=w899) -> ("error out"=w896:errorcluster)  [unwired: 5 in]
        n408 = call <vilib>:"Add State(s) to Queue__JKI_lib_State_Machine.vi"("State(s) in (\"\")"=w894) -> ("States Out"=w893:string)  [unwired: 14 in]
      }
      frame "Initialize Core Data" {
        # "Build default path based on the location of project"
        # "Do not delete, rename, or modify this frame.\n(this is used to determine panel behavior on exit)"
        # "originally closed?"
        # "exe?"
        # "If panel starts closed or is an EXE, then close it when we exit"
        n409 = call <vilib>:"Application Directory.vi"() -> ("Application Directory"=w903:path)
        n410 = property on="Property Node" class="App"() -> ("App.Kind"=w917:T15)  [unwired: 2 in, 2 out]
        n411 = property on="Property Node" class="VI"() -> ("FP.State"=w911:T14)  [unwired: 2 in, 2 out]
        n412 = control-ref of="Current VI Reference"() -> (w912:refnum<vi>)
        n413 = Equal?(x=w911, y=T14."Closed" ("Front Panel Window:State")) -> (x = y?=w909:bool)
        n414 = Equal?(x=w917, y=T15."Run Time System" ("Application:Kind")) -> (x = y?=w915:bool)
        n415 = Build Path(base path=w903, name or relative path="Data") -> (appended path=w907:path)
        n416 = Build Path(base path=w903, name or relative path="SystemTemp") -> (appended path=w904:path)
        n417 = Build Path(base path=w903, name or relative path="SystemCalibrationFile") -> (appended path=w901:path)
        n418 = Or(x=w909, y=w915) -> (x .or. y?=w913:bool)
        n419 = Bundle By Name(cluster=w914, "Core.Current VI Reference"=w912, "Core.Close Panel on Exit?"=w913, "DefaultPath"=w907, "TempPath"=w904, "CaliPath"=w901) -> (w919:T20)
        n420 = call <vilib>:"Add State(s) to Queue__JKI_lib_State_Machine.vi"("State(s) in (\"\")"=w921) -> ("States Out"=w920:string)  [unwired: 14 in]
      }
      frame "Error Handler" {
        # "Unhandled Error -- Display it"
        # "Handle any errors here.\nYou can also output any states to clean-up after errors occur"
        # "Clear error"
        n421 = Unbundle By Name(w922) -> ("code"=w924:i32)
        n422 = case shown="5002" w924 {
          tunnel: ["Macro: Exit" w934 w940] -> w923
          tunnel: w922 -> [w930 _ _]
          frame Default {
            w932 = T34 1 items=["no dialog", "OK message", "continue or stop message", "OK message + warnings", "continue/stop + warnings"] ("type of dialog (OK msg:1)")
            n423 = call <vilib>:"General Error Handler.vi"("type of dialog (OK msg:1)"=w932, "error in (no error)"=w930) -> ()  [unwired: 9 in, 5 out]
          }
          frame 5002 {
            n424 = Two Button Dialog(message="Laser interlock open! Please close interlock and try again! ", 1:"Safely Shutdown" ("F button name (\"Cancel\")"), 2:"OK" ("T button name (\"OK\")")) -> (T button?=w935:bool)
            n425 = case shown="True" w935 {
              tunnel: ["Macro: Exit" "355 Laser: CheckControllerStatus"] -> w934
              frame False {
              }
              frame True {
              }
            }
          }
          frame 5001 {
            n426 = Two Button Dialog(message="Unable to connect to imaging computer, do you want to run data aquisiton alone? ", 1:"No" ("F button name (\"Cancel\")"), 2:"Yes" ("T button name (\"OK\")")) -> (T button?=w941:bool)
            n427 = case shown="False" w941 {
              tunnel: ["Macro: Exit" "" ("Empty String Constant")] -> w940
              frame False {
              }
              frame True {
              }
            }
          }
        }
        n428 = call <vilib>:"Add State(s) to Queue__JKI_lib_State_Machine.vi"("State(s) in Front (\"\")"=w923, "State(s) in (\"\")"=w929) -> ("States Out"=w928:string)  [unwired: 13 in]
      }
      frame "Exit" {
        # "Do not put any code in this frame.\n(No errors that occur here will be handled.)"
        n429 = call <vilib>:"Add State(s) to Queue__JKI_lib_State_Machine.vi"("State(s) in (\"\")"=w952) -> ("States Out"=w951:string)  [unwired: 14 in]
      }
      frame "---------- AimingBeam ----------" {
        # "Template Separator\n(You can make a copy of, or modify, this frame)"
        n430 = call <vilib>:"Add State(s) to Queue__JKI_lib_State_Machine.vi"("State(s) in (\"\")"=w957) -> ("States Out"=w956:string)  [unwired: 14 in]
      }
      frame "AimingBeam: Initialize" {
        # "set aiming beam button color"
        # "Open COM port for Aiming Beam\n(Require USB connection)"
        n431 = Unbundle By Name(w959) -> ("AB Cluster.Aiming Beam COM Port"=w967:refnum<visa-resource-name>)
        n432 = call-poly "VISA Configure Serial Port"("VISA resource name"=w967, "Enable Termination\nChar (T)"=TRUE ("Enable Termination\nChar (T)"), "baud rate (9600)"=u32 9600, "error in (no error)"=w964) -> ("error out"=w963:errorcluster)  [unwired: 10 in, 1 out]
        n433 = Unbundle By Name(w963) -> ("status"=w962:bool)
        n434 = Not(x=w962) -> (.not. x?=w961:bool)
        n435 = Bundle By Name(cluster=w959, "System Status.Aiming Beam"=w961) -> (w960:T20)
        n436 = call <vilib>:"Add State(s) to Queue__JKI_lib_State_Machine.vi"("State(s) in (\"\")"=w969) -> ("States Out"=w968:string)  [unwired: 14 in]
      }
      frame "AimingBeam: Close" {
        # "Close Aiming Beam COM port\n(Require USB connection to Aiming Beam Laser)"
        n437 = Unbundle By Name(w972) -> ("AB Cluster.Aiming Beam COM Port"=w976:refnum<visa-resource-name>)
        n438 = VISA Close(VISA resource name=w976, error in (no error)=w974) -> (error out=w975:errorcluster)
        n439 = Bundle By Name(cluster=w972, "System Status.Aiming Beam"=FALSE) -> (w973:T20)
        n440 = call <vilib>:"Add State(s) to Queue__JKI_lib_State_Machine.vi"("State(s) in (\"\")"=w978) -> ("States Out"=w977:string)  [unwired: 14 in]
      }
      frame "AimingBeam: Set Current" {
        # "Set Aiming Beam Current\n(You can make a copy of, or modify, this frame)"
        n441 = Unbundle By Name(w993) -> ("AB Cluster.Aiming Beam COM Port"=w986:refnum<visa-resource-name>, "AB Cluster.Max Current"=w982:dbl, "AB Cluster.Default Current"=w984:dbl, "AB Cluster.Min Current"=w983:dbl)
        n442 = In Range and Coerce(upper limit=w982, x=w984, lower limit=w983) -> (coerced(x)=w979:dbl)  [unwired: 1 out]
        n443 = Number To Fractional String(number=w979, precision (6)=i16 2) -> (F-format string=w987:string)  [unwired: 2 in]
        n444 = Concatenate Strings("slc:", w987, "\r" ("Carriage Return Constant"), "\n" ("Line Feed Constant")) -> (w990:string)
        n445 = VISA Write(VISA resource name=w986, write buffer=w990, error in (no error)=w981) -> (error out=w985:errorcluster)  [unwired: 2 out]
        n446 = call <vilib>:"Add State(s) to Queue__JKI_lib_State_Machine.vi"("State(s) in (\"\")"=w995) -> ("States Out"=w994:string)  [unwired: 14 in]
      }
      frame "AimingBeam: Set Status" {
        # "Enable Aiming Beam\n(Usage: \"AimingBeam: Set >> Enable|Disable\")"
        n447 = Unbundle By Name(w1002) -> ("AB Cluster.Aiming Beam COM Port"=w999:refnum<visa-resource-name>)
        n448 = case shown="\"Enable\"" w1001 {
          tunnel: [w1005 w1009] -> w1000
          frame "Disable", Default {
            n449 = Concatenate Strings("cof", "\r" ("Carriage Return Constant"), "\n" ("Line Feed Constant")) -> (w1005:string)
          }
          frame "Enable" {
            n450 = Concatenate Strings("con", "\r" ("Carriage Return Constant"), "\n" ("Line Feed Constant")) -> (w1009:string)
          }
        }
        n451 = VISA Write(VISA resource name=w999, write buffer=w1000, error in (no error)=w997) -> (error out=w998:errorcluster)  [unwired: 2 out]
        n452 = call <vilib>:"Add State(s) to Queue__JKI_lib_State_Machine.vi"("State(s) in (\"\")"=w1004) -> ("States Out"=w1003:string)  [unwired: 14 in]
      }
      frame "AimingBeam: GetPWMStatus" {
        # "Get aiming beam PWM status\n()"
        n453 = Unbundle By Name(w1017) -> ("AB Cluster.Freq"=w1016:i32, "LJ Pinout.AimingBeam PWM"=w1023:string)
        n454 = Equal To 0?(x=w1016) -> (x = 0?=w1015:bool)
        n455 = call "LabJack_FGV.vi"("Operation(Read)"=enum16{"Write", "Read"}."Read" ("Operation"), "error in (no error)"=w1019) -> ("error out"=w1021:errorcluster, "Read data"=w1022:i32)  [unwired: 8 in]
        n456 = case shown="True" w1015 {
          tunnel: w1023 -> [w1036 _]
          tunnel: [w1034 "DIO_STATE"] -> w1020
          frame False {
            n457 = Concatenate Strings(w1036, "_EF_ENABLE" ("string")) -> (w1034:string)
          }
          frame True {
          }
        }
        n458 = call "LJM_eReadName.vi"("Handle In"=w1022, "Name"=w1020, "error in"=w1021) -> ("Value"=w1014:dbl, "error out"=w1018:errorcluster)  [unwired: 10 in, 1 out]
        n459 = case shown="True" w1015 {
          tunnel: w1014 -> [w1029 w1033]
          tunnel: [w1028 w1030] -> w1013
          frame False {
            n460 = Greater Than 0?(x=w1029) -> (x > 0?=w1028:bool)
          }
          frame True {
            n461 = Number To Boolean Array(number=w1033) -> (Boolean array=w1032:bool[])
            n462 = Index Array(array=w1032, index=3) -> (element=w1030:bool)
          }
        }
        n463 = case shown="True" w1013 {
          frame False {
            # "PWM is off\nset color to dark green"
            n464 = local write "Aiming beam toggle"(FALSE ("Aimging beam")) -> ()
          }
          frame True {
            # "PWM is on\nset color to light green"
            n465 = local write "Aiming beam toggle"(TRUE ("Aimging beam")) -> ()
          }
        }
        n466 = call <vilib>:"Add State(s) to Queue__JKI_lib_State_Machine.vi"("State(s) in (\"\")"=w1027) -> ("States Out"=w1026:string)  [unwired: 14 in]
      }
      frame "---------- Case ----------" {
        # "Template Separator\n(You can make a copy of, or modify, this frame)"
        n467 = call <vilib>:"Add State(s) to Queue__JKI_lib_State_Machine.vi"("State(s) in (\"\")"=w1044) -> ("States Out"=w1043:string)  [unwired: 14 in]
      }
      frame "Case: getCaliID" {
        # "Get Calibration file #\n(You can make a copy of, or modify, this frame)"
        n468 = Unbundle By Name(w1045) -> ("Pathes.CaliPath"=w1048:path)
        n469 = call <vilib>:"Recursive File List.vi"("pattern"="*.tdms", "Treat LLBs as Folders?"=FALSE, "Folder Path"=w1048) -> ("All Files in Dir"=w1053:path[])  [unwired: 4 in, 4 out]
        n470 = for {
          tunnel: w1053 -> [w1063] mode=indexing
          tunnel: [w1062] -> w1052 mode=indexing
          tunnel: "Calibration" -> [w1059]
          n471 = Strip Path(path=w1063) -> (name=w1060:string)  [unwired: 1 out]
          n472 = Search and Replace String(input string=w1060, search string=w1059) -> (result string=w1058:string)  [unwired: 6 in, 3 out]
          n473 = Scan From String(format string="%d" ("string"), input string=w1058) -> (output 1=w1062:i32)  [unwired: 3 in, 3 out]
        }
        n474 = Array Max & Min(array=w1052) -> (max value=w1051:i32)  [unwired: 3 out]
        n475 = Bundle By Name(cluster=w1045, "IDs.Cali ID"=w1051) -> (w1046:T20)
        n476 = call <vilib>:"Add State(s) to Queue__JKI_lib_State_Machine.vi"("State(s) in (\"\")"=w1057) -> ("States Out"=w1056:string)  [unwired: 14 in]
      }
      frame "Case: getBGID" {
        # "Get background #\n(You can make a copy of, or modify, this frame)"
        n477 = Unbundle By Name(w1066) -> ("Pathes.BG Path"=w1071:path)
        n478 = call <vilib>:"Recursive File List.vi"("pattern"="*.tdms", "Treat LLBs as Folders?"=FALSE, "Folder Path"=w1071) -> ("All Files in Dir"=w1069:path[])  [unwired: 4 in, 4 out]
        n479 = for {
          tunnel: w1069 -> [w1086] mode=indexing
          tunnel: "Background" ("name or relative path") -> [w1084]
          shift-right: [w1077] -> w1064
          shift-left: 0 -> [w1081]
          n480 = Strip Path(path=w1086) -> (name=w1085:string)  [unwired: 1 out]
          n481 = Search and Replace String(input string=w1085, search string=w1084) -> (number of replacements=w1083:i32)  [unwired: 6 in, 3 out]
          n482 = Greater Than 0?(x=w1083) -> (x > 0?=w1082:bool)
          n483 = Select(t=1, s=w1082, f=0) -> (s? t:f=w1080:i32)
          n484 = Add(x=w1080, y=w1081) -> (x+y=w1077:i32)
        }
        n485 = Bundle By Name(cluster=w1066, "IDs.BG ID"=w1064) -> (w1067:T20)
        n486 = call <vilib>:"Add State(s) to Queue__JKI_lib_State_Machine.vi"("State(s) in (\"\")"=w1076) -> ("States Out"=w1075:string)  [unwired: 14 in]
      }
      frame "Case: getRunID" {
        # "Check folder for run ID\n(You can make a copy of, or modify, this frame)"
        n487 = Unbundle By Name(w1092) -> ("Pathes.DataPath"=w1091:path, "CaseID"=w1087:string)
        n488 = Build Array("Background" ("name or relative path"), "Calibration") -> (w1098:string[])
        n489 = call <vilib>:"Recursive File List.vi"("Folders to Exclude"=w1098, "pattern"="*.tdms", "Treat LLBs as Folders?"=FALSE, "Folder Path"=w1091) -> ("All Files in Dir"=w1088:path[])  [unwired: 3 in, 4 out]
        n490 = for {
          tunnel: w1088 -> [w1108] mode=indexing
          tunnel: [w1107] -> w1094 mode=indexing
          tunnel: w1087 -> [w1104]
          n491 = Strip Path(path=w1108) -> (name=w1105:string)  [unwired: 1 out]
          n492 = Search and Replace String(input string=w1105, search string=w1104) -> (result string=w1103:string)  [unwired: 6 in, 3 out]
          n493 = Scan From String(format string="_%d" ("string"), input string=w1103) -> (output 1=w1107:i32)  [unwired: 3 in, 3 out]
        }
        n494 = Array Max & Min(array=w1094) -> (max value=w1095:i32)  [unwired: 3 out]
        n495 = Bundle By Name(cluster=w1092, "IDs.RunID"=w1095) -> (w1093:T20)
        n496 = call <vilib>:"Add State(s) to Queue__JKI_lib_State_Machine.vi"("State(s) in (\"\")"=w1102) -> ("States Out"=w1101:string)  [unwired: 14 in]
      }
      frame "Case: CreatFileStruct" {
        # "Creat case file structure"
        n497 = Unbundle By Name(w1120) -> ("DefaultPath"=w1126:path, "CaseID"=w1111:string)
        n498 = Build Path(base path=w1126, name or relative path=w1111) -> (appended path=w1125:path)
        n499 = call <vilib>:"Check if File or Folder Exists.vi"("error in (no error)"=w1118, "path"=w1125) -> ("error out"=w1122:errorcluster, "file or folder exists?"=w1124:bool, "dup path"=w1123:path)  [unwired: 7 in]
        n500 = case shown="True" w1124 {
          tunnel: w1123 -> [w1143 w1151]
          tunnel: w1122 -> [w1141 w1146]
          tunnel: [w1135 w1151] -> w1116
          tunnel: [w1139 w1153] -> w1119
          tunnel: [u32 0 u32 0] -> w1110
          tunnel: [w1137 w1156] -> w1115
          tunnel: "Background" ("name or relative path") -> [w1136 w1148]
          tunnel: "Calibration" -> [w1134 w1147]
          tunnel: [w1130 w1149] -> w1112
          tunnel: w1111 -> [_ _]
          tunnel: ["" ("Empty String Constant") "Case: getRunID\nCase: getBGID\nCase: getCaliID\nUI: Update"] -> w1109
          frame False {
            # "Folder not exist. Creat folders."
            n501 = Create Folder(path (use dialog)=w1143, error in=w1141) -> (created path=w1135:path, error out=w1132:errorcluster)  [unwired: 1 in, 1 out]
            n502 = Build Path(base path=w1135, name or relative path=w1134) -> (appended path=w1133:path)
            n503 = Build Path(base path=w1135, name or relative path=w1136) -> (appended path=w1142:path)
            n504 = Create Folder(path (use dialog)=w1142, error in=w1132) -> (created path=w1137:path, error out=w1138:errorcluster)  [unwired: 1 in, 1 out]
            n505 = Create Folder(path (use dialog)=w1133, error in=w1132) -> (created path=w1130:path, error out=w1131:errorcluster)  [unwired: 1 in, 1 out]
            n506 = Merge Errors(w1138, w1131) -> (w1139:errorcluster)
          }
          frame True {
            # "Folder exsit, check file #"
            n507 = Build Path(base path=w1151, name or relative path=w1147) -> (appended path=w1152:path)
            n508 = Build Path(base path=w1151, name or relative path=w1148) -> (appended path=w1157:path)
            n509 = call <vilib>:"Check if File or Folder Exists.vi"("path"=w1152) -> ("file or folder exists?"=w1150:bool, "dup path"=w1149:path)  [unwired: 8 in, 1 out]
            n510 = call <vilib>:"Check if File or Folder Exists.vi"("path"=w1157) -> ("file or folder exists?"=w1155:bool, "dup path"=w1156:path)  [unwired: 8 in, 1 out]
            n511 = And(x=w1155, y=w1150) -> (x .and. y?=w1154:bool)
            n512 = case shown="False" w1154 {
              tunnel: w1146 -> [_ w1159]
              tunnel: [errorcluster {"status"=TRUE, "code"=5003, "source"="File structure error."} ("error out") w1159] -> w1153
              frame False {
              }
              frame True {
              }
            }
          }
        }
        n513 = Bundle By Name(cluster=w1120, "Pathes.DataPath"=w1116, "Pathes.BG Path"=w1115, "Pathes.CaliPath"=w1112, "IDs.RunID"=w1110, "IDs.BG ID"=w1110, "IDs.Cali ID"=w1110) -> (w1121:T20)
        n514 = call <vilib>:"Add State(s) to Queue__JKI_lib_State_Machine.vi"("State(s) in Front (\"\")"=w1109, "State(s) in (\"\")"=w1128) -> ("States Out"=w1127:string)  [unwired: 13 in]
      }
      frame "Case: GetID" {
        # "Template Separator\n(You can make a copy of, or modify, this frame)"
        n515 = call "set_subjectID.vi"() -> ("subject_id"=w1160:string)  [unwired: 10 in]
        n516 = Bundle By Name(cluster=w1162, "CaseID"=w1160) -> (w1163:T20)
        n517 = call <vilib>:"Add State(s) to Queue__JKI_lib_State_Machine.vi"("State(s) in (\"\")"=w1166) -> ("States Out"=w1165:string)  [unwired: 14 in]
      }
      frame "---------- DeconEngine ----------" {
        # "start data aquisition and then set irfAligh to ture and decon channel to 1,2 and 3."
        # "Template Separator\n(You can make a copy of, or modify, this frame)"
        n518 = call <vilib>:"Add State(s) to Queue__JKI_lib_State_Machine.vi"("State(s) in (\"\")"=w1171) -> ("States Out"=w1170:string)  [unwired: 14 in]
      }
      frame "DeconEngine: InitilizeMacro" {
        # "start data aquisition and then set irfAligh to ture and decon channel to 1,2 and 3."
        # "Initilize Decon Engine for all channel\n(You can make a copy of, or modify, this frame)"
        n519 = call <vilib>:"Add State(s) to Queue__JKI_lib_State_Machine.vi"("State(s) in Front (\"\")"="DeconEngine: InitializeCh1\nDeconEngine: InitializeCh2\nDeconEngine: InitializeCh3" ("State(s) in Front (\"\")"), "State(s) in (\"\")"=w1177) -> ("States Out"=w1176:string)  [unwired: 13 in]
      }
      frame "DeconEngine: InitializeCh1" {
        w1201 = refnum<class "LaguerreDeconEngineClass.lvclass"> refnum  # Ch1DeconObj
        # "Initilize Laguerre Deconvolution engine Object\n(You can make a copy of, or modify, this frame)"
        n520 = call "FLImDAQ_FGV.vi"("error in (no error)"=w1186) -> ("error out"=w1197:errorcluster, "Read data"=w1196:T5)  [unwired: 9 in]
        n521 = global read "GlobalVariables.vi" "LastUseiRF"() -> (w1179:T35)
        n522 = Unbundle By Name(w1196) -> ("min record length"=w1195:i32)
        n523 = call "setLaguerreOrder.vi"("error in (no error)"=w1197, "LaguerreOrder"=u32 12, "LaguerreDeconClass in"=w1201) -> ("error out"=w1198:errorcluster, "LaguerreDeconClass out"=w1199:refnum<class "LaguerreDeconEngineClass.lvclass">)  [unwired: 7 in]
        n524 = Unbundle By Name(w1179) -> ("Ch1 iRF"=w1178:dbl[])
        n525 = call "setDataLength.vi"("error in (no error)"=w1198, "dataLength"=w1195, "LaguerreDeconClass in"=w1199) -> ("error out"=w1194:errorcluster, "LaguerreDeconClass out"=w1193:refnum<class "LaguerreDeconEngineClass.lvclass">)  [unwired: 7 in]
        n526 = call "setIRF.vi"("error in (no error)"=w1194, "iRF"=w1178, "LaguerreDeconClass in"=w1193) -> ("error out"=w1191:errorcluster, "LaguerreDeconClass out"=w1192:refnum<class "LaguerreDeconEngineClass.lvclass">)  [unwired: 7 in]
        n527 = call "computeAlpha.vi"("error in (no error)"=w1191, "LaguerreDeconClass in"=w1192) -> ("error out"=w1189:errorcluster, "LaguerreDeconClass out"=w1190:refnum<class "LaguerreDeconEngineClass.lvclass">)  [unwired: 8 in]
        n528 = call "dataInitilize.vi"("error in (no error)"=w1189, "LaguerreDeconClass in"=w1190) -> ("error out"=w1187:errorcluster, "LaguerreDeconClass out"=w1188:refnum<class "LaguerreDeconEngineClass.lvclass">)  [unwired: 8 in]
        n529 = call "computeDeconMatrix.vi"("error in (no error)"=w1187, "LaguerreDeconClass in"=w1188) -> ("error out"=w1183:errorcluster, "LaguerreDeconClass out"=w1185:refnum<class "LaguerreDeconEngineClass.lvclass">)  [unwired: 8 in]
        n530 = call "Ch1DeconEngineFGV.vi"("Error In"=w1183, "action(read)"=enum16{"write", "read"}."write" ("action"), "Ch1DeconEngine in"=w1185) -> ("Error Out"=w1182:errorcluster)  [unwired: 7 in, 1 out]
        n531 = call <vilib>:"Add State(s) to Queue__JKI_lib_State_Machine.vi"("State(s) in (\"\")"=w1203) -> ("States Out"=w1202:string)  [unwired: 14 in]
      }
      frame "DeconEngine: InitializeCh2" {
        w1227 = refnum<class "LaguerreDeconEngineClass.lvclass"> refnum  # Ch2DeconObj
        # "Initilize Laguerre Deconvolution engine Object\n(You can make a copy of, or modify, this frame)"
        n532 = global read "GlobalVariables.vi" "LastUseiRF"() -> (w1205:T35)
        n533 = call "FLImDAQ_FGV.vi"("error in (no error)"=w1213) -> ("error out"=w1206:errorcluster, "Read data"=w1223:T5)  [unwired: 9 in]
        n534 = call "setLaguerreOrder.vi"("error in (no error)"=w1206, "LaguerreOrder"=u32 12, "LaguerreDeconClass in"=w1227) -> ("error out"=w1224:errorcluster, "LaguerreDeconClass out"=w1225:refnum<class "LaguerreDeconEngineClass.lvclass">)  [unwired: 7 in]
        n535 = Unbundle By Name(w1223) -> ("min record length"=w1222:i32)
        n536 = Unbundle By Name(w1205) -> ("Ch2 iRF"=w1204:dbl[])
        n537 = call "setDataLength.vi"("error in (no error)"=w1224, "dataLength"=w1222, "LaguerreDeconClass in"=w1225) -> ("error out"=w1221:errorcluster, "LaguerreDeconClass out"=w1220:refnum<class "LaguerreDeconEngineClass.lvclass">)  [unwired: 7 in]
        n538 = call "setIRF.vi"("error in (no error)"=w1221, "iRF"=w1204, "LaguerreDeconClass in"=w1220) -> ("error out"=w1218:errorcluster, "LaguerreDeconClass out"=w1219:refnum<class "LaguerreDeconEngineClass.lvclass">)  [unwired: 7 in]
        n539 = call "computeAlpha.vi"("error in (no error)"=w1218, "LaguerreDeconClass in"=w1219) -> ("error out"=w1216:errorcluster, "LaguerreDeconClass out"=w1217:refnum<class "LaguerreDeconEngineClass.lvclass">)  [unwired: 8 in]
        n540 = call "dataInitilize.vi"("error in (no error)"=w1216, "LaguerreDeconClass in"=w1217) -> ("error out"=w1214:errorcluster, "LaguerreDeconClass out"=w1215:refnum<class "LaguerreDeconEngineClass.lvclass">)  [unwired: 8 in]
        n541 = call "computeDeconMatrix.vi"("error in (no error)"=w1214, "LaguerreDeconClass in"=w1215) -> ("error out"=w1210:errorcluster, "LaguerreDeconClass out"=w1212:refnum<class "LaguerreDeconEngineClass.lvclass">)  [unwired: 8 in]
        n542 = call "Ch2DeconEngineFGV.vi"("Error In"=w1210, "action(read)"=enum16{"write", "read"}."write" ("action"), "Ch2DeconEngine in"=w1212) -> ("Error Out"=w1209:errorcluster)  [unwired: 7 in, 1 out]
        n543 = call <vilib>:"Add State(s) to Queue__JKI_lib_State_Machine.vi"("State(s) in (\"\")"=w1229) -> ("States Out"=w1228:string)  [unwired: 14 in]
      }
      frame "DeconEngine: InitializeCh3" {
        w1230 = refnum<class "LaguerreDeconEngineClass.lvclass"> refnum  # Ch3DeconObj
        # "Initilize Laguerre Deconvolution engine Object\n(You can make a copy of, or modify, this frame)"
        n544 = call "FLImDAQ_FGV.vi"("error in (no error)"=w1239) -> ("error out"=w1250:errorcluster, "Read data"=w1249:T5)  [unwired: 9 in]
        n545 = global read "GlobalVariables.vi" "LastUseiRF"() -> (w1232:T35)
        n546 = call "setLaguerreOrder.vi"("error in (no error)"=w1250, "LaguerreOrder"=u32 12, "LaguerreDeconClass in"=w1230) -> ("error out"=w1251:errorcluster, "LaguerreDeconClass out"=w1252:refnum<class "LaguerreDeconEngineClass.lvclass">)  [unwired: 7 in]
        n547 = Unbundle By Name(w1249) -> ("min record length"=w1248:i32)
        n548 = Unbundle By Name(w1232) -> ("Ch3 iRF"=w1231:dbl[])
        n549 = call "setDataLength.vi"("error in (no error)"=w1251, "dataLength"=w1248, "LaguerreDeconClass in"=w1252) -> ("error out"=w1247:errorcluster, "LaguerreDeconClass out"=w1246:refnum<class "LaguerreDeconEngineClass.lvclass">)  [unwired: 7 in]
        n550 = call "setIRF.vi"("error in (no error)"=w1247, "iRF"=w1231, "LaguerreDeconClass in"=w1246) -> ("error out"=w1244:errorcluster, "LaguerreDeconClass out"=w1245:refnum<class "LaguerreDeconEngineClass.lvclass">)  [unwired: 7 in]
        n551 = call "computeAlpha.vi"("error in (no error)"=w1244, "LaguerreDeconClass in"=w1245) -> ("error out"=w1242:errorcluster, "LaguerreDeconClass out"=w1243:refnum<class "LaguerreDeconEngineClass.lvclass">)  [unwired: 8 in]
        n552 = call "dataInitilize.vi"("error in (no error)"=w1242, "LaguerreDeconClass in"=w1243) -> ("error out"=w1240:errorcluster, "LaguerreDeconClass out"=w1241:refnum<class "LaguerreDeconEngineClass.lvclass">)  [unwired: 8 in]
        n553 = call "computeDeconMatrix.vi"("error in (no error)"=w1240, "LaguerreDeconClass in"=w1241) -> ("error out"=w1236:errorcluster, "LaguerreDeconClass out"=w1238:refnum<class "LaguerreDeconEngineClass.lvclass">)  [unwired: 8 in]
        n554 = call "Ch3DeconEngineFGV.vi"("Error In"=w1236, "action(read)"=enum16{"write", "read"}."write" ("action"), "Ch3DeconEngine in"=w1238) -> ("Error Out"=w1235:errorcluster)  [unwired: 7 in, 1 out]
        n555 = call <vilib>:"Add State(s) to Queue__JKI_lib_State_Machine.vi"("State(s) in (\"\")"=w1255) -> ("States Out"=w1254:string)  [unwired: 14 in]
      }
      frame "---------- Digitizer ----------" {
        # "Template Separator\n(You can make a copy of, or modify, this frame)"
        n556 = call <vilib>:"Add State(s) to Queue__JKI_lib_State_Machine.vi"("State(s) in (\"\")"=w1260) -> ("States Out"=w1259:string)  [unwired: 14 in]
      }
      frame "Digitizer: Initialize" {
        # "Initialize digitizer.\nInitialize both digitizer and update status."
        n557 = Unbundle By Name(w1270) -> ("SysConfigCluster.Ch1Enable?"=w1275:bool, "SysConfigCluster.Ch2Enable?"=w1274:bool, "SysConfigCluster.Ch3Enable?"=w1272:bool)
        n558 = call "FLImDAQ_FGV.vi"("error in (no error)"=w1266) -> ("error out"=w1265:errorcluster, "Read data"=w1264:T5)  [unwired: 9 in]
        n559 = property on="Digitizer" class="Bool (strict)"("Blinking"=TRUE) -> ()  [unwired: 2 in, 2 out]
        n560 = Unbundle By Name(w1264) -> ("Digitizer 1"=w1263:refnum<k15>, "Digitizer 2"=w1262:refnum<k15>)
        n561 = Or(x=w1275, y=w1274) -> (x .or. y?=w1273:bool)
        n562 = case shown="True" w1272 {
          tunnel: w1265 -> [w1278 w1280]
          tunnel: [w1278 w1282] -> w1268
          tunnel: w1262 -> [_ w1281]
          frame False {
          }
          frame True {
            n563 = call <instrlib>:"niScope Initialize.vi"("resource name"=w1281, "reset device"=FALSE, "error in"=w1280) -> ("error out"=w1282:errorcluster)  [unwired: 11 in, 1 out]
          }
        }
        n564 = case shown="True" w1273 {
          tunnel: w1265 -> [w1283 w1285]
          tunnel: [w1283 w1287] -> w1269
          tunnel: w1263 -> [_ w1286]
          frame False {
          }
          frame True {
            n565 = call <instrlib>:"niScope Initialize.vi"("resource name"=w1286, "reset device"=FALSE, "error in"=w1285) -> ("error out"=w1287:errorcluster)  [unwired: 11 in, 1 out]
          }
        }
        n566 = Merge Errors(w1269, w1268) -> (w1267:errorcluster)
        n567 = call <vilib>:"Add State(s) to Queue__JKI_lib_State_Machine.vi"("State(s) in (\"\")"=w1277) -> ("States Out"=w1276:string)  [unwired: 14 in]
      }
      frame "Digitizer: Config" {
        w1288 = enum16{"Write", "Read"}."Read" ("Operation")
        # "Synchronize is taking time ~3s."
        # "Config  digitizer\nCall subVi to config digitizer"
        n568 = call "FLImDAQ_FGV.vi"() -> ("Read data"=w1306:T5)  [unwired: 10 in, 1 out]
        n569 = Unbundle By Name(w1315) -> ("SysConfigCluster.Ch1Enable?"=w1323:bool, "SysConfigCluster.Ch2Enable?"=w1322:bool, "SysConfigCluster.Ch3Enable?"=w1320:bool, "FLImDAQ"=w1317:T27)
        n570 = Unbundle By Name(w1306) -> ("Digitizer 1"=w1309:refnum<k15>, "Digitizer 2"=w1308:refnum<k15>)
        n571 = property on="Digitizer" class="Bool (strict)"(error in=w1310, "Blinking"=TRUE) -> (error out=w1311:errorcluster)  [unwired: 1 in, 1 out]
        n572 = Or(x=w1323, y=w1322) -> (x .or. y?=w1321:bool)
        n573 = case shown="True" w1321 {
          tunnel: w1317 -> [_ w1336]
          tunnel: w1311 -> [w1332 w1335]
          tunnel: [w1332 w1334] -> w1318
          tunnel: w1309 -> [_ w1333]
          frame False {
          }
          frame True {
            n574 = call "DigitizerConfig.vi"("error in (no error)"=w1335, "FLImDAQ"=w1336, "IVI Refnum in"=w1333) -> ("error out"=w1334:errorcluster)  [unwired: 7 in, 1 out]
          }
        }
        n575 = case shown="True" w1320 {
          tunnel: w1317 -> [_ w1331]
          tunnel: w1318 -> [w1326 w1330]
          tunnel: [w1326 w1329] -> w1294
          tunnel: w1308 -> [_ w1327]
          frame False {
          }
          frame True {
            n576 = call "DigitizerConfig.vi"("Config Trigger? (T)"=FALSE ("Config Trigge(T)r:"), "error in (no error)"=w1330, "FLImDAQ"=w1331, "IVI Refnum in"=w1327) -> ("error out"=w1329:errorcluster)  [unwired: 6 in, 1 out]
          }
        }
        n577 = call "Digitizer1_FGV.vi"("error in (no error)"=w1294, "Operation (Read)"=w1288) -> ("error out"=w1304:errorcluster, "Read data"=w1305:refnum<k15>)  [unwired: 8 in]
        n578 = call <instrlib>:"niScope Get Session Reference.vi"("instrument handle"=w1305, "error in"=w1304) -> ("session reference"=w1298:refnum<k20>, "error out"=w1296:errorcluster)  [unwired: 11 in, 1 out]
        n579 = call "Digitizer2_FGV.vi"("error in (no error)"=w1296, "Operation (Read)"=w1288) -> ("error out"=w1302:errorcluster, "Read data"=w1303:refnum<k15>)  [unwired: 8 in]
        n580 = call <instrlib>:"niScope Get Session Reference.vi"("instrument handle"=w1303, "error in"=w1302) -> ("session reference"=w1297:refnum<k20>, "error out"=w1295:errorcluster)  [unwired: 11 in, 1 out]
        n581 = Build Array(w1298, w1297) -> (w1301:refnum<k20>[])
        n582 = call <instrlib>:"niTClk Configure For Homogeneous Triggers.vi"("error in (no error)"=w1295, "sessions"=w1301) -> ("error out"=w1300:errorcluster, "sessions out"=w1299:refnum<k20>[])  [unwired: 8 in]
        n583 = call <instrlib>:"niTClk Synchronize.vi"("error in (no error)"=w1300, "sessions"=w1299) -> ("error out"=w1293:errorcluster, "sessions out"=w1290:refnum<k20>[])  [unwired: 8 in]
        n584 = call <userlib>:"Wait (ms)__ogtk.vi"("error in (no error)"=w1293, "milliseconds to wait"=u32 1500) -> ("error out"=w1292:errorcluster)  [unwired: 8 in, 1 out]
        n585 = Unbundle By Name(w1292) -> ("status"=w1314:bool)
        n586 = Not(x=w1314) -> (.not. x?=w1313:bool)
        n587 = Bundle By Name(cluster=w1315, "System Status.Digitizer"=w1313, "niTClk sessions"=w1290) -> (w1316:T20)
        n588 = property on="Digitizer" class="Bool (strict)"(error in=w1292, "Blinking"=FALSE) -> (error out=w1307:errorcluster)  [unwired: 1 in, 1 out]
        n589 = call <vilib>:"Add State(s) to Queue__JKI_lib_State_Machine.vi"("State(s) in (\"\")"=w1325) -> ("States Out"=w1324:string)  [unwired: 14 in]
      }
      frame "Digitizer: Start" {
        # "send trigger to start acquisition loop"
        # "initilize aquisition"
        # "Template Separator\n(You can make a copy of, or modify, this frame)"
        n590 = Unbundle By Name(w1344) -> ("niTClk sessions"=w1343:refnum<k20>[])
        n591 = call <instrlib>:"niTClk Initiate.vi"("error in (no error)"=w1337, "sessions"=w1343) -> ("error out"=w1339:errorcluster)  [unwired: 8 in, 1 out]
        n592 = Generate User Event(priority (normal)=usereventprio."high priority", user event=w1340, event data cluster=TRUE ("event data"), error in=w1339) -> (error out=w1338:errorcluster)  [unwired: 1 out]
        n593 = call <vilib>:"Add State(s) to Queue__JKI_lib_State_Machine.vi"("State(s) in (\"\")"=w1347) -> ("States Out"=w1346:string)  [unwired: 14 in]
      }
      frame "Digitizer: Abort" {
        # "Template Separator\n(You can make a copy of, or modify, this frame)"
        n594 = call "Digitizer1_FGV.vi"("error in (no error)"=w1351, "Operation (Read)"=enum16{"Write", "Read"}."Read" ("Operation")) -> ("error out"=w1358:errorcluster, "Read data"=w1355:refnum<k15>)  [unwired: 8 in]
        n595 = call "Digitizer2_FGV.vi"("error in (no error)"=w1351, "Operation (Read)"=enum16{"Write", "Read"}."Read" ("Operation")) -> ("error out"=w1354:errorcluster, "Read data"=w1356:refnum<k15>)  [unwired: 8 in]
        n596 = Bundle By Name(cluster=w1348, "SysRunning?"=FALSE ("System Status")) -> (w1349:T20)
        n597 = call <instrlib>:"niScope Abort.vi"("instrument handle"=w1355, "error in"=w1358) -> ("error out"=w1360:errorcluster)  [unwired: 12 in, 1 out]
        n598 = call <instrlib>:"niScope Abort.vi"("instrument handle"=w1356, "error in"=w1354) -> ("error out"=w1359:errorcluster)  [unwired: 12 in, 1 out]
        n599 = Merge Errors(w1360, w1359) -> (w1352:errorcluster)
        n600 = call <vilib>:"Add State(s) to Queue__JKI_lib_State_Machine.vi"("State(s) in (\"\")"=w1363) -> ("States Out"=w1362:string)  [unwired: 14 in]
      }
      frame "Digitizer: checkTemp" {
        w1367 = enum16{"Write", "Read"}."Read" ("Operation")
        # "Template Separator\n(You can make a copy of, or modify, this frame)"
        n601 = call "Digitizer1_FGV.vi"("Operation (Read)"=w1367) -> ("error out"=w1369:errorcluster, "Read data"=w1370:refnum<k15>)  [unwired: 9 in]
        n602 = call "Digitizer2_FGV.vi"("Operation (Read)"=w1367) -> ("error out"=w1365:errorcluster, "Read data"=w1366:refnum<k15>)  [unwired: 9 in]
        n603 = property on="Property Node" class="niScope"(reference=w1370, error in=w1369) -> ("Device Temperature"=→"Dig1 Temp":dbl)  [unwired: 2 out]
        n604 = property on="Property Node" class="niScope"(reference=w1366, error in=w1365) -> ("Device Temperature"=→"Dig2 Temp":dbl)  [unwired: 2 out]
        n605 = call <vilib>:"Add State(s) to Queue__JKI_lib_State_Machine.vi"("State(s) in (\"\")"=w1375) -> ("States Out"=w1374:string)  [unwired: 14 in]
      }
      frame "Digitizer: Close" {
        # "Close Digitizer"
        n606 = call "Digitizer1_FGV.vi"("error in (no error)"=w1381, "Operation (Read)"=enum16{"Write", "Read"}."Read" ("Operation")) -> ("error out"=w1383:errorcluster, "Read data"=w1387:refnum<k15>)  [unwired: 8 in]
        n607 = call "Digitizer2_FGV.vi"("error in (no error)"=w1381, "Operation (Read)"=enum16{"Write", "Read"}."Read" ("Operation")) -> ("error out"=w1382:errorcluster, "Read data"=w1385:refnum<k15>)  [unwired: 8 in]
        n608 = call <instrlib>:"niScope Close.vi"("instrument handle"=w1387, "error in"=w1383) -> ("error out"=w1380:errorcluster)  [unwired: 13 in]
        n609 = call <instrlib>:"niScope Close.vi"("instrument handle"=w1385, "error in"=w1382) -> ("error out"=w1379:errorcluster)  [unwired: 13 in]
        n610 = Merge Errors(w1380, w1379) -> (w1378:errorcluster)
        n611 = Unbundle By Name(w1378) -> ("status"=w1377:bool)
        n612 = Bundle By Name(cluster=w1388, "System Status.Digitizer"=w1377) -> (w1389:T20)
        n613 = call <vilib>:"Add State(s) to Queue__JKI_lib_State_Machine.vi"("State(s) in (\"\")"=w1391) -> ("States Out"=w1390:string)  [unwired: 14 in]
      }
      frame "---------- LabJack ----------" {
        # "Template Separator\n(You can make a copy of, or modify, this frame)"
        n614 = call <vilib>:"Add State(s) to Queue__JKI_lib_State_Machine.vi"("State(s) in (\"\")"=w1396) -> ("States Out"=w1395:string)  [unwired: 14 in]
      }
      frame "LabJack: checkPedal" {
        # "Template Separator\n(You can make a copy of, or modify, this frame)"
        n615 = Unbundle By Name(w1397) -> ("LJ Pinout.Foot Pedal"=w1401:string)
        n616 = call "LabJack_FGV.vi"("Operation(Read)"=enum16{"Write", "Read"}."Read" ("Operation"), "error in (no error)"=w1399) -> ("error out"=w1403:errorcluster, "Read data"=w1404:i32)  [unwired: 8 in]
        n617 = call "LJM_eReadName.vi"("Handle In"=w1404, "Name"=w1401, "error in"=w1403) -> ("Value"=w1402:dbl, "error out"=w1400:errorcluster)  [unwired: 10 in, 1 out]
        n618 = case shown="1" w1402 {
          tunnel: w1397 -> [w1409 w1412]
          tunnel: [w1409 w1410] -> w1398
          frame 0, Default {
          }
          frame 1 {
            # "If Pedal pressed"
            n619 = Tick Count (ms)() -> (millisecond timer value=w1416:u32)
            n620 = Unbundle By Name(w1412) -> ("Last Trigger"=w1411:u32)
            n621 = Subtract(x=w1416, y=w1411) -> (x-y=w1415:u32)
            n622 = Greater Or Equal?(x=w1415, y=u32 2000) -> (x >= y?=w1413:bool)
            n623 = case shown="True" w1413 {
              tunnel: w1412 -> [w1417 w1418]
              tunnel: w1411 -> [_ _]
              tunnel: [w1417 w1419] -> w1410
              frame False {
              }
              frame True {
                n624 = Tick Count (ms)() -> (millisecond timer value=w1420:u32)
                n625 = Unbundle By Name(w1418) -> ("SysRunning?"=w1421:bool)
                n626 = case shown="False" w1421 {
                  frame False {
                    n627 = property on="StartButton" class="Bool (strict)"("Val(Sgnl)"=TRUE ("Value (Signaling)")) -> ()  [unwired: 2 in, 2 out]
                  }
                  frame True {
                    n628 = property on="StopButton" class="Bool (strict)"("Val(Sgnl)"=TRUE ("Value (Signaling)")) -> ()  [unwired: 2 in, 2 out]
                  }
                }
                n629 = Bundle By Name(cluster=w1418, "Last Trigger"=w1420) -> (w1419:T20)
              }
            }
          }
        }
        n630 = call <vilib>:"Add State(s) to Queue__JKI_lib_State_Machine.vi"("State(s) in (\"\")"=w1408) -> ("States Out"=w1407:string)  [unwired: 14 in]
      }
      frame "LabJack: ZeroV" {
        # "Just Zero V\nDO not update FGV and front panel\nWIll resume from last V"
        # "set bias to 0"
        # "Zero APD bias\n(You can make a copy of, or modify, this frame)"
        n631 = Unbundle By Name(w1426) -> ("LJ Pinout.Ch1 Bias"=w1431:string, "LJ Pinout.Ch2 Bias"=w1430:string, "LJ Pinout.Ch3 Bias"=w1429:string)
        n632 = Build Array(w1431, w1430, w1429) -> (w1428:string[])
        n633 = call "LabJack_FGV.vi"("Operation(Read)"=enum16{"Write", "Read"}."Read" ("Operation"), "error in (no error)"=w1425) -> ("error out"=w1432:errorcluster, "Read data"=w1433:i32)  [unwired: 8 in]
        n634 = call "LJM_eWriteNames.vi"("Handle In"=w1433, "aNames"=w1428, "aValuesIn"=dbl[] [0.0, 0.0, 0.0], "error in"=w1432) -> ("error out"=w1424:errorcluster)  [unwired: 9 in, 2 out]
        n635 = call <vilib>:"Add State(s) to Queue__JKI_lib_State_Machine.vi"("State(s) in (\"\")"=w1437) -> ("States Out"=w1436:string)  [unwired: 14 in]
      }
      frame "LabJack: SetV" {
        # "set bias to user specifid"
        # "Zero APD bias\n(You can make a copy of, or modify, this frame)"
        n636 = Unbundle By Name(w1451) -> ("LJ Pinout.Ch1 Bias"=w1455:string, "LJ Pinout.Ch2 Bias"=w1454:string, "LJ Pinout.Ch3 Bias"=w1453:string)
        n637 = call "V1FGV.vi"("Error In"=w1450, "action (write)"=enum16{"write", "read"}."read") -> ("Error Out"=w1449:errorcluster, "V1 out"=w1443:dbl)  [unwired: 8 in]
        n638 = local write "V 1"(w1443) -> ()
        n639 = call "V2FGV.vi"("Error In"=w1449, "action(write)"=enum16{"write", "read"}."read") -> ("Error Out"=w1448:errorcluster, "V2 out"=w1442:dbl)  [unwired: 8 in]
        n640 = local write "V 2"(w1442) -> ()
        n641 = Build Array(w1455, w1454, w1453) -> (w1452:string[])
        n642 = call "V3FGV.vi"("Error In"=w1448, "action(write)"=enum16{"write", "read"}."read" ("action(read)")) -> ("Error Out"=w1445:errorcluster, "V3 out"=w1441:dbl)  [unwired: 8 in]
        n643 = local write "V 3"(w1441) -> ()
        n644 = Build Array(w1443, w1442, w1441) -> (w1444:dbl[])
        n645 = call "LabJack_FGV.vi"("Operation(Read)"=enum16{"Write", "Read"}."Read" ("Operation"), "error in (no error)"=w1450) -> ("error out"=w1456:errorcluster, "Read data"=w1457:i32)  [unwired: 8 in]
        n646 = call "LJM_eWriteNames.vi"("Handle In"=w1457, "aNames"=w1452, "aValuesIn"=w1444, "error in"=w1456) -> ("error out"=w1446:errorcluster)  [unwired: 9 in, 2 out]
        n647 = Merge Errors(w1445, w1446) -> (w1447:errorcluster)
        n648 = call <vilib>:"Add State(s) to Queue__JKI_lib_State_Machine.vi"("State(s) in (\"\")"=w1461) -> ("States Out"=w1460:string)  [unwired: 14 in]
      }
      frame "LabJack: Open" {
        # "Initialize LabJack T7\nEstablish connection and initialize pins"
        n649 = call "LJ_Open.vi"("error in"=w1470) -> ("error out"=w1467:errorcluster, "Success?"=w1468:bool, "Handle Out"=w1462:i32)  [unwired: 8 in]
        n650 = call "LabJack_FGV.vi"("Operation(Read)"=enum16{"Write", "Read"}."Write" ("Operation"), "error in (no error)"=w1467, "Write data"=w1462) -> ("error out"=w1464:errorcluster)  [unwired: 7 in, 1 out]
        n651 = Bundle By Name(cluster=w1465, "System Status.Labjack"=w1468) -> (w1469:T20)
        n652 = call <vilib>:"Add State(s) to Queue__JKI_lib_State_Machine.vi"("State(s) in (\"\")"=w1472) -> ("States Out"=w1471:string)  [unwired: 14 in]
      }
      frame "LabJack: SetDefaultSub" {
        w1492 = "_EF_ENABLE" ("string")
        # "1. Disable PWM\n2. Set all V to 0\n3. Set 355 relay to open\n4. Set LED to off"
        # "read once to set DIO to input"
        # "set all initila V to 0. Set footpedal to input. Set PWM to low. Set laser relay to open. Set LEDs to yellow."
        # "Set Labjack to correct input and output state and initial values"
        n653 = Unbundle By Name(w1489) -> ("LJ Pinout.355 PWM"=w1494:string, "LJ Pinout.AimingBeam PWM"=w1493:string, "LJ Pinout.Ch1 Bias"=w1501:string, "LJ Pinout.Ch2 Bias"=w1507:string, "LJ Pinout.Ch3 Bias"=w1506:string, "LJ Pinout.Laser Start/Stop"=w1505:string, "LJ Pinout.Red LED"=w1504:string, "LJ Pinout.Green LED"=w1503:string)
        n654 = call "V1FGV.vi"("Error In"=w1482, "action (write)"=enum16{"write", "read"}."write" ("action"), "V1 in"=0.0) -> ("Error Out"=w1483:errorcluster, "V1 out"=w1475:dbl)  [unwired: 7 in]
        n655 = call "LabJack_FGV.vi"("Operation(Read)"=enum16{"Write", "Read"}."Read" ("Operation"), "error in (no error)"=w1482) -> ("error out"=w1497:errorcluster, "Read data"=w1498:i32)  [unwired: 8 in]
        n656 = local write "V 1"(w1475) -> ()
        n657 = call "V2FGV.vi"("Error In"=w1483, "action(write)"=enum16{"write", "read"}."write" ("action"), "V2 in"=0.0) -> ("Error Out"=w1479:errorcluster, "V2 out"=w1474:dbl)  [unwired: 7 in]
        n658 = Concatenate Strings(w1494, w1492) -> (w1491:string)
        n659 = Concatenate Strings(w1493, w1492) -> (w1490:string)
        n660 = local write "V 2"(w1474) -> ()
        n661 = call "V3FGV.vi"("Error In"=w1479, "action(write)"=enum16{"write", "read"}."write" ("action"), "V3 in"=0.0) -> ("Error Out"=w1476:errorcluster, "V3 out"=w1473:dbl)  [unwired: 7 in]
        n662 = Build Array(w1491, w1490, w1501, w1507, w1506, w1505, w1504, w1503) -> (w1502:string[])
        n663 = local write "V 3"(w1473) -> ()
        n664 = Unbundle By Name(w1489) -> ("LJ Pinout.Foot Pedal"=w1488:string)
        n665 = call "LJM_eWriteNames.vi"("Handle In"=w1498, "aNames"=w1502, "aValuesIn"=dbl[] [0.0, 0.0, 0.0, 0.0, 0.0, 0.0, 0.0, 0.0], "error in"=w1497) -> ("Handle Out"=w1496:i32, "error out"=w1495:errorcluster)  [unwired: 9 in, 1 out]
        n666 = call "LJM_eReadName.vi"("Handle In"=w1496, "Name"=w1488, "error in"=w1495) -> ("error out"=w1478:errorcluster)  [unwired: 10 in, 2 out]
        n667 = Merge Errors(w1478, w1476) -> (w1477:errorcluster)
        n668 = call <vilib>:"Add State(s) to Queue__JKI_lib_State_Machine.vi"("State(s) in (\"\")"=w1510) -> ("States Out"=w1509:string)  [unwired: 14 in]
      }
      frame "LabJack: FootPedalConfig" {
        # "Setup footPedal\n(You can make a copy of, or modify, this frame)"
        n669 = call "LabJack_FGV.vi"("Operation(Read)"=enum16{"Write", "Read"}."Read" ("Operation"), "error in (no error)"=w1512) -> ("error out"=w1516:errorcluster, "Read data"=w1517:i32)  [unwired: 8 in]
        n670 = call "LJM_eWriteName.vi"("Handle In"=w1517, "Name"="DIO15", "Value"=1.0, "error in"=w1516) -> ("error out"=w1513:errorcluster)  [unwired: 10 in, 1 out]
        n671 = call <vilib>:"Add State(s) to Queue__JKI_lib_State_Machine.vi"("State(s) in (\"\")"=w1521) -> ("States Out"=w1520:string)  [unwired: 14 in]
      }
      frame "LabJack: SetDefaultAndClose" {
        # "Template Separator\n(You can make a copy of, or modify, this frame)"
        n672 = call <vilib>:"Add State(s) to Queue__JKI_lib_State_Machine.vi"("State(s) in Front (\"\")"="LabJack: SetDefaultSub\nLabJack: Close" ("State(s) in Front (\"\")"), "State(s) in (\"\")"=w1527) -> ("States Out"=w1526:string)  [unwired: 13 in]
      }
      frame "LabJack: Close" {
        # "Close LabJack Refnum"
        n673 = call "LabJack_FGV.vi"("Operation(Read)"=enum16{"Write", "Read"}."Read" ("Operation"), "error in (no error)"=w1533) -> ("error out"=w1528:errorcluster, "Read data"=w1529:i32)  [unwired: 8 in]
        n674 = Bundle By Name(cluster=w1531, "System Status.Labjack"=FALSE ("System Status.Gain Control")) -> (w1534:T20)
        n675 = call "LJM_Close.vi"("error in"=w1528, "Handle"=w1529) -> ("error out"=w1536:errorcluster)  [unwired: 9 in]
        n676 = call <vilib>:"Add State(s) to Queue__JKI_lib_State_Machine.vi"("State(s) in (\"\")"=w1538) -> ("States Out"=w1537:string)  [unwired: 14 in]
      }
      frame "LabJack: Interlock enable/disable" {
        w1547 = i8 0  # int8
        # "[Covers: REQ8]"
        # "Interlock enable/disable\n(Usage: \"LabJack: Interlock enable/disable >> 1|0\")"
        n677 = Fract/Exp String To Number(string=w1548, default (0 dbl)=w1547) -> (number=w1544:i8)  [unwired: 2 in, 1 out]
        n678 = Unbundle By Name(w1546) -> ("LJ Pinout.Interlock"=w1545:string)
        n679 = call "LabJack_FGV.vi"("Operation(Read)"=enum16{"Write", "Read"}."Read" ("Operation")) -> ("Read data"=w1542:i32)  [unwired: 9 in, 1 out]
        n680 = call "LJM_eWriteName.vi"("Handle In"=w1542, "Name"=w1545, "Value"=w1544, "error in"=w1543) -> ("error out"=w1540:errorcluster)  [unwired: 10 in, 1 out]
        n681 = call <vilib>:"Add State(s) to Queue__JKI_lib_State_Machine.vi"("State(s) in (\"\")"=w1550) -> ("States Out"=w1549:string)  [unwired: 14 in]
      }
      frame "LabJack: 355_PWM_Config" {
        w1552 = 0.0 ("element")
        w1572 = "DIO_EF_CLOCK1_ENABLE"
        # "Config PWM frequency"
        n682 = Unbundle By Name(w1564) -> ("LJ Pinout.355 PWM"=w1571:string)
        n683 = Unbundle By Name(w1564) -> ("355 PWM setting.DIO_EF_CLOCK1_DIVISOR"=w1563:i16, "355 PWM setting.DIO_EF_CLOCK1_ROLL_VALUE"=w1562:i32, "355 PWM setting.DIO#_EF_INDEX"=w1559:i16, "355 PWM setting.DIO#_EF_OPTIONS"=w1558:i16, "355 PWM setting.DIO#_EF_CONFIG_A"=w1557:i32)
        n684 = Concatenate Strings(w1571, "_EF_ENABLE" ("string")) -> (w1567:string)
        n685 = Concatenate Strings(w1571, "_EF_INDEX") -> (w1570:string)
        n686 = Concatenate Strings(w1571, "_EF_OPTIONS") -> (w1569:string)
        n687 = Concatenate Strings(w1571, "_EF_CONFIG_A") -> (w1568:string)
        n688 = call "LabJack_FGV.vi"("Operation(Read)"=enum16{"Write", "Read"}."Read" ("Operation")) -> ("Read data"=w1565:i32)  [unwired: 9 in, 1 out]
        n689 = Build Array(w1552, w1552, w1563, w1562, 1.0 ("element"), 0.0 ("element"), w1559, w1558, w1557) -> (w1556:dbl[])
        n690 = Build Array("DIO_EF_CLOCK0_ENABLE", w1572, "DIO_EF_CLOCK1_DIVISOR", "DIO_EF_CLOCK1_ROLL_VALUE", w1572, w1567, w1570, w1569, w1568) -> (w1566:string[])
        n691 = call "LJM_eWriteNames.vi"("Handle In"=w1565, "aNames"=w1566, "aValuesIn"=w1556, "error in"=w1554) -> ("error out"=w1555:errorcluster)  [unwired: 9 in, 2 out]
        n692 = call <vilib>:"Add State(s) to Queue__JKI_lib_State_Machine.vi"("State(s) in (\"\")"=w1581) -> ("States Out"=w1580:string)  [unwired: 14 in]
      }
      frame "LabJack: 355_PWM_Start" {
        # "Template Separator\n(You can make a copy of, or modify, this frame)"
        n693 = Unbundle By Name(w1589) -> ("LJ Pinout.355 PWM"=w1588:string)
        n694 = call "LabJack_FGV.vi"("Operation(Read)"=enum16{"Write", "Read"}."Read" ("Operation"), "error in (no error)"=w1583) -> ("error out"=w1590:errorcluster, "Read data"=w1591:i32)  [unwired: 8 in]
        n695 = Concatenate Strings(w1588, "_EF_ENABLE" ("string")) -> (w1586:string)
        n696 = call "LJM_eWriteName.vi"("Handle In"=w1591, "Name"=w1586, "Value"=1.0, "error in"=w1590) -> ("error out"=w1584:errorcluster)  [unwired: 10 in, 1 out]
        n697 = call <vilib>:"Add State(s) to Queue__JKI_lib_State_Machine.vi"("State(s) in (\"\")"=w1594) -> ("States Out"=w1593:string)  [unwired: 14 in]
      }
      frame "LabJack: 355_PWM_Stop" {
        # "Template Separator\n(You can make a copy of, or modify, this frame)"
        n698 = Unbundle By Name(w1600) -> ("LJ Pinout.355 PWM"=w1604:string)
        n699 = call "LabJack_FGV.vi"("Operation(Read)"=enum16{"Write", "Read"}."Read" ("Operation"), "error in (no error)"=w1599) -> ("error out"=w1605:errorcluster, "Read data"=w1597:i32)  [unwired: 8 in]
        n700 = Concatenate Strings(w1604, "_EF_ENABLE" ("string")) -> (w1602:string)
        n701 = call "LJM_eWriteName.vi"("Handle In"=w1597, "Name"=w1602, "Value"=0.0, "error in"=w1605) -> ("error out"=w1596:errorcluster)  [unwired: 10 in, 1 out]
        n702 = local write "355nm Laser toggle"(FALSE ("355nm Laser toggle")) -> ()
        n703 = call <vilib>:"Add State(s) to Queue__JKI_lib_State_Machine.vi"("State(s) in (\"\")"=w1608) -> ("States Out"=w1607:string)  [unwired: 14 in]
      }
      frame "LabJack: AB_Start" {
        # "Aiming Beam Start\n(Based on aimging beam frequency, set LabJack pin)"
        n704 = Unbundle By Name(w1618) -> ("AB Cluster.Freq"=w1610:i32, "LJ Pinout.AimingBeam PWM"=w1617:string)
        n705 = Greater Than 0?(x=w1610) -> (x > 0?=w1609:bool)
        n706 = case shown="False" w1609 {
          tunnel: w1617 -> [w1624 w1627]
          tunnel: [w1624 w1625] -> w1616
          frame False {
            # "if 0 freq, set PWM pin"
          }
          frame True {
            # "if non zero freq, set PWM enable"
            n707 = Concatenate Strings(w1627, "_EF_ENABLE" ("string")) -> (w1625:string)
          }
        }
        n708 = call "LabJack_FGV.vi"("Operation(Read)"=enum16{"Write", "Read"}."Read" ("Operation"), "error in (no error)"=w1613) -> ("error out"=w1619:errorcluster, "Read data"=w1620:i32)  [unwired: 8 in]
        n709 = call "LJM_eWriteName.vi"("Handle In"=w1620, "Name"=w1616, "Value"=1.0, "error in"=w1619) -> ("error out"=w1614:errorcluster)  [unwired: 10 in, 1 out]
        n710 = local write "Aiming beam toggle"(TRUE ("Aiming beam toggle")) -> ()
        n711 = call <vilib>:"Add State(s) to Queue__JKI_lib_State_Machine.vi"("State(s) in (\"\")"=w1623) -> ("States Out"=w1622:string)  [unwired: 14 in]
      }
      frame "LabJack: AB_Stop" {
        # "Aiming Beam Stop\n(Based on aiming beam frequency, set LabJack pin low)"
        n712 = Unbundle By Name(w1635) -> ("AB Cluster.Freq"=w1630:i32, "LJ Pinout.AimingBeam PWM"=w1637:string)
        n713 = Greater Than 0?(x=w1630) -> (x > 0?=w1629:bool)
        n714 = case shown="False" w1629 {
          tunnel: w1637 -> [w1643 w1646]
          tunnel: [w1643 w1644] -> w1628
          frame False {
          }
          frame True {
            n715 = Concatenate Strings(w1646, "_EF_ENABLE" ("string")) -> (w1644:string)
          }
        }
        n716 = call "LabJack_FGV.vi"("Operation(Read)"=enum16{"Write", "Read"}."Read" ("Operation"), "error in (no error)"=w1633) -> ("error out"=w1638:errorcluster, "Read data"=w1639:i32)  [unwired: 8 in]
        n717 = call "LJM_eWriteName.vi"("Handle In"=w1639, "Name"=w1628, "Value"=0.0, "error in"=w1638) -> ("error out"=w1634:errorcluster)  [unwired: 10 in, 1 out]
        n718 = local write "Aiming beam toggle"(FALSE ("Aiming beam toggle")) -> ()
        n719 = call <vilib>:"Add State(s) to Queue__JKI_lib_State_Machine.vi"("State(s) in (\"\")"=w1642) -> ("States Out"=w1641:string)  [unwired: 14 in]
      }
      frame "LabJack: AB_PWM_Config" {
        w1648 = 0.0 ("element")
        w1668 = "DIO_EF_CLOCK2_ENABLE"
        # "Config PWM frequency"
        n720 = Unbundle By Name(w1660) -> ("LJ Pinout.AimingBeam PWM"=w1667:string)
        n721 = Unbundle By Name(w1660) -> ("AB PWM setting.DIO_EF_CLOCK1_DIVISOR"=w1659:i16, "AB PWM setting.DIO_EF_CLOCK1_ROLL_VALUE"=w1658:i32, "AB PWM setting.DIO#_EF_INDEX"=w1655:i16, "AB PWM setting.DIO#_EF_OPTIONS"=w1654:i16, "AB PWM setting.DIO#_EF_CONFIG_A"=w1653:i32)
        n722 = Concatenate Strings(w1667, "_EF_ENABLE" ("string")) -> (w1663:string)
        n723 = Concatenate Strings(w1667, "_EF_INDEX") -> (w1666:string)
        n724 = Concatenate Strings(w1667, "_EF_OPTIONS") -> (w1665:string)
        n725 = Concatenate Strings(w1667, "_EF_CONFIG_A") -> (w1664:string)
        n726 = call "LabJack_FGV.vi"("Operation(Read)"=enum16{"Write", "Read"}."Read" ("Operation")) -> ("Read data"=w1661:i32)  [unwired: 9 in, 1 out]
        n727 = Build Array(w1648, w1648, w1659, w1658, 1.0 ("element"), 0.0 ("element"), w1655, w1654, w1653) -> (w1652:dbl[])
        n728 = Build Array("DIO_EF_CLOCK0_ENABLE", w1668, "DIO_EF_CLOCK2_DIVISOR", "DIO_EF_CLOCK2_ROLL_VALUE", w1668, w1663, w1666, w1665, w1664) -> (w1662:string[])
        n729 = call "LJM_eWriteNames.vi"("Handle In"=w1661, "aNames"=w1662, "aValuesIn"=w1652, "error in"=w1650) -> ("error out"=w1651:errorcluster)  [unwired: 9 in, 2 out]
        n730 = call <vilib>:"Add State(s) to Queue__JKI_lib_State_Machine.vi"("State(s) in (\"\")"=w1677) -> ("States Out"=w1676:string)  [unwired: 14 in]
      }
      frame "---------- LED ----------" {
        # "Template Separator\n(You can make a copy of, or modify, this frame)"
        n731 = call <vilib>:"Add State(s) to Queue__JKI_lib_State_Machine.vi"("State(s) in (\"\")"=w1682) -> ("States Out"=w1681:string)  [unwired: 14 in]
      }
      frame "LED: OpenVIRef" {
        # "Template Separator\n(You can make a copy of, or modify, this frame)"
        n732 = call <vilib>:"Application Directory.vi"() -> ("Application Directory"=w1687:path)
        n733 = Build Path(base path=w1687, name or relative path="SubVI") -> (appended path=w1685:path)
        n734 = Build Path(base path=w1685, name or relative path="LEDBreath.vi") -> (appended path=w1683:path)
        n735 = Open VI Reference(vi path=w1683, error in (no error)=w1688) -> (vi reference=w1690:refnum<vi>, error out=w1689:errorcluster)  [unwired: 4 in]
        n736 = Bundle By Name(cluster=w1691, "LED vi reference"=w1690) -> (w1692:T20)
        n737 = call <vilib>:"Add State(s) to Queue__JKI_lib_State_Machine.vi"("State(s) in (\"\")"=w1695) -> ("States Out"=w1694:string)  [unwired: 14 in]
      }
      frame "LED: CloseVIRef" {
        # "Template Separator\n(You can make a copy of, or modify, this frame)"
        n738 = Unbundle By Name(w1696) -> ("LED vi reference"=w1697:refnum<vi>)
        n739 = Close Reference(reference=w1697, error in (no error)=w1699) -> (error out=w1698:errorcluster)
        n740 = call <vilib>:"Add State(s) to Queue__JKI_lib_State_Machine.vi"("State(s) in (\"\")"=w1702) -> ("States Out"=w1701:string)  [unwired: 14 in]
      }
      frame "LED: BreathGreen" {
        w1703 = FALSE ("Wait Until Done")
        # "Breath system LED\n(LED: Breath >> True/False)"
        n741 = Unbundle By Name(w1711) -> ("LED vi reference"=w1710:refnum<vi>)
        n742 = invoke class="VI" method="Ctrl Val.Set"(reference=w1710, error in=w1708, "Control Name"="Color", "Value"=0) -> (reference out=w1707:refnum<vi>, error out=w1706:errorcluster)  [unwired: 1 in, 3 out]
        n743 = invoke on="Invoke Node" class="VI" method="Run VI"(reference=w1707, error in=w1706, "Wait until done"=w1703, "Auto Dispose Ref"=w1703) -> (error out=w1709:errorcluster)  [unwired: 1 in, 4 out]
        n744 = call <vilib>:"Add State(s) to Queue__JKI_lib_State_Machine.vi"("State(s) in (\"\")"=w1714) -> ("States Out"=w1713:string)  [unwired: 14 in]
      }
      frame "LED: BreathOrange" {
        w1715 = FALSE ("Wait Until Done")
        # "Breath system LED\n(LED: Breath >> True/False)"
        n745 = Unbundle By Name(w1723) -> ("LED vi reference"=w1722:refnum<vi>)
        n746 = invoke class="VI" method="Ctrl Val.Set"(reference=w1722, error in=w1720, "Control Name"="Color", "Value"=1) -> (reference out=w1719:refnum<vi>, error out=w1718:errorcluster)  [unwired: 1 in, 3 out]
        n747 = invoke on="Invoke Node" class="VI" method="Run VI"(reference=w1719, error in=w1718, "Wait until done"=w1715, "Auto Dispose Ref"=w1715) -> (error out=w1721:errorcluster)  [unwired: 1 in, 4 out]
        n748 = call <vilib>:"Add State(s) to Queue__JKI_lib_State_Machine.vi"("State(s) in (\"\")"=w1726) -> ("States Out"=w1725:string)  [unwired: 14 in]
      }
      frame "LED: BreathOff" {
        # "System LED Breath Off\n(Breath off, check VI status to make sure it is off)"
        n749 = Unbundle By Name(w1735) -> ("LED vi reference"=w1734:refnum<vi>)
        n750 = invoke on="Invoke Node" class="VI" method="Ctrl Val.Set"(reference=w1734, error in=w1732, "Control Name"="Stop", "Value"=TRUE) -> (reference out=w1727:refnum<vi>, error out=w1728:errorcluster)  [unwired: 1 in, 3 out]
        n751 = case shown="No Error" w1728 {
          selector: w1728 -> [w1740 _]
          tunnel: [w1739 errorcluster {"status"=FALSE, "code"=0, "source"=""} ("error IO")] -> w1733
          tunnel: ["" ("State(s) in Front (\"\")") "LED: BreathOff" ("State(s) in Front (\"\")")] -> w1731
          tunnel: w1727 -> [w1741 _]
          frame No Error {
            # "No error, wait for VI to stop"
            n752 = while {
              tunnel: w1741 -> [w1749]
              shift-right: [w1743] -> w1739
              shift-left: w1740 -> [w1748]
              stop <- w1745 stop-if-true
              # "continue check whether vi is running"
              n753 = property class="VI"(reference=w1749, error in=w1748) -> (error out=w1743:errorcluster, "Exec.State"=w1747:T17)  [unwired: 1 out]
              n754 = Wait (ms)(milliseconds to wait=u32 50) -> ()  [unwired: 1 out]
              n755 = Equal?(x=w1747, y=T17."Idle") -> (x = y?=w1745:bool)
            }
          }
          frame Error {
            # "try again when error"
          }
        }
        n756 = call <vilib>:"Add State(s) to Queue__JKI_lib_State_Machine.vi"("State(s) in Front (\"\")"=w1731, "State(s) in (\"\")"=w1738) -> ("States Out"=w1737:string)  [unwired: 13 in]
      }
      frame "LED: Off" {
        # "set LED to red"
        # "Template Separator\n(You can make a copy of, or modify, this frame)"
        n757 = Unbundle By Name(w1754) -> ("LJ Pinout.Red LED"=w1753:string, "LJ Pinout.Green LED"=w1752:string)
        n758 = call "LabJack_FGV.vi"("Operation(Read)"=enum16{"Write", "Read"}."Read" ("Operation"), "error in (no error)"=w1755) -> ("error out"=w1762:errorcluster, "Read data"=w1761:i32)  [unwired: 8 in]
        n759 = call "LJM_eWriteName.vi"("Handle In"=w1761, "Name"=w1753, "Value"=0.0, "error in"=w1762) -> ("Handle Out"=w1759:i32, "error out"=w1758:errorcluster)  [unwired: 10 in]
        n760 = call "LJM_eWriteName.vi"("Handle In"=w1759, "Name"=w1752, "Value"=0.0, "error in"=w1758) -> ("error out"=w1756:errorcluster)  [unwired: 10 in, 1 out]
        n761 = call <vilib>:"Add State(s) to Queue__JKI_lib_State_Machine.vi"("State(s) in (\"\")"=w1766) -> ("States Out"=w1765:string)  [unwired: 14 in]
      }
      frame "LED: Green" {
        # "set LED to green"
        # "Template Separator\n(You can make a copy of, or modify, this frame)"
        n762 = Unbundle By Name(w1770) -> ("LJ Pinout.Red LED"=w1768:string, "LJ Pinout.Green LED"=w1769:string)
        n763 = call "LabJack_FGV.vi"("Operation(Read)"=enum16{"Write", "Read"}."Read" ("Operation"), "error in (no error)"=w1772) -> ("error out"=w1778:errorcluster, "Read data"=w1777:i32)  [unwired: 8 in]
        n764 = call "LJM_eWriteName.vi"("Handle In"=w1777, "Name"=w1768, "Value"=0.0, "error in"=w1778) -> ("Handle Out"=w1775:i32, "error out"=w1774:errorcluster)  [unwired: 10 in]
        n765 = call "LJM_eWriteName.vi"("Handle In"=w1775, "Name"=w1769, "Value"=9.0, "error in"=w1774) -> ("error out"=w1771:errorcluster)  [unwired: 10 in, 1 out]
        n766 = call <vilib>:"Add State(s) to Queue__JKI_lib_State_Machine.vi"("State(s) in (\"\")"=w1781) -> ("States Out"=w1780:string)  [unwired: 14 in]
      }
      frame "---------- Queue ----------" {
        # "Template Separator\n(You can make a copy of, or modify, this frame)"
        n767 = call <vilib>:"Add State(s) to Queue__JKI_lib_State_Machine.vi"("State(s) in (\"\")"=w1786) -> ("States Out"=w1785:string)  [unwired: 14 in]
      }
      frame "Queue: Flash" {
        # "Clear queue contnet\n(clear queue content by flash it)"
        n768 = Flush Queue(queue=w1792, error in (no error)=w1791) -> (error out=w1790:errorcluster)  [unwired: 2 out]
        n769 = Flush Queue(queue=w1793, error in (no error)=w1790) -> (error out=w1788:errorcluster)  [unwired: 2 out]
        n770 = Flush Queue(queue=w1789, error in (no error)=w1788) -> (error out=w1787:errorcluster)  [unwired: 2 out]
        n771 = call <vilib>:"Add State(s) to Queue__JKI_lib_State_Machine.vi"("State(s) in (\"\")"=w1797) -> ("States Out"=w1796:string)  [unwired: 14 in]
      }
      frame "Queue: Destory" {
        # "Destory Data Queue\nDistory data queue ref so the aquisition loop stop"
        n772 = Release Queue(queue=w1803, error in (no error)=w1799) -> (error out=w1806:errorcluster)  [unwired: 1 in, 2 out]
        n773 = Release Queue(queue=w1802, error in (no error)=w1799) -> (error out=w1805:errorcluster)  [unwired: 1 in, 2 out]
        n774 = Release Queue(queue=w1800, error in (no error)=w1799) -> (error out=w1798:errorcluster)  [unwired: 1 in, 2 out]
        n775 = Merge Errors(w1806, w1805, w1798) -> (w1804:errorcluster)
        n776 = call <vilib>:"Simple Error Handler.vi"("error in (no error)"=w1804) -> ()  [unwired: 4 in, 5 out]
        n777 = call <vilib>:"Add State(s) to Queue__JKI_lib_State_Machine.vi"("State(s) in (\"\")"=w1809) -> ("States Out"=w1808:string)  [unwired: 14 in]
      }
      frame "---------- Run ----------" {
        # "Template Separator\n(You can make a copy of, or modify, this frame)"
        n778 = call <vilib>:"Add State(s) to Queue__JKI_lib_State_Machine.vi"("State(s) in (\"\")"=w1814) -> ("States Out"=w1813:string)  [unwired: 14 in]
      }
      frame "Run: CaliIncrement" {
        # "Increment Calibration #\n(You can make a copy of, or modify, this frame)"
        n779 = Unbundle By Name(w1816) -> ("IDs.Cali ID"=w1818:i8)
        n780 = Increment(x=w1818) -> (x+1=w1815:i8)
        n781 = Bundle By Name(cluster=w1816, "IDs.Cali ID"=w1815) -> (w1817:T20)
        n782 = call <vilib>:"Add State(s) to Queue__JKI_lib_State_Machine.vi"("State(s) in (\"\")"=w1822) -> ("States Out"=w1821:string)  [unwired: 14 in]
      }
      frame "Run: BGIncrement" {
        # "Increment BG #\n(You can make a copy of, or modify, this frame)"
        n783 = Unbundle By Name(w1823) -> ("IDs.BG ID"=w1826:i8)
        n784 = Increment(x=w1826) -> (x+1=w1825:i8)
        n785 = Bundle By Name(cluster=w1823, "IDs.BG ID"=w1825) -> (w1824:T20)
        n786 = call <vilib>:"Add State(s) to Queue__JKI_lib_State_Machine.vi"("State(s) in (\"\")"=w1830) -> ("States Out"=w1829:string)  [unwired: 14 in]
      }
      frame "Run: Increment" {
        # "Increase Run# by 1"
        n787 = Unbundle By Name(w1833) -> ("IDs.RunID"=w1835:i8)
        n788 = Increment(x=w1835) -> (x+1=w1832:i8)
        n789 = Bundle By Name(cluster=w1833, "IDs.RunID"=w1832) -> (w1834:T20)
        n790 = call <vilib>:"Add State(s) to Queue__JKI_lib_State_Machine.vi"("State(s) in (\"\")"=w1838) -> ("States Out"=w1837:string)  [unwired: 14 in]
      }
      frame "Run: Decrement" {
        # "Increase Run# by 1"
        n791 = Unbundle By Name(w1841) -> ("IDs.RunID"=w1843:i8)
        n792 = Decrement(x=w1843) -> (x-1=w1840:i8)
        n793 = Bundle By Name(cluster=w1841, "IDs.RunID"=w1840) -> (w1842:T20)
        n794 = call <vilib>:"Add State(s) to Queue__JKI_lib_State_Machine.vi"("State(s) in (\"\")"=w1846) -> ("States Out"=w1845:string)  [unwired: 14 in]
      }
      frame "---------- SysConfig ----------" {
        # "Template Separator\n(You can make a copy of, or modify, this frame)"
        n795 = call <vilib>:"Add State(s) to Queue__JKI_lib_State_Machine.vi"("State(s) in (\"\")"=w1851) -> ("States Out"=w1850:string)  [unwired: 14 in]
      }
      frame "SysConfig: LoadAPDSerialNumber" {
        w1857 = T23 {"Ch1APDSerial#"="", "Ch2APDSerial#"="", "Ch3APDSerial#"=""}  # APD Serials cons
        # "Template Separator\n(You can make a copy of, or modify, this frame)"
        n796 = call <vilib>:"Application Directory.vi"() -> ("Application Directory"=w1864:path)
        n797 = Build Path(base path=w1864, name or relative path="ConfigFiles\\APDSerial.txt") -> (appended path=w1862:path)
        n798 = Read from Text File(file (use dialog)=w1862, error in=w1852) -> (text=w1859:string, error out=w1858:errorcluster)  [unwired: 2 in, 2 out]
        n799 = call <vilib>:"Unflatten From JSON String.vi"("Type and Defaults"=w1857, "error in"=w1858, "JSON String"=w1859) -> ("error out"=w1860:errorcluster, "Variant"=w1861:variant)  [unwired: 7 in]
        n800 = Variant To Data(error in=w1860, type=w1857, Variant=w1861) -> (data=w1856:T23, error out=w1853:errorcluster)
        n801 = Bundle By Name(cluster=w1854, "APDSerialNum"=w1856) -> (w1855:T20)
        n802 = call <vilib>:"Add State(s) to Queue__JKI_lib_State_Machine.vi"("State(s) in (\"\")"=w1867) -> ("States Out"=w1866:string)  [unwired: 14 in]
      }
      frame "SysConfig: Load Sys Config" {
        # "[Covers: REQ5]"
        # "Load System config"
        # "Load system configuration\n(Load both hardware and DAQ config)"
        n803 = call "LoadSysConfig.vi"("Error In"=w1870, "Enum"=enum16{"LastUse", "Default"}."LastUse") -> ("Error Out"=w1869:errorcluster, "SysConfigCluster"=w1872:T3)  [unwired: 8 in]
        "SysConfigCluster" <- w1872
        n804 = Bundle By Name(cluster=w1873, "SysConfigCluster"=w1872) -> (w1874:T20)
        n805 = call <vilib>:"Add State(s) to Queue__JKI_lib_State_Machine.vi"("State(s) in (\"\")"=w1876) -> ("States Out"=w1875:string)  [unwired: 14 in]
      }
      frame "SysConfig: Load Digitizer Setting" {
        w1877 = enum16{"Write", "Read"}."Write" ("Operation")
        # "Load DAQ config\nSave to FGV"
        # "Template Separator\n(You can make a copy of, or modify, this frame)"
        n806 = call <userlib>:"Current VIs Parent Directory__ogtk.vi"() -> ("Parent Directory (+ Relative)"=w1891:path)  [unwired: 5 in]
        n807 = Build Path(base path=w1891, name or relative path="SubVI\\DigitizerConfiguration\\V6_Scope_last_use.config") -> (appended path=w1892:path)
        n808 = call "ReadDigitizerConfig(SubVI).vi"("error in (no error)"=w1889, "appended path"=w1892) -> ("error out"=w1885:errorcluster, "FLImDAQ"=w1883:T5)  [unwired: 8 in]
        n809 = call "FLImDAQ_FGV.vi"("error in (no error)"=w1885, "Operation (Read)"=w1877, "Write data"=w1883) -> ("error out"=w1887:errorcluster)  [unwired: 7 in, 1 out]
        n810 = Unbundle By Name(w1883) -> ("min record length"=→"data length":i32, "Digitizer 1"=w1879:refnum<k15>, "Digitizer 2"=w1886:refnum<k15>)
        n811 = Bundle By Name(cluster=w1881, "FLImDAQ"=w1883) -> (w1882:T20)
        n812 = call "Digitizer1_FGV.vi"("error in (no error)"=w1887, "Operation (Read)"=w1877, "Write data"=w1879) -> ("error out"=w1888:errorcluster)  [unwired: 7 in, 1 out]
        n813 = call "Digitizer2_FGV.vi"("error in (no error)"=w1888, "Operation (Read)"=w1877, "Write data"=w1886) -> ("error out"=w1884:errorcluster)  [unwired: 7 in, 1 out]
        n814 = call <vilib>:"Add State(s) to Queue__JKI_lib_State_Machine.vi"("State(s) in (\"\")"=w1894) -> ("States Out"=w1893:string)  [unwired: 14 in]
      }
      frame "SysConfig: Load LJ Pinout" {
        # "Template Separator\n(You can make a copy of, or modify, this frame)"
        n815 = call <userlib>:"Current VIs Parent Directory__ogtk.vi"() -> ("Parent Directory (+ Relative)"=w1908:path)  [unwired: 5 in]
        n816 = Build Path(base path=w1908, name or relative path="SubVI\\LabJack\\LJ_pin_setting.config") -> (appended path=w1906:path)
        n817 = call "ReadLabjackConfig(SubVI).vi"("error in (no error)"=w1904, "appended path"=w1906) -> ("error out"=w1905:errorcluster, "Utility"=w1902:T4)  [unwired: 8 in]
        n818 = Unbundle By Name(w1902) -> ("Ch1 Bias"=w1901:string, "Ch2 Bias"=w1900:string, "Ch3 Bias"=w1899:string, "Red LED"=w1896:string, "Green LED"=w1895:string)
        n819 = global write "GlobalVariables.vi" "LED Green pin"(w1895) -> ()
        n820 = global write "GlobalVariables.vi" "LED Red pin"(w1896) -> ()
        n821 = global write "GlobalVariables.vi" "Ch1 LJ pin"(w1901) -> ()
        n822 = global write "GlobalVariables.vi" "Ch2 LJ pin"(w1900) -> ()
        n823 = global write "GlobalVariables.vi" "Ch3 LJ pin"(w1899) -> ()
        n824 = Bundle By Name(cluster=w1897, "LJ Pinout"=w1902) -> (w1903:T20)
        n825 = call <vilib>:"Add State(s) to Queue__JKI_lib_State_Machine.vi"("State(s) in (\"\")"=w1910) -> ("States Out"=w1909:string)  [unwired: 14 in]
      }
      frame "SysConfig: Load 355 PWM" {
        # "Template Separator\n(You can make a copy of, or modify, this frame)"
        n826 = call <userlib>:"Current VIs Parent Directory__ogtk.vi"() -> ("Parent Directory (+ Relative)"=w1928:path)  [unwired: 5 in]
        n827 = Build Path(base path=w1928, name or relative path="SubVI\\LabJack\\PWM_setting_355.config") -> (appended path=w1926:path)
        n828 = call "ReadPWMConfig(SubVI).vi"("error in (no error)"=w1923, "appended path"=w1926) -> ("error out"=w1924:errorcluster, "PWM Setting"=w1922:T36)  [unwired: 8 in]
        n829 = Unbundle By Name(w1922) -> ("DIO_EF_CLOCK1_DIVISOR"=w1919:i16, "DIO_EF_CLOCK1_ROLL_VALUE"=w1918:i32)
        n830 = Multiply(x=w1919, y=w1918) -> (x*y=w1920:i32)
        n831 = Bundle By Name(cluster=w1925, "355 PWM setting"=w1922) -> (w1912:T20)
        n832 = Divide(x=80000000.0, y=w1920) -> (x/y=w1917:dbl)
        "Laser Rep Rate" <- w1917
        n833 = Number To Decimal String(number=w1917) -> (decimal integer string=w1916:string)  [unwired: 1 in]
        n834 = Concatenate Strings("355nm " ("string"), w1916, "Hz" ("string")) -> (w1914:string)
        n835 = property on="355nm Laser toggle" class="Bool (strict)"("Caption.Text"=w1914) -> ()  [unwired: 2 in, 2 out]
        n836 = call <vilib>:"Add State(s) to Queue__JKI_lib_State_Machine.vi"("State(s) in (\"\")"=w1930) -> ("States Out"=w1929:string)  [unwired: 14 in]
      }
      frame "SysConfig: Load AB PWM" {
        # "Template Separator\n(You can make a copy of, or modify, this frame)"
        n837 = call <userlib>:"Current VIs Parent Directory__ogtk.vi"() -> ("Parent Directory (+ Relative)"=w1939:path)  [unwired: 5 in]
        n838 = Build Path(base path=w1939, name or relative path="SubVI\\LabJack\\PWM_setting_AB.config") -> (appended path=w1937:path)
        n839 = call "ReadPWMConfig(SubVI).vi"("error in (no error)"=w1934, "appended path"=w1937) -> ("error out"=w1935:errorcluster, "PWM Setting"=w1933:T36)  [unwired: 8 in]
        n840 = Bundle By Name(cluster=w1931, "AB PWM setting"=w1933) -> (w1936:T20)
        n841 = call <vilib>:"Add State(s) to Queue__JKI_lib_State_Machine.vi"("State(s) in (\"\")"=w1941) -> ("States Out"=w1940:string)  [unwired: 14 in]
      }
      frame "SysConfig: Load AB setting" {
        # "Template Separator\n(You can make a copy of, or modify, this frame)"
        n842 = call "readAimingBeamSetting.vi"("error in (no error)"=w1959) -> ("error out"=w1954:errorcluster, "Aiming Beam Setting"=w1946:T37)  [unwired: 9 in]
        n843 = Unbundle By Name(w1946) -> ("Default Current"=w1945:dbl)
        n844 = Unbundle By Name(w1946) -> ("Frequency(Hz)"=w1942:u32)
        n845 = Equal To 0?(x=w1942) -> (x = 0?=w1952:bool)
        n846 = Select(t="", s=w1952, f="SysConfig: Load AB PWM" ("State(s) in Front (\"\")")) -> (s? t:f=w1955:string)
        n847 = Number To Decimal String(number=w1942) -> (decimal integer string=w1951:string)  [unwired: 1 in]
        n848 = Number To Decimal String(number=w1945, width (-)=i16 2) -> (decimal integer string=w1944:string)
        n849 = Concatenate Strings("445nm " ("string"), w1951, "Hz " ("string"), w1944, "mA" ("string")) -> (w1950:string)
        n850 = property on="Aiming beam toggle" class="Bool (strict)"("Caption.Text"=w1950) -> ()  [unwired: 2 in, 2 out]
        n851 = case shown="False" w1952 {
          tunnel: w1954 -> [w1965 w1968]
          tunnel: [w1964 w1968] -> w1953
          frame False {
            n852 = call "LJ_calculate_PWM_parameters.vi"("Error In"=w1965, "Show Confirmation"=FALSE, "Laser"=enum16{"355nm", "AimingBeam"}."AimingBeam") -> ("Error Out"=w1964:errorcluster)  [unwired: 7 in, 1 out]
          }
          frame True {
          }
        }
        n853 = Bundle By Name(cluster=w1960, "AB Cluster"=w1946) -> (w1961:T20)
        n854 = call <vilib>:"Add State(s) to Queue__JKI_lib_State_Machine.vi"("State(s) in Front (\"\")"=w1955, "State(s) in (\"\")"=w1963) -> ("States Out"=w1962:string)  [unwired: 13 in]
      }
      frame "SysConfig: LoadABVideoSetting" {
        # "Load AB video setting form ini file\n()"
        n855 = call "readVideoConfig.vi"("error in (no error)"=w1972) -> ("error out"=w1973:errorcluster, "Aiming Beam Config"=w1971:T19)  [unwired: 8 in, 1 out]
        n856 = Bundle By Name(cluster=w1969, "VideoConfig"=w1971) -> (w1970:T20)
        n857 = call <vilib>:"Add State(s) to Queue__JKI_lib_State_Machine.vi"("State(s) in (\"\")"=w1976) -> ("States Out"=w1975:string)  [unwired: 14 in]
      }
      frame "SysConfig: LoadCursorLocation" {
        # "Load cursor location from ini file\n(load cursor from system setting ini file)"
        n858 = call "readCursorConfigMain.vi"("error in (no error)"=w1982) -> ("error out"=w1983:errorcluster, "Cursor Locations"=w1981:T38)  [unwired: 9 in]
        n859 = Unbundle By Name(w1981) -> ("DC1"=w1980:i32, "DC2"=w1979:i32, "BG1"=w1978:i32, "BG2"=w1977:i32)
        n860 = global write "GlobalVariables.vi" "DC Idx1"(w1980) -> ()
        n861 = global write "GlobalVariables.vi" "DC Idx2"(w1979) -> ()
        n862 = global write "GlobalVariables.vi" "BG Idx1"(w1978) -> ()
        n863 = global write "GlobalVariables.vi" "BG Idx2"(w1977) -> ()
        n864 = call <vilib>:"Add State(s) to Queue__JKI_lib_State_Machine.vi"("State(s) in (\"\")"=w1987) -> ("States Out"=w1986:string)  [unwired: 14 in]
      }
      frame "---------- SystemStatus ----------" {
        # "Template Separator\n(You can make a copy of, or modify, this frame)"
        n865 = call <vilib>:"Add State(s) to Queue__JKI_lib_State_Machine.vi"("State(s) in (\"\")"=w1992) -> ("States Out"=w1991:string)  [unwired: 14 in]
      }
      frame "SystemStatus: SlowSysStatusMacro" {
        # "store system check time"
        # "Template Separator\n(You can make a copy of, or modify, this frame)"
        n866 = Tick Count (ms)() -> (millisecond timer value=w1995:u32)
        n867 = Bundle By Name(cluster=w1993, "SlowTimer"=w1995) -> (w1994:T20)
        n868 = call <vilib>:"Add State(s) to Queue__JKI_lib_State_Machine.vi"("State(s) in Front (\"\")"="Digitizer: checkTemp\nTCP: CheckConnection" ("State(s) in Front (\"\")"), "State(s) in (\"\")"=w2000) -> ("States Out"=w1999:string)  [unwired: 13 in]
      }
      frame "SystemStatus: FastSysStatusMacro" {
        # "store system check time"
        # "Template Separator\n(You can make a copy of, or modify, this frame)"
        n869 = Tick Count (ms)() -> (millisecond timer value=w2003:u32)
        n870 = Bundle By Name(cluster=w2001, "FastTimer"=w2003) -> (w2002:T20)
        n871 = call <vilib>:"Add State(s) to Queue__JKI_lib_State_Machine.vi"("State(s) in Front (\"\")"="355 Laser: CheckPWMStatus\nAimingBeam: GetPWMStatus\n/*355 Laser: CheckControllerStatus" ("State(s) in Front (\"\")"), "State(s) in (\"\")"=w2008) -> ("States Out"=w2007:string)  [unwired: 13 in]
      }
      frame "---------- UI ----------" {
        # "Do not put any code in this frame.\n(It is a separator no-op. You can make a copy of this frame to create a new UI frame)"
        n872 = call <vilib>:"Add State(s) to Queue__JKI_lib_State_Machine.vi"("State(s) in (\"\")"=w2013) -> ("States Out"=w2012:string)  [unwired: 14 in]
      }
      frame "UI: Initialize" {
        w2014 = T39 {"Minimum"=0.0, "Maximum"=4.6, "Increment"=0.1} ("Data Entry Limits")
        w2016 = T8."Disabled and Grayed Out" ("Disabled")
        # "Disable all button on startup"
        # "Initialize the User Interface, here.\n(this is called automatically, by the Macro: Init)"
        n873 = property on="V 1" class="DigNum (strict)"("DisabledEnum"=w2016) -> ()  [unwired: 2 in, 2 out]
        n874 = property on="V 2" class="DigNum (strict)"("DisabledEnum"=w2016) -> ()  [unwired: 2 in, 2 out]
        n875 = property on="StopButton" class="Bool (strict)"("DisabledEnum"=w2016) -> ()  [unwired: 2 in, 2 out]
        n876 = property on="Sys Reconfig" class="Bool"("DisabledEnum"=w2016) -> ()  [unwired: 2 in, 2 out]
        n877 = property on="StartButton" class="Bool (strict)"("DisabledEnum"=w2016) -> ()  [unwired: 2 in, 2 out]
        n878 = property on="355nm Laser toggle" class="Bool (strict)"("DisabledEnum"=w2016) -> ()  [unwired: 2 in, 2 out]
        n879 = property on="Aiming beam toggle" class="Bool (strict)"("DisabledEnum"=w2016) -> ()  [unwired: 2 in, 2 out]
        n880 = property on="Background" class="Bool (strict)"("DisabledEnum"=w2016) -> ()  [unwired: 2 in, 2 out]
        n881 = property on="Cali&iRF alignment" class="Bool (strict)"("DisabledEnum"=w2016) -> ()  [unwired: 2 in, 2 out]
        n882 = property on="V 3" class="DigNum (strict)"("DisabledEnum"=w2016) -> ()  [unwired: 2 in, 2 out]
        n883 = property on="V 1" class="DigNum (strict)"("Data Range"=w2014) -> ()  [unwired: 2 in, 2 out]
        n884 = property on="V 2" class="DigNum (strict)"("Data Range"=w2014) -> ()  [unwired: 2 in, 2 out]
        n885 = property on="V 3" class="DigNum (strict)"("Data Range"=w2014) -> ()  [unwired: 2 in, 2 out]
        n886 = call <vilib>:"Add State(s) to Queue__JKI_lib_State_Machine.vi"("State(s) in Front (\"\")"="UI: CaliAndiRFNotReady" ("State(s) in Front (\"\")"), "State(s) in (\"\")"=w2021) -> ("States Out"=w2020:string)  [unwired: 13 in]
      }
      frame "UI: BGLoaded" {
        # "[Covers: REQ24]"
        # "Do not put any code in this frame.\n(It is a separator no-op. You can make a copy of this frame to create a new UI frame)"
        n887 = property on="Background" class="Bool (strict)"("BoolText.Text"="Loaded!" ("Boolean Text.Text"), "Colors [4]"=cluster{u32, u32}[] [{15764023, 15764023}, {16711680, 16711680}]) -> ()  [unwired: 2 in, 2 out]
        n888 = call <vilib>:"Add State(s) to Queue__JKI_lib_State_Machine.vi"("State(s) in (\"\")"=w2028) -> ("States Out"=w2027:string)  [unwired: 14 in]
      }
      frame "UI: CaliAndiRFLoaded" {
        # "[Covers: REQ24]"
        # "Do not put any code in this frame.\n(It is a separator no-op. You can make a copy of this frame to create a new UI frame)"
        n889 = property on="Cali&iRF alignment" class="Bool (strict)"("BoolText.Text"="Loaded!" ("Boolean Text.Text"), "Colors [4]"=cluster{u32, u32}[] [{15764023, 15764023}, {16711680, 16711680}]) -> ()  [unwired: 2 in, 2 out]
        n890 = call <vilib>:"Add State(s) to Queue__JKI_lib_State_Machine.vi"("State(s) in (\"\")"=w2035) -> ("States Out"=w2034:string)  [unwired: 14 in]
      }
      frame "UI: WFAutoScale" {
        # "Set graph auto scale.\n(UI: WFAutoScale >> T/F)"
        n891 = Equal?(x=w2036, y="F") -> (x = y?=w2037:bool)
        n892 = Equal?(x=w2036, y="T") -> (x = y?=w2039:bool)
        n893 = case shown="True" w2039 {
          frame False {
          }
          frame True {
            w2055 = u8 2 ("Y Scale.Scale Fit")
            n894 = property on="Channel 1" class="WFGraph (strict)"("YScale.ScaleFit"=w2055) -> ()  [unwired: 2 in, 2 out]
            n895 = property on="Channel 2" class="WFGraph (strict)"("YScale.ScaleFit"=w2055) -> ()  [unwired: 2 in, 2 out]
            n896 = property on="Channel 3" class="WFGraph (strict)"("YScale.ScaleFit"=w2055) -> ()  [unwired: 2 in, 2 out]
          }
        }
        n897 = case shown="True" w2037 {
          frame False {
          }
          frame True {
            w2052 = 0.0 ("Y Scale.Range:Maximum")
            w2053 = 2.0 ("Y Scale.Range:Maximum")
            w2054 = u8 0 ("Y Scale.Scale Fit")
            n898 = property on="Channel 1" class="WFGraph (strict)"("YScale.ScaleFit"=w2054) -> (error out=w2051:errorcluster)  [unwired: 2 in, 1 out]
            n899 = property on="Channel 2" class="WFGraph (strict)"("YScale.ScaleFit"=w2054) -> (error out=w2050:errorcluster)  [unwired: 2 in, 1 out]
            n900 = property on="Channel 3" class="WFGraph (strict)"("YScale.ScaleFit"=w2054) -> (error out=w2049:errorcluster)  [unwired: 2 in, 1 out]
            n901 = property on="Channel 1" class="WFGraph (strict)"(error in=w2051, "YScale.Maximum"=w2053) -> (error out=w2048:errorcluster)  [unwired: 1 in, 1 out]
            n902 = property on="Channel 2" class="WFGraph (strict)"(error in=w2050, "YScale.Maximum"=w2053) -> (error out=w2047:errorcluster)  [unwired: 1 in, 1 out]
            n903 = property on="Channel 3" class="WFGraph (strict)"(error in=w2049, "YScale.Maximum"=w2053) -> (error out=w2046:errorcluster)  [unwired: 1 in, 1 out]
            n904 = property on="Channel 1" class="WFGraph (strict)"(error in=w2048, "YScale.Minimum"=w2052) -> ()  [unwired: 1 in, 2 out]
            n905 = property on="Channel 2" class="WFGraph (strict)"(error in=w2047, "YScale.Minimum"=w2052) -> ()  [unwired: 1 in, 2 out]
            n906 = property on="Channel 3" class="WFGraph (strict)"(error in=w2046, "YScale.Minimum"=w2052) -> ()  [unwired: 1 in, 2 out]
          }
        }
        n907 = call <vilib>:"Add State(s) to Queue__JKI_lib_State_Machine.vi"("State(s) in (\"\")"=w2045) -> ("States Out"=w2044:string)  [unwired: 14 in]
      }
      frame "UI: showDisclaimer" {
        # "Show disclamer window.\n(It is a separator no-op. You can make a copy of this frame to create a new UI frame)"
        n908 = call <vilib>:"Application Directory.vi"() -> ("Application Directory"=w2068:path)
        n909 = Build Path(base path=w2068, name or relative path="Disclamer.png") -> (appended path=w2066:path)
        n910 = property on="Disclamer" class="Pict"() -> ("Draw Area Size"=w2064:T40)  [unwired: 2 in, 2 out]
        n911 = disable-structure "Diagram Disable Structure" shown="Disabled" {
          frame Disabled {
            n912 = flat-sequence {
              frame #0 {
                n913 = call "disclaimer.vi"() -> ()  [unwired: 12 in]
              }
              frame #1 {
                n914 = Wait (ms)(milliseconds to wait=u32 250) -> ()  [unwired: 1 out]
              }
              frame #2 {
                n915 = call "SoftwareNote.vi"() -> ()  [unwired: 12 in]
              }
            }
          }
          frame Enabled {
          }
        }
        n916 = call <vilib>:"Read PNG File.vi"("path to PNG file"=w2066) -> ("image data"=w2063:T41)  [unwired: 8 in, 2 out]
        n917 = Unbundle By Name(w2063) -> ("Rectangle.right"=w2061:i16, "Rectangle.bottom"=w2059:i16)
        n918 = Unbundle By Name(w2064) -> ("Width"=w2062:u32, "Height"=w2060:u32)
        n919 = call <vilib>:"Draw Flattened Pixmap.vi"("image data"=w2063) -> ("new picture"=→"Disclamer":picture)  [unwired: 8 in]
        n920 = Divide(x=w2062, y=w2061) -> (x/y=w2058:dbl)
        n921 = Divide(x=w2060, y=w2059) -> (x/y=w2057:dbl)
        n922 = Max & Min(x=w2058, y=w2057) -> (min(x,y)=w2056:dbl)  [unwired: 1 out]
        n923 = property on="Disclamer" class="Pict"("ZoomFactor"=w2056) -> ()  [unwired: 2 in, 2 out]
        n924 = call <vilib>:"Add State(s) to Queue__JKI_lib_State_Machine.vi"("State(s) in (\"\")"=w2073) -> ("States Out"=w2072:string)  [unwired: 14 in]
      }
      frame "UI: CaliAndiRFNotReady" {
        # "Do not put any code in this frame.\n(It is a separator no-op. You can make a copy of this frame to create a new UI frame)"
        n925 = property on="Cali&iRF alignment" class="Bool (strict)"("BoolText.Text"="No Info" ("Boolean Text.Text"), "Colors [4]"=cluster{u32, u32}[] [{13816530, 13816530}, {16711680, 16711680}]) -> ()  [unwired: 2 in, 2 out]
        n926 = call <vilib>:"Add State(s) to Queue__JKI_lib_State_Machine.vi"("State(s) in (\"\")"=w2081) -> ("States Out"=w2080:string)  [unwired: 14 in]
      }
      frame "UI: BGnotReady" {
        # "Do not put any code in this frame.\n(It is a separator no-op. You can make a copy of this frame to create a new UI frame)"
        n927 = property on="Background" class="Bool (strict)"("BoolText.Text"="No Info" ("Boolean Text.Text"), "Colors [4]"=cluster{u32, u32}[] [{13816530, 13816530}, {16711680, 16711680}]) -> ()  [unwired: 2 in, 2 out]
        n928 = call <vilib>:"Add State(s) to Queue__JKI_lib_State_Machine.vi"("State(s) in (\"\")"=w2088) -> ("States Out"=w2087:string)  [unwired: 14 in]
      }
      frame "UI: Reset" {
        w2090 = cluster{u32, u32}[] [{13816530, 13816530}, {13816530, 13816530}] ("Colors [4]")
        # "Do not put any code in this frame.\n(It is a separator no-op. You can make a copy of this frame to create a new UI frame)"
        n929 = property on="Cali&iRF alignment" class="Bool (strict)"("BoolText.Text"="No Info" ("Boolean Text.Text"), "Colors [4]"=w2090) -> ()  [unwired: 2 in, 2 out]
        n930 = property on="Background" class="Bool (strict)"("BoolText.Text"="No Info" ("Boolean Text.Text"), "Colors [4]"=w2090) -> ()  [unwired: 2 in, 2 out]
        n931 = call <vilib>:"Add State(s) to Queue__JKI_lib_State_Machine.vi"("State(s) in (\"\")"=w2096) -> ("States Out"=w2095:string)  [unwired: 14 in]
      }
      frame "UI: SetButtonText" {
        # "Set button text of 355nm laser and aiming beam."
        n932 = call <vilib>:"Add State(s) to Queue__JKI_lib_State_Machine.vi"("State(s) in (\"\")"=w2101) -> ("States Out"=w2100:string)  [unwired: 14 in]
      }
      frame "UI: DuringAquisition" {
        w2102 = T8."Disabled and Grayed Out" ("Disabled")
        # "Do not put any code in this frame.\n(It is a separator no-op. You can make a copy of this frame to create a new UI frame)"
        n933 = property on="StopButton" class="Bool (strict)"("DisabledEnum"=T8."Enabled" ("Disabled")) -> ()  [unwired: 2 in, 2 out]
        n934 = property on="StartButton" class="Bool (strict)"("DisabledEnum"=w2102) -> ()  [unwired: 2 in, 2 out]
        n935 = property on="Sys Reconfig" class="Bool"("DisabledEnum"=w2102) -> ()  [unwired: 2 in, 2 out]
        n936 = property on="355nm Laser toggle" class="Bool (strict)"("DisabledEnum"=w2102) -> ()  [unwired: 2 in, 2 out]
        n937 = property on="Aiming beam toggle" class="Bool (strict)"("DisabledEnum"=w2102) -> ()  [unwired: 2 in, 2 out]
        n938 = property on="Background" class="Bool (strict)"("DisabledEnum"=w2102) -> ()  [unwired: 2 in, 2 out]
        n939 = property on="Radio Buttons" class="RadioBtnsControl (strict)"("DisabledEnum"=w2102) -> ()  [unwired: 2 in, 2 out]
        n940 = property on="Cali&iRF alignment" class="Bool (strict)"("DisabledEnum"=w2102) -> ()  [unwired: 2 in, 2 out]
        n941 = property on="Video Source" class="RadioBtnsControl (strict)"("DisabledEnum"=w2102) -> ()  [unwired: 2 in, 2 out]
        n942 = property on="Quit" class="Bool"("DisabledEnum"=w2102) -> ()  [unwired: 2 in, 2 out]
        n943 = property on="Skip Data Save?" class="Bool (strict)"("DisabledEnum"=w2102) -> ()  [unwired: 2 in, 2 out]
        n944 = property on="Video Display" class="Bool (strict)"("DisabledEnum"=w2102) -> ()  [unwired: 2 in, 2 out]
        n945 = call <vilib>:"Add State(s) to Queue__JKI_lib_State_Machine.vi"("State(s) in (\"\")"=w2108) -> ("States Out"=w2107:string)  [unwired: 14 in]
      }
      frame "UI: duringIRFAlign" {
        w2109 = T8."Disabled and Grayed Out" ("Disabled")
        # "Set UI to during iRF alignment\n(It is a separator no-op. You can make a copy of this frame to create a new UI frame)"
        n946 = property on="StartButton" class="Bool (strict)"("DisabledEnum"=w2109) -> ()  [unwired: 2 in, 2 out]
        n947 = property on="Sys Reconfig" class="Bool"("DisabledEnum"=w2109) -> ()  [unwired: 2 in, 2 out]
        n948 = property on="355nm Laser toggle" class="Bool (strict)"("DisabledEnum"=w2109) -> ()  [unwired: 2 in, 2 out]
        n949 = property on="Aiming beam toggle" class="Bool (strict)"("DisabledEnum"=w2109) -> ()  [unwired: 2 in, 2 out]
        n950 = property on="Background" class="Bool (strict)"("DisabledEnum"=w2109) -> ()  [unwired: 2 in, 2 out]
        n951 = property on="StopButton" class="Bool (strict)"("DisabledEnum"=w2109) -> ()  [unwired: 2 in, 2 out]
        n952 = call <vilib>:"Add State(s) to Queue__JKI_lib_State_Machine.vi"("State(s) in (\"\")"=w2114) -> ("States Out"=w2113:string)  [unwired: 14 in]
      }
      frame "UI: duringBGAcquire" {
        w2115 = T8."Disabled and Grayed Out" ("Disabled")
        # "Do not put any code in this frame.\n(It is a separator no-op. You can make a copy of this frame to create a new UI frame)"
        n953 = property on="StartButton" class="Bool (strict)"("DisabledEnum"=w2115) -> ()  [unwired: 2 in, 2 out]
        n954 = property on="StopButton" class="Bool (strict)"("DisabledEnum"=w2115) -> ()  [unwired: 2 in, 2 out]
        n955 = property on="Sys Reconfig" class="Bool"("DisabledEnum"=w2115) -> ()  [unwired: 2 in, 2 out]
        n956 = property on="355nm Laser toggle" class="Bool (strict)"("DisabledEnum"=w2115) -> ()  [unwired: 2 in, 2 out]
        n957 = property on="Aiming beam toggle" class="Bool (strict)"("DisabledEnum"=w2115) -> ()  [unwired: 2 in, 2 out]
        n958 = property on="Cali&iRF alignment" class="Bool (strict)"("DisabledEnum"=w2115) -> ()  [unwired: 2 in, 2 out]
        n959 = call <vilib>:"Add State(s) to Queue__JKI_lib_State_Machine.vi"("State(s) in (\"\")"=w2120) -> ("States Out"=w2119:string)  [unwired: 14 in]
      }
      frame "UI: ReadyForAquisition" {
        w2123 = T8."Enabled" ("Disabled")
        # "Do not put any code in this frame.\n(It is a separator no-op. You can make a copy of this frame to create a new UI frame)"
        n960 = Unbundle By Name(w2122) -> ("System Status.TCP/IP"=w2121:bool)
        n961 = property on="StopButton" class="Bool (strict)"("DisabledEnum"=T8."Disabled and Grayed Out" ("Disabled")) -> ()  [unwired: 2 in, 2 out]
        n962 = property on="StartButton" class="Bool (strict)"("DisabledEnum"=w2123) -> ()  [unwired: 2 in, 2 out]
        n963 = property on="Sys Reconfig" class="Bool"("DisabledEnum"=w2123) -> ()  [unwired: 2 in, 2 out]
        n964 = property on="355nm Laser toggle" class="Bool (strict)"("DisabledEnum"=w2123) -> ()  [unwired: 2 in, 2 out]
        n965 = property on="Aiming beam toggle" class="Bool (strict)"("DisabledEnum"=w2123) -> ()  [unwired: 2 in, 2 out]
        n966 = property on="Cali&iRF alignment" class="Bool (strict)"("DisabledEnum"=w2123) -> ()  [unwired: 2 in, 2 out]
        n967 = property on="Video Source" class="RadioBtnsControl (strict)"("DisabledEnum"=w2123) -> ()  [unwired: 2 in, 2 out]
        n968 = property on="Background" class="Bool (strict)"("DisabledEnum"=w2123) -> ()  [unwired: 2 in, 2 out]
        n969 = property on="Quit" class="Bool"("DisabledEnum"=w2123) -> ()  [unwired: 2 in, 2 out]
        n970 = property on="Radio Buttons" class="RadioBtnsControl (strict)"("DisabledEnum"=w2123) -> ()  [unwired: 2 in, 2 out]
        n971 = property on="Skip Data Save?" class="Bool (strict)"("DisabledEnum"=w2123) -> ()  [unwired: 2 in, 2 out]
        n972 = case shown="True" w2121 {
          tunnel: w2123 -> [_ w2129]
          frame False {
          }
          frame True {
            n973 = property on="Video Display" class="Bool (strict)"("DisabledEnum"=w2129) -> ()  [unwired: 2 in, 2 out]
          }
        }
        n974 = call <vilib>:"Add State(s) to Queue__JKI_lib_State_Machine.vi"("State(s) in (\"\")"=w2128) -> ("States Out"=w2127:string)  [unwired: 14 in]
      }
      frame "UI: Update" {
        # "Do not put any code in this frame.\n(It is a separator no-op. You can make a copy of this frame to create a new UI frame)"
        n975 = Unbundle By Name(w2139) -> ("System Status"=→"System Hardware Connection Status":T1, "IDs.RunID"=→"Run #":i8, "CaseID"=→"Case #":string, "FLImDAQ"=→"FLImDAQ":T27, "SysRunning?"=→"Aquisition Status:":bool, "LJ Pinout"=→"LJ Pinout":T4, "IDs.BG ID"=→"BG #":i8, "IDs.Cali ID"=→"Calibration #":i8)
        n976 = call <vilib>:"Add State(s) to Queue__JKI_lib_State_Machine.vi"("State(s) in (\"\")"=w2142) -> ("States Out"=w2141:string)  [unwired: 14 in]
      }
      frame "UI: Cursor Set" {
        # "Argument"
        # "Set and Unset Cursor Busy.\n(Usage: \"UI: Cursor Set >> Busy|Idle\")"
        n977 = case shown="\"Idle\", Default" w2144 {
          tunnel: w2146 -> [w2151 w2153]
          tunnel: [w2150 w2152] -> w2145
          frame "Idle", Default {
            n978 = call <vilib>:"Unset Busy.vi"("error in (no error)"=w2151) -> ("error out"=w2150:errorcluster)  [unwired: 10 in]
          }
          frame "Busy" {
            n979 = call <vilib>:"Set Busy.vi"("error in (no error)"=w2153) -> ("error out"=w2152:errorcluster)  [unwired: 9 in, 1 out]
          }
        }
        n980 = call <vilib>:"Add State(s) to Queue__JKI_lib_State_Machine.vi"("State(s) in (\"\")"=w2149) -> ("States Out"=w2148:string)  [unwired: 14 in]
      }
      frame "UI: Front Panel State" {
        # "Argument"
        # "Set Front Panel Open or Closed\n(Usage: \"UI: Front Panel State >> Open|Close\")"
        n981 = Unbundle By Name(w2157) -> ("Core.Current VI Reference"=w2156:refnum<vi>)
        n982 = case shown="\"Open\", \"Standard\", Default" w2155 {
          tunnel: w2159 -> [w2167 w2182 w2193 w2206 w2219]
          tunnel: [w2169 w2183 w2195 w2208 w2221] -> w2158
          tunnel: w2156 -> [w2168 w2180 w2194 w2207 w2220]
          frame "Open", "Standard", Default {
            w2162 = T14."Standard" ("State")
            n983 = property on="Property Node" class="VI"(reference=w2168, error in=w2167) -> (reference out=w2165:refnum<vi>, error out=w2166:errorcluster, "FP.State"=w2164:T14)
            n984 = Not Equal?(x=w2164, y=w2162) -> (x != y?=w2163:bool)
            n985 = case shown="True" w2163 {
              tunnel: [w2173 w2175] -> w2169
              tunnel: w2166 -> [w2172 w2175]
              tunnel: w2165 -> [w2171 _]
              tunnel: w2162 -> [w2170 _]
              frame True {
                n986 = invoke on="Invoke Node" class="VI" method="FP.Open"(reference=w2171, error in=w2172, "Activate"=TRUE, "State"=w2170) -> (error out=w2173:errorcluster)  [unwired: 1 in, 4 out]
              }
              frame False {
              }
            }
          }
          frame "Close", "Closed" {
            n987 = property on="Property Node" class="VI"(reference=w2180, error in=w2182) -> (reference out=w2179:refnum<vi>, error out=w2181:errorcluster, "FP.State"=w2177:T14)
            n988 = Not Equal?(x=w2177, y=T14."Closed" ("Front Panel Window:State")) -> (x != y?=w2176:bool)
            n989 = case shown="True" w2176 {
              tunnel: [w2184 w2187] -> w2183
              tunnel: w2181 -> [w2184 w2186]
              tunnel: w2179 -> [_ w2185]
              frame False {
              }
              frame True {
                n990 = invoke on="Invoke Node" class="VI" method="FP.Close"(reference=w2185, error in=w2186) -> (error out=w2187:errorcluster)  [unwired: 1 in, 2 out]
              }
            }
          }
          frame "Hidden", "Hide" {
            w2188 = T14."Hidden" ("State")
            n991 = property on="Property Node" class="VI"(reference=w2194, error in=w2193) -> (reference out=w2191:refnum<vi>, error out=w2192:errorcluster, "FP.State"=w2190:T14)
            n992 = Not Equal?(x=w2190, y=w2188) -> (x != y?=w2189:bool)
            n993 = case shown="True" w2189 {
              tunnel: [w2199 w2200] -> w2195
              tunnel: w2192 -> [w2198 w2200]
              tunnel: w2191 -> [w2197 _]
              tunnel: w2188 -> [w2196 _]
              frame True {
                n994 = invoke on="Invoke Node" class="VI" method="FP.Open"(reference=w2197, error in=w2198, "State"=w2196) -> (error out=w2199:errorcluster)  [unwired: 2 in, 4 out]
              }
              frame False {
              }
            }
          }
          frame "Minimize", "Minimized" {
            w2201 = T14."Minimized" ("State")
            n995 = property on="Property Node" class="VI"(reference=w2207, error in=w2206) -> (reference out=w2204:refnum<vi>, error out=w2205:errorcluster, "FP.State"=w2203:T14)
            n996 = Not Equal?(x=w2203, y=w2201) -> (x != y?=w2202:bool)
            n997 = case shown="True" w2202 {
              tunnel: [w2212 w2213] -> w2208
              tunnel: w2205 -> [w2211 w2213]
              tunnel: w2204 -> [w2210 _]
              tunnel: w2201 -> [w2209 _]
              frame True {
                n998 = invoke on="Invoke Node" class="VI" method="FP.Open"(reference=w2210, error in=w2211, "State"=w2209) -> (error out=w2212:errorcluster)  [unwired: 2 in, 4 out]
              }
              frame False {
              }
            }
          }
          frame "Maximize", "Maximized" {
            w2214 = T14."Maximized" ("State")
            n999 = property on="Property Node" class="VI"(reference=w2220, error in=w2219) -> (reference out=w2217:refnum<vi>, error out=w2218:errorcluster, "FP.State"=w2216:T14)
            n1000 = Not Equal?(x=w2216, y=w2214) -> (x != y?=w2215:bool)
            n1001 = case shown="True" w2215 {
              tunnel: [w2225 w2226] -> w2221
              tunnel: w2218 -> [w2224 w2226]
              tunnel: w2217 -> [w2223 _]
              tunnel: w2214 -> [w2222 _]
              frame True {
                n1002 = invoke on="Invoke Node" class="VI" method="FP.Open"(reference=w2223, error in=w2224, "State"=w2222) -> (error out=w2225:errorcluster)  [unwired: 2 in, 4 out]
              }
              frame False {
              }
            }
          }
        }
        n1003 = call <vilib>:"Add State(s) to Queue__JKI_lib_State_Machine.vi"("State(s) in (\"\")"=w2161) -> ("States Out"=w2160:string)  [unwired: 14 in]
      }
      frame "---------- 355 Laser ----------" {
        # "Template Separator\n(You can make a copy of, or modify, this frame)"
        n1004 = call <vilib>:"Add State(s) to Queue__JKI_lib_State_Machine.vi"("State(s) in (\"\")"=w2231) -> ("States Out"=w2230:string)  [unwired: 14 in]
      }
      frame "355 Laser: Check Dewelling" {
        # "if time laser start time is less than 7.5s before, wait 250ms then check again."
        # "Template Separator\n(You can make a copy of, or modify, this frame)"
        n1005 = Unbundle By Name(w2239) -> ("Laser start tic"=w2236:u32)
        n1006 = Tick Count (ms)() -> (millisecond timer value=w2237:u32)
        n1007 = Subtract(x=w2237, y=w2236) -> (x-y=w2235:u32)
        n1008 = Greater?(x=w2235, y=u32 5000) -> (0:w2233:bool)
        n1009 = case shown="False" w2233 {
          tunnel: ["355 Laser: Check Dewelling" ""] -> w2232
          frame False {
            n1010 = Wait (ms)(milliseconds to wait=u32 250) -> ()  [unwired: 1 out]
          }
          frame True {
          }
        }
        n1011 = call <vilib>:"Add State(s) to Queue__JKI_lib_State_Machine.vi"("State(s) in Front (\"\")"=w2232, "State(s) in (\"\")"=w2242) -> ("States Out"=w2241:string)  [unwired: 13 in]
      }
      frame "355 Laser: Laser enable" {
        # "Laser enable/disable\n(Usage: \"LabJack: Laser enable/disable >> 1|0\")"
        n1012 = Unbundle By Name(w2249) -> ("LJ Pinout.Laser Start/Stop"=w2253:string, "System Status.355 Laser"=w2247:bool)
        n1013 = case shown="False" w2247 {
          tunnel: w2246 -> [w2268 w2269]
          tunnel: w2253 -> [w2262 _]
          tunnel: [w2257 w2269] -> w2251
          tunnel: [w2256 u32 0 ("millisecond timer value")] -> w2248
          frame False {
            n1014 = call "LabJack_FGV.vi"("Operation(Read)"=enum16{"Write", "Read"}."Read" ("Operation")) -> ("Read data"=w2264:i32)  [unwired: 9 in, 1 out]
            n1015 = call "LJM_eWriteName.vi"("Handle In"=w2264, "Name"=w2262, "Value"=1.0, "error in"=w2268) -> ("Handle Out"=w2263:i32, "error out"=w2261:errorcluster)  [unwired: 10 in]
            n1016 = call <userlib>:"Wait (ms)__ogtk.vi"("error in (no error)"=w2261, "milliseconds to wait"=u32 250) -> ("error out"=w2260:errorcluster)  [unwired: 8 in, 1 out]
            n1017 = call "LJM_eWriteName.vi"("Handle In"=w2263, "Name"=w2262, "Value"=0.0, "error in"=w2260) -> ("error out"=w2258:errorcluster)  [unwired: 10 in, 1 out]
            n1018 = call <userlib>:"Tick Count (ms)__ogtk.vi"("error in (no error)"=w2258) -> ("error out"=w2257:errorcluster, "millisecond timer value"=w2256:u32)  [unwired: 9 in]
          }
          frame True {
          }
        }
        n1019 = Bundle By Name(cluster=w2249, "Laser start tic"=w2248) -> (w2250:T20)
        n1020 = call <vilib>:"Add State(s) to Queue__JKI_lib_State_Machine.vi"("State(s) in (\"\")"=w2255) -> ("States Out"=w2254:string)  [unwired: 14 in]
      }
      frame "355 Laser: Laser disable" {
        # "Laser enable/disable\n(Usage: \"LabJack: Laser enable/disable >> 1|0\")"
        n1021 = Unbundle By Name(w2273) -> ("LJ Pinout.Laser Start/Stop"=w2277:string, "System Status.355 Laser"=w2271:bool)
        n1022 = case shown="True" w2271 {
          tunnel: w2278 -> [w2281 w2295]
          tunnel: w2277 -> [_ w2289]
          tunnel: [w2281 w2284] -> w2275
          tunnel: [u32 0 ("millisecond timer value") w2283] -> w2272
          frame False {
          }
          frame True {
            n1023 = call "LabJack_FGV.vi"("Operation(Read)"=enum16{"Write", "Read"}."Read" ("Operation")) -> ("Read data"=w2291:i32)  [unwired: 9 in, 1 out]
            n1024 = call "LJM_eWriteName.vi"("Handle In"=w2291, "Name"=w2289, "Value"=1.0, "error in"=w2295) -> ("Handle Out"=w2290:i32, "error out"=w2288:errorcluster)  [unwired: 10 in]
            n1025 = call <userlib>:"Wait (ms)__ogtk.vi"("error in (no error)"=w2288, "milliseconds to wait"=u32 250) -> ("error out"=w2287:errorcluster)  [unwired: 8 in, 1 out]
            n1026 = call "LJM_eWriteName.vi"("Handle In"=w2290, "Name"=w2289, "Value"=0.0, "error in"=w2287) -> ("error out"=w2285:errorcluster)  [unwired: 10 in, 1 out]
            n1027 = call <userlib>:"Tick Count (ms)__ogtk.vi"("error in (no error)"=w2285) -> ("error out"=w2284:errorcluster, "millisecond timer value"=w2283:u32)  [unwired: 9 in]
          }
        }
        n1028 = Bundle By Name(cluster=w2273, "Laser start tic"=w2272) -> (w2274:T20)
        n1029 = call <vilib>:"Add State(s) to Queue__JKI_lib_State_Machine.vi"("State(s) in (\"\")"=w2280) -> ("States Out"=w2279:string)  [unwired: 14 in]
      }
      frame "355 Laser: Dewelling" {
        # "Wait some time (ms)\n(355 Laser: Dewelling >> #)"
        n1030 = Fract/Exp String To Number(string=w2299, default (0 dbl)=0) -> (number=w2297:i32)  [unwired: 2 in, 1 out]
        n1031 = Wait (ms)(milliseconds to wait=w2297) -> ()  [unwired: 1 out]
        n1032 = call <vilib>:"Add State(s) to Queue__JKI_lib_State_Machine.vi"("State(s) in (\"\")"=w2303) -> ("States Out"=w2302:string)  [unwired: 14 in]
      }
      frame "355 Laser: Close" {
        # "Template Separator\n(You can make a copy of, or modify, this frame)"
        n1033 = call <vilib>:"Add State(s) to Queue__JKI_lib_State_Machine.vi"("State(s) in Front (\"\")"="355 Laser: CheckControllerStatus\n355 Laser: Laser disable\n355 Laser: Dewelling >>1000", "State(s) in (\"\")"=w2309) -> ("States Out"=w2308:string)  [unwired: 13 in]
      }
      frame "355 Laser: CheckControllerStatus" {
        # "if average < 2, laser no power\nif average 2 < average < 9.3, laser on\nif 9.3<average<10, interlock open, blink indicator\nif average > 10, laser off\n[Covers: REQ30]"
        # "take 10 measuremt and look at average"
        # "Check 355 laser controller status\nBy probing Emisison Lamp negative terminal voltage"
        n1034 = Unbundle By Name(w2318) -> ("LJ Pinout.Laser Ready"=w2321:string)
        n1035 = call "LabJack_FGV.vi"("Operation(Read)"=enum16{"Write", "Read"}."Read" ("Operation")) -> ("Read data"=w2322:i32)  [unwired: 9 in, 1 out]
        n1036 = for {
          N: 20 -> [_]
          tunnel: w2322 -> [w2333]
          tunnel: w2321 -> [w2332]
          shift-right: [w2331] -> w2314
          shift-left: w2320 -> [w2330]
          tunnel: [w2328] -> w2315 mode=indexing
          n1037 = call "LJM_eReadName.vi"("Handle In"=w2333, "Name"=w2332, "error in"=w2330) -> ("Value"=w2328:dbl, "error out"=w2331:errorcluster)  [unwired: 10 in, 1 out]
          n1038 = Wait (ms)(milliseconds to wait=u32 25) -> ()  [unwired: 1 out]
        }
        n1039 = call "checkLaserStatus.vi"("error in (no error)"=w2314, "Laser LED voltage"=w2315) -> ("error out"=w2310:errorcluster, "Interlock open?"=w2311:bool, "Laser on?"=w2312:bool, "Mean voltage"=→"laser EM lamp V":dbl)  [unwired: 6 in]
        n1040 = case shown="True" w2311 {
          frame False {
            n1041 = property on="355 Laser" class="Bool (strict)"("Blinking"=FALSE) -> ()  [unwired: 2 in, 2 out]
          }
          frame True {
            n1042 = property on="355 Laser" class="Bool (strict)"("Blinking"=TRUE) -> ()  [unwired: 2 in, 2 out]
          }
        }
        n1043 = Bundle By Name(cluster=w2318, "System Status.355 Laser"=w2312) -> (w2319:T20)
        n1044 = call <vilib>:"Add State(s) to Queue__JKI_lib_State_Machine.vi"("State(s) in (\"\")"=w2325) -> ("States Out"=w2324:string)  [unwired: 14 in]
      }
      frame "355 Laser: CheckPWMStatus" {
        # "Check 355 laser PWM status\n(Read LJ DIO#EF_ENABLE register to determine PWM status)"
        n1045 = Unbundle By Name(w2343) -> ("LJ Pinout.355 PWM"=w2342:string)
        n1046 = call "LabJack_FGV.vi"("Operation(Read)"=enum16{"Write", "Read"}."Read" ("Operation"), "error in (no error)"=w2336) -> ("error out"=w2339:errorcluster, "Read data"=w2340:i32)  [unwired: 8 in]
        n1047 = Concatenate Strings(w2342, "_EF_ENABLE" ("string")) -> (w2338:string)
        n1048 = call "LJM_eReadName.vi"("Handle In"=w2340, "Name"=w2338, "error in"=w2339) -> ("Value"=w2335:dbl, "error out"=w2337:errorcluster)  [unwired: 10 in, 1 out]
        n1049 = Greater Than 0?(x=w2335) -> (x > 0?=w2334:bool)
        n1050 = case shown="False" w2334 {
          frame False {
            # "PWM is off\nset color to gray"
            n1051 = local write "355nm Laser toggle"(FALSE ("355nm Laser")) -> ()
          }
          frame True {
            # "PWM is on\nset color to light green"
            n1052 = local write "355nm Laser toggle"(TRUE ("355nm Laser")) -> ()
          }
        }
        n1053 = call <vilib>:"Add State(s) to Queue__JKI_lib_State_Machine.vi"("State(s) in (\"\")"=w2347) -> ("States Out"=w2346:string)  [unwired: 14 in]
      }
      frame "355 Laser: Start" {
        # "Template Separator\n(You can make a copy of, or modify, this frame)"
        n1054 = call <vilib>:"Add State(s) to Queue__JKI_lib_State_Machine.vi"("State(s) in Front (\"\")"="LabJack: 355_PWM_Start", "State(s) in (\"\")"=w2355) -> ("States Out"=w2354:string)  [unwired: 13 in]
      }
      frame "355 Laser: Stop" {
        # "Template Separator\n(You can make a copy of, or modify, this frame)"
        n1055 = call <vilib>:"Add State(s) to Queue__JKI_lib_State_Machine.vi"("State(s) in Front (\"\")"="LabJack: 355_PWM_Stop", "State(s) in (\"\")"=w2361) -> ("States Out"=w2360:string)  [unwired: 13 in]
      }
      frame "---------- Utility ----------" {
        # "Template Separator\n(You can make a copy of, or modify, this frame)"
        n1056 = call <vilib>:"Add State(s) to Queue__JKI_lib_State_Machine.vi"("State(s) in (\"\")"=w2366) -> ("States Out"=w2365:string)  [unwired: 14 in]
      }
      frame "Utility: SetDataClass" {
        # "Set Data Class in Queues\n(Set data class to either Data, Bg or Cali)"
        n1057 = case shown="\"Cali\"" w2368 {
          tunnel: [enum16{"Data", "BG", "Cali"}."Data" ("Data Class") enum16{"Data", "BG", "Cali"}."BG" ("Data Class") enum16{"Data", "BG", "Cali"}."Cali" ("Data Class")] -> w2367
          frame "Data", Default {
          }
          frame "Bg" {
          }
          frame "Cali" {
          }
        }
        n1058 = local write "Data Class"(w2367) -> ()
        n1059 = call <vilib>:"Add State(s) to Queue__JKI_lib_State_Machine.vi"("State(s) in (\"\")"=w2373) -> ("States Out"=w2372:string)  [unwired: 14 in]
      }
      frame "Utility: AquiTimerReset" {
        # "Set Aquisition Timer\n(You can make a copy of, or modify, this frame)"
        n1060 = Tick Count (ms)() -> (millisecond timer value=w2379:u32)
        n1061 = Bundle By Name(cluster=w2377, "Aquisition Timer"=w2379) -> (w2378:T20)
        n1062 = call <vilib>:"Add State(s) to Queue__JKI_lib_State_Machine.vi"("State(s) in (\"\")"=w2383) -> ("States Out"=w2382:string)  [unwired: 14 in]
      }
      frame "Utility: AquiTimerCheck" {
        # "5min to ms"
        # "Set Aquisition Timer\n([Covers: REQ35])"
        n1063 = Unbundle By Name(w2391) -> ("Aquisition Timer"=w2389:u32)
        n1064 = Tick Count (ms)() -> (millisecond timer value=w2390:u32)
        n1065 = Subtract(x=w2390, y=w2389) -> (x-y=w2388:u32)
        n1066 = Multiply(x=1000, y=300) -> (x*y=w2385:i32)
        n1067 = Greater Or Equal?(x=w2388, y=w2385) -> (x >= y?=w2384:bool)
        n1068 = case shown="True" w2384 {
          frame False {
            # "do nothing"
          }
          frame True {
            # "if timed out, stop aquisition"
            n1069 = property on="StopButton" class="Bool (strict)"("Val(Sgnl)"=TRUE ("Value (Signaling)")) -> ()  [unwired: 2 in, 2 out]
          }
        }
        n1070 = call <vilib>:"Add State(s) to Queue__JKI_lib_State_Machine.vi"("State(s) in (\"\")"=w2395) -> ("States Out"=w2394:string)  [unwired: 14 in]
      }
      frame "Utility: StartBeep" {
        # "Beep\n([Covers: REQ18])"
        n1071 = call <vilib>:"Beep.vi"("use system alert? (T)"=FALSE, "duration (msec)"=u32 1000, "frequency (Hz)"=u32 2000) -> ()  [unwired: 9 in]
        n1072 = call <vilib>:"Add State(s) to Queue__JKI_lib_State_Machine.vi"("State(s) in (\"\")"=w2404) -> ("States Out"=w2403:string)  [unwired: 14 in]
      }
      frame "Utility: EndBeep" {
        # "Beep\n([Covers: REQ18])"
        n1073 = flat-sequence {
          frame #0 {
            n1074 = call <vilib>:"Beep.vi"("use system alert? (T)"=FALSE, "duration (msec)"=u32 500, "frequency (Hz)"=u32 2000) -> ()  [unwired: 9 in]
          }
          frame #1 {
            n1075 = call <vilib>:"Beep.vi"("use system alert? (T)"=FALSE, "duration (msec)"=u32 500, "frequency (Hz)"=u32 2000) -> ()  [unwired: 9 in]
          }
        }
        n1076 = call <vilib>:"Add State(s) to Queue__JKI_lib_State_Machine.vi"("State(s) in (\"\")"=w2409) -> ("States Out"=w2408:string)  [unwired: 14 in]
      }
      frame "Utility: RestoreDeConChan" {
        # "Template Separator\n(You can make a copy of, or modify, this frame)"
        n1077 = global read "GlobalVariables.vi" "DeconChan Temp"() -> (w2416:T42)
        n1078 = local write "Radio Buttons"(w2416) -> ()
        n1079 = call <vilib>:"Add State(s) to Queue__JKI_lib_State_Machine.vi"("State(s) in (\"\")"=w2421) -> ("States Out"=w2420:string)  [unwired: 14 in]
      }
      frame "Utility: SaveDeconChan" {
        # "Save Decon Channel to global temp\n(You can make a copy of, or modify, this frame)"
        n1080 = flat-sequence {
          frame #0 {
          }
          frame #1 {
            (unwired) enum32{"No Selection", "Ch1", "Ch2", "Ch3"}."No Selection" ("Radio Buttons")
          }
        }
        n1081 = flat-sequence {
          frame #0 {
            n1082 = local read "Radio Buttons"() -> (w2427:enum32{"No Selection", "Ch1", "Ch2", "Ch3"})
            n1083 = global write "GlobalVariables.vi" "DeconChan Temp"(w2427) -> ()
          }
          frame #1 {
            n1084 = local write "Radio Buttons"(enum32{"No Selection", "Ch1", "Ch2", "Ch3"}."No Selection" ("Radio Buttons")) -> ()
          }
        }
        n1085 = call <vilib>:"Add State(s) to Queue__JKI_lib_State_Machine.vi"("State(s) in (\"\")"=w2426) -> ("States Out"=w2425:string)  [unwired: 14 in]
      }
      frame "Utility: Dewelling" {
        # "Main loop dewell\n(Dewelling >> #)"
        n1086 = Fract/Exp String To Number(string=w2432, default (0 dbl)=0) -> (number=w2430:i32)  [unwired: 2 in, 1 out]
        n1087 = Wait (ms)(milliseconds to wait=w2430) -> ()  [unwired: 1 out]
        n1088 = call <vilib>:"Add State(s) to Queue__JKI_lib_State_Machine.vi"("State(s) in (\"\")"=w2436) -> ("States Out"=w2435:string)  [unwired: 14 in]
      }
      frame "Utility: SetAllChanManualGain" {
        # "Template Separator\n(You can make a copy of, or modify, this frame)"
        n1089 = property on="Auto gain ch1" class="Bool (strict)"("Val(Sgnl)"=FALSE ("Value (Signaling)")) -> ()  [unwired: 2 in, 2 out]
        n1090 = property on="Auto gain ch2" class="Bool (strict)"("Val(Sgnl)"=FALSE ("Value (Signaling)")) -> ()  [unwired: 2 in, 2 out]
        n1091 = property on="Auto gain ch3" class="Bool (strict)"("Val(Sgnl)"=FALSE ("Value (Signaling)")) -> ()  [unwired: 2 in, 2 out]
        n1092 = call <vilib>:"Add State(s) to Queue__JKI_lib_State_Machine.vi"("State(s) in (\"\")"=w2444) -> ("States Out"=w2443:string)  [unwired: 14 in]
      }
      frame "Utility: SetAllChanAutoGain" {
        # "Template Separator\n(You can make a copy of, or modify, this frame)"
        n1093 = property on="Auto gain ch1" class="Bool (strict)"("Val(Sgnl)"=TRUE ("Value (Signaling)")) -> ()  [unwired: 2 in, 2 out]
        n1094 = property on="Auto gain ch2" class="Bool (strict)"("Val(Sgnl)"=TRUE ("Value (Signaling)")) -> ()  [unwired: 2 in, 2 out]
        n1095 = property on="Auto gain ch3" class="Bool (strict)"("Val(Sgnl)"=TRUE ("Value (Signaling)")) -> ()  [unwired: 2 in, 2 out]
        n1096 = call <vilib>:"Add State(s) to Queue__JKI_lib_State_Machine.vi"("State(s) in (\"\")"=w2452) -> ("States Out"=w2451:string)  [unwired: 14 in]
      }
      frame "---------- SysLog ----------" {
        # "Template Separator\n(You can make a copy of, or modify, this frame)"
        n1097 = call <vilib>:"Add State(s) to Queue__JKI_lib_State_Machine.vi"("State(s) in (\"\")"=w2457) -> ("States Out"=w2456:string)  [unwired: 14 in]
      }
      frame "SysLog: OpenLogFile" {
        # "Template Separator\n(You can make a copy of, or modify, this frame)"
        n1098 = call <vilib>:"Add State(s) to Queue__JKI_lib_State_Machine.vi"("State(s) in (\"\")"=w2462) -> ("States Out"=w2461:string)  [unwired: 14 in]
      }
      frame "---------- Graph ----------" {
        # "Template Separator\n(You can make a copy of, or modify, this frame)"
        n1099 = call <vilib>:"Add State(s) to Queue__JKI_lib_State_Machine.vi"("State(s) in (\"\")"=w2467) -> ("States Out"=w2466:string)  [unwired: 14 in]
      }
      frame "Graph: SetXMultiplier" {
        # "Set X multiplier of WF graphs\n(You can make a copy of, or modify, this frame)"
        n1100 = call "Digitizer1_FGV.vi"() -> ("error out"=w2471:errorcluster, "Read data"=w2472:refnum<k15>)  [unwired: 10 in]
        n1101 = property class="niScope"(reference=w2472, error in=w2471) -> ("Min Sample Rate"=w2470:dbl)  [unwired: 2 out]
        n1102 = Divide(x=1.0, y=w2470) -> (x/y=w2468:dbl)
        n1103 = property on="Channel 1" class="WFGraph (strict)"("XScale.Multiplier"=w2468) -> ()  [unwired: 2 in, 2 out]
        n1104 = property on="Channel 2" class="WFGraph (strict)"("XScale.Multiplier"=w2468) -> ()  [unwired: 2 in, 2 out]
        n1105 = property on="Channel 3" class="WFGraph (strict)"("XScale.Multiplier"=w2468) -> ()  [unwired: 2 in, 2 out]
        n1106 = call <vilib>:"Add State(s) to Queue__JKI_lib_State_Machine.vi"("State(s) in (\"\")"=w2477) -> ("States Out"=w2476:string)  [unwired: 14 in]
      }
      frame "Graph: AddCursors" {
        # "Add BG and DC cursor to all graphs\n(You can make a copy of, or modify, this frame)"
        n1107 = property on="Channel 1" class="WFGraph (strict)"() -> ("XScale.Multiplier"=w2484:dbl)  [unwired: 2 in, 2 out]
        n1108 = global read "GlobalVariables.vi" "DC Idx1"() -> (w2483:i32)
        n1109 = global read "GlobalVariables.vi" "DC Idx2"() -> (w2482:i32)
        n1110 = global read "GlobalVariables.vi" "BG Idx1"() -> (w2481:i32)
        n1111 = global read "GlobalVariables.vi" "BG Idx2"() -> (w2480:i32)
        n1112 = property on="Channel 2" class="WFGraph (strict)"() -> ("CrsrList"=w2492:T21)  [unwired: 2 in, 2 out]
        n1113 = property on="Channel 3" class="WFGraph (strict)"() -> ("CrsrList"=w2491:T21)  [unwired: 2 in, 2 out]
        n1114 = property on="Channel 1" class="WFGraph (strict)"(error in=w2486) -> ("CrsrList"=w2495:T21)  [unwired: 1 in, 2 out]
        n1115 = Build Array(w2483, w2482, w2481, w2480) -> (w2479:i32[])
        n1116 = Multiply(x=w2479, y=w2484) -> (x*y=w2478:dbl[])
        n1117 = for {
          tunnel: w2495 -> [w2507] mode=indexing
          tunnel: w2478 -> [w2503] mode=indexing
          tunnel: [w2506] -> w2494 mode=indexing
          tunnel: u32[] [6618880, 6618880, 16711680, 16711680] -> [w2502] mode=indexing
          tunnel: w2492 -> [w2505] mode=indexing
          tunnel: w2491 -> [w2504] mode=indexing
          tunnel: [w2501] -> w2490 mode=indexing
          tunnel: [w2500] -> w2489 mode=indexing
          n1118 = Bundle By Name(cluster=w2507, "Position.X"=w2503, "Color"=w2502) -> (w2506:T22)
          n1119 = Bundle By Name(cluster=w2505, "Position.X"=w2503, "Color"=w2502) -> (w2501:T22)
          n1120 = Bundle By Name(cluster=w2504, "Position.X"=w2503, "Color"=w2502) -> (w2500:T22)
        }
        n1121 = control-ref of="Channel 1"() -> (w2488:refnum<vi>)
        n1122 = property on="Channel 1" class="WFGraph (strict)"("CrsrList"=w2494) -> (error out=w2485:errorcluster)  [unwired: 2 in, 1 out]
        n1123 = property on="Channel 2" class="WFGraph (strict)"("CrsrList"=w2490) -> ()  [unwired: 2 in, 2 out]
        n1124 = property on="Channel 3" class="WFGraph (strict)"("CrsrList"=w2489) -> ()  [unwired: 2 in, 2 out]
        n1125 = call "UpdateCurserIdx(SubVI).vi"("error in (no error)"=w2485, "WaveformGraph in"=w2488) -> ("error out"=w2487:errorcluster)  [unwired: 9 in]
        n1126 = call <vilib>:"Add State(s) to Queue__JKI_lib_State_Machine.vi"("State(s) in (\"\")"=w2499) -> ("States Out"=w2498:string)  [unwired: 14 in]
      }
      frame "Graph: SaveCursorLoc" {
        # "Save cursor location to ini file\n(Save cursor location to system setting ini file)"
        n1127 = global read "GlobalVariables.vi" "DC Idx1"() -> (w2514:i32)
        n1128 = global read "GlobalVariables.vi" "DC Idx2"() -> (w2513:i32)
        n1129 = global read "GlobalVariables.vi" "BG Idx1"() -> (w2512:i32)
        n1130 = global read "GlobalVariables.vi" "BG Idx2"() -> (w2511:i32)
        n1131 = Bundle("DC Idx1"=w2514, "DC Idx2"=w2513, "BG Idx1"=w2512, "BG Idx2"=w2511) -> (w2510:T43)  [unwired: 1 in]
        n1132 = call "writeCursorConfigMain.vi"("error in (no error)"=w2508, "Cursor Locations"=w2510) -> ("error out"=w2509:errorcluster)  [unwired: 9 in]
        n1133 = call <vilib>:"Add State(s) to Queue__JKI_lib_State_Machine.vi"("State(s) in (\"\")"=w2518) -> ("States Out"=w2517:string)  [unwired: 14 in]
      }
      frame "---------- APD ----------" {
        # "Template Separator\n(You can make a copy of, or modify, this frame)"
        n1134 = call <vilib>:"Add State(s) to Queue__JKI_lib_State_Machine.vi"("State(s) in (\"\")"=w2523) -> ("States Out"=w2522:string)  [unwired: 14 in]
      }
      frame "APD: Initialize" {
        w2530 = enum16{"Read", "Write"}."Write" ("Operation (Read)")
        w2529 = refnum<class "APDClass.lvclass"> refnum  # APDClass.lvclass
        # "Initialize APD FGV\n(Initialized APD FGV for holding data)"
        n1135 = call "APD1FGV.vi"("Error In"=w2524, "Operation (Read)"=w2530, "APDClass in"=w2529) -> ("Error Out"=w2528:errorcluster)  [unwired: 7 in, 1 out]
        n1136 = call "APD2FGV.vi"("Error In"=w2524, "Operation (Read)"=w2530, "APDClass in"=w2529) -> ("Error Out"=w2527:errorcluster)  [unwired: 7 in, 1 out]
        n1137 = call "APD3FGV.vi"("Error In"=w2524, "Operation (Read)"=w2530, "APDClass in"=w2529) -> ("Error Out"=w2526:errorcluster)  [unwired: 7 in, 1 out]
        n1138 = Merge Errors(w2528, w2527, w2526) -> (w2525:errorcluster)
        n1139 = call <vilib>:"Add State(s) to Queue__JKI_lib_State_Machine.vi"("State(s) in (\"\")"=w2534) -> ("States Out"=w2533:string)  [unwired: 14 in]
      }
      frame "APD: LoadFromSerial" {
        w2543 = enum16{"Read", "Write"}."Write" ("Operation (Read)")
        # "Load APD data from tdms file\n(load and update FGV)"
        n1140 = call "readAPDSerial.vi"("Error In"=w2538) -> ("Error Out"=w2537:errorcluster, "output cluster"=w2536:T44)  [unwired: 9 in]
        n1141 = Unbundle By Name(w2536) -> ("Ch1APDSerial#"=w2551:string, "Ch2APDSerial#"=w2535:string, "Ch3APDSerial#"=w2550:string)
        n1142 = call "CreatFromSerialNumNoRaw.vi"("error in (no error)"=w2537, "APD Serial #"=w2535) -> ("error out"=w2546:errorcluster, "APDClass out"=w2547:refnum<class "APDClass.lvclass">)  [unwired: 8 in]
        n1143 = call "CreatFromSerialNumNoRaw.vi"("error in (no error)"=w2537, "APD Serial #"=w2550) -> ("error out"=w2544:errorcluster, "APDClass out"=w2545:refnum<class "APDClass.lvclass">)  [unwired: 8 in]
        n1144 = call "CreatFromSerialNumNoRaw.vi"("error in (no error)"=w2537, "APD Serial #"=w2551) -> ("error out"=w2548:errorcluster, "APDClass out"=w2549:refnum<class "APDClass.lvclass">)  [unwired: 8 in]
        n1145 = call "APD1FGV.vi"("Error In"=w2548, "Operation (Read)"=w2543, "APDClass in"=w2549) -> ("Error Out"=w2542:errorcluster)  [unwired: 7 in, 1 out]
        n1146 = call "APD2FGV.vi"("Error In"=w2546, "Operation (Read)"=w2543, "APDClass in"=w2547) -> ("Error Out"=w2540:errorcluster)  [unwired: 7 in, 1 out]
        n1147 = call "APD3FGV.vi"("Error In"=w2544, "Operation (Read)"=w2543, "APDClass in"=w2545) -> ("Error Out"=w2541:errorcluster)  [unwired: 7 in, 1 out]
        n1148 = Merge Errors(w2542, w2540, w2541) -> (w2539:errorcluster)
        n1149 = call <vilib>:"Add State(s) to Queue__JKI_lib_State_Machine.vi"("State(s) in (\"\")"=w2555) -> ("States Out"=w2554:string)  [unwired: 14 in]
      }
      frame "APD: UpdateCtrlVLimit" {
        w2570 = enum16{"Read", "Write"}."Read" ("Operation (Read)")
        # "Template Separator\n(You can make a copy of, or modify, this frame)"
        n1150 = call "APD1FGV.vi"("Error In"=w2567, "Operation (Read)"=w2570) -> ("Error Out"=w2568:errorcluster, "APDClass out"=w2569:refnum<class "APDClass.lvclass">)  [unwired: 8 in]
        n1151 = call "APD2FGV.vi"("Error In"=w2567, "Operation (Read)"=w2570) -> ("Error Out"=w2565:errorcluster, "APDClass out"=w2566:refnum<class "APDClass.lvclass">)  [unwired: 8 in]
        n1152 = call "APD3FGV.vi"("Error In"=w2567, "Operation (Read)"=w2570) -> ("Error Out"=w2563:errorcluster, "APDClass out"=w2564:refnum<class "APDClass.lvclass">)  [unwired: 8 in]
        n1153 = call-dynamic "ReadMaxCtrlV.vi"("error in (no error)"=w2568, "APDClass in"=w2569) -> ("error out"=w2561:errorcluster, "Numeric"=w2558:dbl)  [unwired: 7 in, 1 out]
        n1154 = call-dynamic "ReadMaxCtrlV.vi"("error in (no error)"=w2565, "APDClass in"=w2566) -> ("error out"=w2560:errorcluster, "Numeric"=w2557:dbl)  [unwired: 7 in, 1 out]
        n1155 = call-dynamic "ReadMaxCtrlV.vi"("error in (no error)"=w2563, "APDClass in"=w2564) -> ("error out"=w2559:errorcluster, "Numeric"=w2556:dbl)  [unwired: 7 in, 1 out]
        n1156 = property on="V 1" class="DigNum (strict)"("Maximum"=w2558) -> ()  [unwired: 2 in, 2 out]
        n1157 = property on="V 2" class="DigNum (strict)"("Maximum"=w2557) -> ()  [unwired: 2 in, 2 out]
        n1158 = property on="V 3" class="DigNum (strict)"("Maximum"=w2556) -> ()  [unwired: 2 in, 2 out]
        n1159 = Merge Errors(w2561, w2560, w2559) -> (w2562:errorcluster)
        n1160 = call <vilib>:"Add State(s) to Queue__JKI_lib_State_Machine.vi"("State(s) in (\"\")"=w2574) -> ("States Out"=w2573:string)  [unwired: 14 in]
      }
      frame "APD: GetGainLimits" {
        w2589 = enum16{"Read", "Write"}."Read" ("Operation (Read)")
        # "Template Separator\n(You can make a copy of, or modify, this frame)"
        n1161 = call "APD1FGV.vi"("Error In"=w2588, "Operation (Read)"=w2589) -> ("Error Out"=w2579:errorcluster, "APDClass out"=w2580:refnum<class "APDClass.lvclass">)  [unwired: 8 in]
        n1162 = call "APD2FGV.vi"("Error In"=w2588, "Operation (Read)"=w2589) -> ("Error Out"=w2586:errorcluster, "APDClass out"=w2587:refnum<class "APDClass.lvclass">)  [unwired: 8 in]
        n1163 = call "APD3FGV.vi"("Error In"=w2588, "Operation (Read)"=w2589) -> ("Error Out"=w2584:errorcluster, "APDClass out"=w2585:refnum<class "APDClass.lvclass">)  [unwired: 8 in]
        n1164 = call-dynamic "Read Gain Limits(Log).vi"("error in (no error)"=w2579, "APDClass in"=w2580) -> ("error out"=w2578:errorcluster, "GainLimits(Log)"=w2575:cluster{"GainMax":dbl, "GainMin":dbl})  [unwired: 7 in, 1 out]
        n1165 = call-dynamic "Read Gain Limits(Log).vi"("error in (no error)"=w2586, "APDClass in"=w2587) -> ("error out"=w2582:errorcluster, "GainLimits(Log)"=w2577:cluster{"GainMax":dbl, "GainMin":dbl})  [unwired: 7 in, 1 out]
        n1166 = call-dynamic "Read Gain Limits(Log).vi"("error in (no error)"=w2584, "APDClass in"=w2585) -> ("error out"=w2581:errorcluster, "GainLimits(Log)"=w2576:cluster{"GainMax":dbl, "GainMin":dbl})  [unwired: 7 in, 1 out]
        n1167 = global write "GlobalVariables.vi" "Ch1GainLim(Log)"(w2575) -> ()
        n1168 = global write "GlobalVariables.vi" "Ch2GainLim(Log)"(w2577) -> ()
        n1169 = global write "GlobalVariables.vi" "Ch3GainLim(Log)"(w2576) -> ()
        n1170 = Merge Errors(w2578, w2582, w2581) -> (w2583:errorcluster)
        n1171 = call <vilib>:"Add State(s) to Queue__JKI_lib_State_Machine.vi"("State(s) in (\"\")"=w2593) -> ("States Out"=w2592:string)  [unwired: 14 in]
      }
      frame "---------- TCP ----------" {
        # "Template Separator\n(You can make a copy of, or modify, this frame)"
        n1172 = call <vilib>:"Add State(s) to Queue__JKI_lib_State_Machine.vi"("State(s) in (\"\")"=w2598) -> ("States Out"=w2597:string)  [unwired: 14 in]
      }
      frame "TCP: Initialize" {
        # "Initialize TCP connection to aimging beam computer\n(You can make a copy of, or modify, this frame)"
        n1173 = call <vilib>:"TCP Listen.vi"("resolve remote address (T)"=TRUE, "error in (no error)"=w2624, "timeout ms (wait forever: -1)"=2000, "port"=u16 2100, "service name"="RTLT") -> ("error out"=w2619:errorcluster, "remote address"=→"remote address":string, "connection ID"=w2620:refnum<k5>, "listener ID"=w2603:refnum<k5>)  [unwired: 2 in, 1 out]
        n1174 = TCP Read(connection ID=w2620, bytes to read=512, error in (no error)=w2619, 7:T18."CRLF" ("mode (standard)"), 9:5000 ("timeout ms (25000)")) -> (connection ID out=w2610:refnum<k5>, data out=w2616:string, error out=w2611:errorcluster)
        n1175 = Concatenate Strings("alive" ("string"), "\r\n" ("End of Line Constant")) -> (w2614:string)
        n1176 = Equal?(x=w2616, y=w2614) -> (x = y?=w2612:bool)
        n1177 = case shown="False" w2612 {
          tunnel: w2611 -> [w2628 w2649]
          tunnel: w2610 -> [_ w2643]
          tunnel: [w2629 w2647] -> w2609
          tunnel: w2607 -> [w2635 _]
          tunnel: [w2631 0] -> w2606
          tunnel: [w2630 "" ("Empty String Constant")] -> w2604
          tunnel: [FALSE TRUE] -> w2599
          frame False {
            # "if unsuccessful and count <10, increament count \nand try again"
            n1178 = Unbundle By Name(w2635) -> ("TCP attempt count"=w2632:i32)
            n1179 = Less?(x=w2632, y=3) -> (x < y?=w2633:bool)
            n1180 = case shown="True" w2633 {
              tunnel: w2632 -> [w2638 w2642]
              tunnel: [w2638 w2641] -> w2631
              tunnel: ["" ("Empty String Constant") "TCP: Initialize"] -> w2630
              tunnel: [errorcluster {"status"=TRUE, "code"=5001, "source"="TCP/IP"} ("error in (no error)") errorcluster {"status"=FALSE, "code"=5001, "source"=""} ("error in (no error)")] -> w2629
              tunnel: w2628 -> [_ _]
              frame False {
                # "send error and shut down"
              }
              frame True {
                # "try again until 10th"
                n1181 = Increment(x=w2642) -> (x+1=w2641:i32)
              }
            }
          }
          frame True {
            # "if connection is successful\nwrite TCP FVG"
            n1182 = call "TcpIDFGV.vi"("Error In"=w2649, "action"=enum16{"write", "read"}."write", "connection ID in"=w2643) -> ("Error Out"=w2647:errorcluster)  [unwired: 7 in, 1 out]
          }
        }
        n1183 = global write "GlobalVariables.vi" "TCP connected?"(w2599) -> ()
        n1184 = Bundle By Name(cluster=w2607, "TCP attempt count"=w2606, "System Status.TCP/IP"=w2599, "listener ID"=w2603) -> (w2608:T20)
        n1185 = call <vilib>:"Add State(s) to Queue__JKI_lib_State_Machine.vi"("State(s) in Front (\"\")"=w2604, "State(s) in (\"\")"=w2626) -> ("States Out"=w2625:string)  [unwired: 13 in]
      }
      frame "TCP: SyncTime" {
        # "Template Separator\n(You can make a copy of, or modify, this frame)"
        n1186 = Unbundle By Name(w2651) -> ("System Status.TCP/IP"=w2650:bool)
        n1187 = case shown="True" w2650 {
          tunnel: w2652 -> [_ w2660]
          frame False {
          }
          frame True {
            n1188 = call "TcpIDFGV.vi"("Error In"=w2660, "action"=enum16{"write", "read"}."read") -> ("Error Out"=w2659:errorcluster, "connection ID out"=w2656:refnum<k5>)  [unwired: 8 in]
            n1189 = call <userlib>:"Tick Count (ms)__ogtk.vi"("error in (no error)"=w2659) -> ("error out"=w2658:errorcluster, "millisecond timer value"=w2657:u32)  [unwired: 9 in]
            n1190 = while {
              tunnel: w2658 -> [w2680]
              tunnel: w2656 -> [w2679]
              tunnel: w2657 -> [w2668]
              stop <- w2663 stop-if-true
              n1191 = Concatenate Strings("latencycheck" ("string"), "\r\n" ("End of Line Constant")) -> (w2675:string)
              n1192 = TCP Read(connection ID=w2679, bytes to read=512, error in (no error)=w2680, 7:T18."CRLF" ("mode (standard)"), 9:2000 ("timeout ms (25000)")) -> (connection ID out=w2672:refnum<k5>, data out=w2670:string, error out=w2662:errorcluster)
              n1193 = Tick Count (ms)() -> (millisecond timer value=w2669:u32)
              n1194 = Subtract(x=w2669, y=w2668) -> (x-y=w2667:u32)
              n1195 = Equal?(x=w2670, y=w2675) -> (x = y?=w2671:bool)
              n1196 = case shown="True" w2671 {
                tunnel: w2672 -> [_ w2693]
                tunnel: w2670 -> [w2685 _]
                tunnel: [w2681 FALSE] -> w2665
                tunnel: w2662 -> [_ w2687]
                frame False {
                  n1197 = Concatenate Strings("synctimer" ("string"), "\r\n" ("End of Line Constant")) -> (w2682:string)
                  n1198 = Equal?(x=w2685, y=w2682) -> (x = y?=w2681:bool)
                  "Sync Success?" <- w2681
                }
                frame True {
                  n1199 = Concatenate Strings("latencycheck:" ("string"), "\r\n" ("End of Line Constant")) -> (w2692:string)
                  n1200 = TCP Write(connection ID=w2693, data in=w2692, error in (no error)=w2687, 9:1000 ("timeout ms (25000)")) -> (error out=w2686:errorcluster)  [unwired: 2 out]
                  n1201 = call <vilib>:"Clear Errors.vi"("error in (no error)"=w2686) -> ()  [unwired: 5 in, 2 out]
                }
              }
              n1202 = Greater?(x=w2667, y=u32 10000 ("x-y")) -> (0:w2664:bool)
              n1203 = Or(x=w2665, y=w2664) -> (x .or. y?=w2663:bool)
            }
          }
        }
        n1204 = call <vilib>:"Add State(s) to Queue__JKI_lib_State_Machine.vi"("State(s) in (\"\")"=w2655) -> ("States Out"=w2654:string)  [unwired: 14 in]
      }
      frame "TCP: SendSettingMacro" {
        # "Template Separator\n(You can make a copy of, or modify, this frame)"
        n1205 = Unbundle By Name(w2697) -> ("System Status.TCP/IP"=w2696:bool)
        n1206 = case shown="True" w2696 {
          tunnel: ["" ("Empty String Constant") "TCP: sendSubjectID\nTCP: sendScaleBarSetting\nTCP: sendScaleMaxMin\nTCP: sendDeconChannel\nTCP: sendANSI\nTCP: sendRadius\nTCP: send3Dsetting\nTCP: sendFirefly\nTCP: sendPentero"] -> w2695
          frame False {
          }
          frame True {
          }
        }
        n1207 = call <vilib>:"Add State(s) to Queue__JKI_lib_State_Machine.vi"("State(s) in Front (\"\")"=w2695, "State(s) in (\"\")"=w2700) -> ("States Out"=w2699:string)  [unwired: 13 in]
      }
      frame "TCP: sendRunNum" {
        # "Send run number to AB PC\n(You can make a copy of, or modify, this frame)"
        n1208 = Unbundle By Name(w2706) -> ("System Status.TCP/IP"=w2703:bool, "IDs.RunID"=w2707:i8)
        n1209 = case shown="True" w2703 {
          tunnel: w2707 -> [_ w2721]
          tunnel: [w2711 w2713] -> w2705
          tunnel: w2704 -> [w2711 w2712]
          frame False {
          }
          frame True {
            n1210 = Number To Decimal String(number=w2721, width (-)=i16 3) -> (decimal integer string=w2716:string)
            n1211 = call "TcpIDFGV.vi"("Error In"=w2712, "action"=enum16{"write", "read"}."read") -> ("Error Out"=w2714:errorcluster, "connection ID out"=w2718:refnum<k5>)  [unwired: 8 in]
            n1212 = Concatenate Strings("!run:", w2716) -> (w2715:string)
            n1213 = call "TCP_WriteRead.vi"("error in (no error)"=w2714, "data in"=w2715, "connectin ID in"=w2718) -> ("error out"=w2713:errorcluster)  [unwired: 4 in, 2 out]
          }
        }
        n1214 = call <vilib>:"Add State(s) to Queue__JKI_lib_State_Machine.vi"("State(s) in (\"\")"=w2710) -> ("States Out"=w2709:string)  [unwired: 14 in]
      }
      frame "TCP: sendVideoSource" {
        # "Send video source \n(You can make a copy of, or modify, this frame)"
        n1215 = Unbundle By Name(w2723) -> ("System Status.TCP/IP"=w2722:bool)
        n1216 = case shown="True" w2722 {
          tunnel: [w2729 w2731] -> w2725
          tunnel: w2724 -> [w2729 w2730]
          frame False {
          }
          frame True {
            n1217 = case shown="\"Camera\", Default" "Video Source" {
              tunnel: [0 1] -> w2736
              frame "Camera", Default {
              }
              frame "FrameGrabber" {
              }
            }
            n1218 = call "TcpIDFGV.vi"("Error In"=w2730, "action"=enum16{"write", "read"}."read") -> ("Error Out"=w2732:errorcluster, "connection ID out"=w2738:refnum<k5>)  [unwired: 8 in]
            n1219 = Number To Decimal String(number=w2736) -> (decimal integer string=w2734:string)  [unwired: 1 in]
            n1220 = Concatenate Strings("!invivo:" ("data in"), w2734) -> (w2733:string)
            n1221 = call "TCP_WriteRead.vi"("error in (no error)"=w2732, "data in"=w2733, "connectin ID in"=w2738) -> ("error out"=w2731:errorcluster)  [unwired: 4 in, 2 out]
          }
        }
        n1222 = call <vilib>:"Add State(s) to Queue__JKI_lib_State_Machine.vi"("State(s) in (\"\")"=w2728) -> ("States Out"=w2727:string)  [unwired: 14 in]
      }
      frame "TCP: startRun" {
        # "Template Separator\n(You can make a copy of, or modify, this frame)"
        n1223 = Unbundle By Name(w2743) -> ("System Status.TCP/IP"=w2742:bool)
        n1224 = case shown="True" w2742 {
          tunnel: [w2749 w2751] -> w2745
          tunnel: w2744 -> [w2749 w2750]
          frame False {
          }
          frame True {
            n1225 = call "TcpIDFGV.vi"("Error In"=w2750, "action"=enum16{"write", "read"}."read") -> ("Error Out"=w2752:errorcluster, "connection ID out"=w2753:refnum<k5>)  [unwired: 8 in]
            n1226 = call "TCP_WriteRead.vi"("error in (no error)"=w2752, "data in"="!acquire:1", "connectin ID in"=w2753) -> ("error out"=w2751:errorcluster)  [unwired: 4 in, 2 out]
          }
        }
        n1227 = call <vilib>:"Add State(s) to Queue__JKI_lib_State_Machine.vi"("State(s) in (\"\")"=w2748) -> ("States Out"=w2747:string)  [unwired: 14 in]
      }
      frame "TCP: stopRun" {
        # "Send stop run to AB PC\n(You can make a copy of, or modify, this frame)"
        n1228 = Unbundle By Name(w2757) -> ("System Status.TCP/IP"=w2756:bool)
        n1229 = case shown="True" w2756 {
          tunnel: [w2763 w2765] -> w2759
          tunnel: w2758 -> [w2763 w2764]
          frame False {
            # "if not connected, do nothing"
          }
          frame True {
            # "If TCP connected, send stop run"
            n1230 = call "TcpIDFGV.vi"("Error In"=w2764, "action"=enum16{"write", "read"}."read") -> ("Error Out"=w2766:errorcluster, "connection ID out"=w2768:refnum<k5>)  [unwired: 8 in]
            n1231 = call "TCP_WriteRead.vi"("error in (no error)"=w2766, "data in"="!acquire:0", "connectin ID in"=w2768) -> ("error out"=w2765:errorcluster)  [unwired: 4 in, 2 out]
          }
        }
        n1232 = call <vilib>:"Add State(s) to Queue__JKI_lib_State_Machine.vi"("State(s) in (\"\")"=w2762) -> ("States Out"=w2761:string)  [unwired: 14 in]
      }
      frame "TCP: SyncTimer" {
        # "Template Separator\n(You can make a copy of, or modify, this frame)"
        n1233 = call "TcpIDFGV.vi"("Error In"=w2775, "action"=enum16{"write", "read"}."read") -> ("Error Out"=w2776:errorcluster, "connection ID out"=w2777:refnum<k5>)  [unwired: 8 in]
        n1234 = while {
          tunnel: w2777 -> [w2796]
          shift-right: [w2791] -> w2771
          shift-left: w2776 -> [w2792]
          tunnel: [w2783] -> w2774
          i -> [w2788]
          stop <- w2786 stop-if-true
          n1235 = TCP Read(connection ID=w2796, bytes to read=512, error in (no error)=w2792, 7:T18."CRLF" ("mode (standard)"), 9:1000 ("timeout ms (25000)")) -> (connection ID out=w2783:refnum<k5>, data out=w2790:string, error out=w2791:errorcluster)
          "syctimer data out" <- w2790
          n1236 = Equal?(x="!synctimer:", y=w2790) -> (x = y?=w2785:bool)
          n1237 = Greater?(x=w2788, y=10000) -> (0:w2784:bool)
          n1238 = Or(x=w2785, y=w2784) -> (x .or. y?=w2786:bool)
        }
        n1239 = TCP Write(connection ID=w2774, data in="!synctimer:", error in (no error)=w2771, 9:1000 ("timeout ms (25000)")) -> (error out=w2770:errorcluster)  [unwired: 2 out]
        n1240 = call <vilib>:"Add State(s) to Queue__JKI_lib_State_Machine.vi"("State(s) in (\"\")"=w2782) -> ("States Out"=w2781:string)  [unwired: 14 in]
      }
      frame "TCP: CheckConnection" {
        # "Check TCP/IP connection statuse\n(If connection is lost, throw error)"
        n1241 = Unbundle By Name(w2798) -> ("System Status.TCP/IP"=w2797:bool)
        n1242 = case shown="True" w2797 {
          frame False {
          }
          frame True {
            # "If TCP/IP is true check, otherwise skip"
          }
        }
        n1243 = call <vilib>:"Add State(s) to Queue__JKI_lib_State_Machine.vi"("State(s) in (\"\")"=w2802) -> ("States Out"=w2801:string)  [unwired: 14 in]
      }
      frame "TCP: Close" {
        # "Close TCP connection\n()"
        n1244 = call "TcpIDFGV.vi"("Error In"=w2807, "action"=enum16{"write", "read"}."read") -> ("Error Out"=w2809:errorcluster, "connection ID out"=w2810:refnum<k5>)  [unwired: 8 in]
        n1245 = TCP Close Connection(connection ID=w2810, error in (no error)=w2809) -> (error out=w2803:errorcluster)  [unwired: 1 in, 1 out]
        n1246 = case shown="No Error" w2803 {
          tunnel: [w2815 w2816] -> w2805
          tunnel: w2804 -> [w2814 w2816]
          frame No Error {
            w2813 = FALSE ("System Status.TCP/IP")
            n1247 = Bundle By Name(cluster=w2814, "System Status.TCP/IP"=w2813) -> (w2815:T20)
            n1248 = global write "GlobalVariables.vi" "TCP connected?"(w2813) -> ()
          }
          frame Error {
          }
        }
        n1249 = call <vilib>:"Add State(s) to Queue__JKI_lib_State_Machine.vi"("State(s) in (\"\")"=w2812) -> ("States Out"=w2811:string)  [unwired: 14 in]
      }
      frame "TCP: sendSubjectID" {
        # "Send subject ID"
        n1250 = Unbundle By Name(w2818) -> ("System Status.TCP/IP"=w2817:bool, "CaseID"=w2821:string)
        n1251 = case shown="False" w2817 {
          tunnel: w2821 -> [_ w2832]
          tunnel: [w2825 w2827] -> w2820
          tunnel: w2819 -> [w2825 w2826]
          frame False {
          }
          frame True {
            n1252 = call "TcpIDFGV.vi"("Error In"=w2826, "action"=enum16{"write", "read"}."read") -> ("Error Out"=w2828:errorcluster, "connection ID out"=w2830:refnum<k5>)  [unwired: 8 in]
            n1253 = Concatenate Strings("!subject:", w2832) -> (w2829:string)
            n1254 = call "TCP_WriteRead.vi"("error in (no error)"=w2828, "data in"=w2829, "connectin ID in"=w2830) -> ("error out"=w2827:errorcluster)  [unwired: 4 in, 2 out]
          }
        }
        n1255 = call <vilib>:"Add State(s) to Queue__JKI_lib_State_Machine.vi"("State(s) in (\"\")"=w2824) -> ("States Out"=w2823:string)  [unwired: 14 in]
      }
      frame "TCP: sendScaleBarSetting" {
        # "Template Separator\n(You can make a copy of, or modify, this frame)"
        n1256 = Unbundle By Name(w2836) -> ("System Status.TCP/IP"=w2834:bool, "VideoConfig.Scale Bar"=w2835:bool)
        n1257 = case shown="False" w2834 {
          tunnel: [w2842 w2850] -> w2838
          tunnel: w2837 -> [w2842 w2849]
          tunnel: w2835 -> [_ w2848]
          frame False {
          }
          frame True {
            n1258 = Boolean To (0,1)(Boolean=w2848) -> (0, 1=w2847:i16)
            n1259 = call "TcpIDFGV.vi"("Error In"=w2849, "action"=enum16{"write", "read"}."read") -> ("Error Out"=w2851:errorcluster, "connection ID out"=w2852:refnum<k5>)  [unwired: 8 in]
            n1260 = Number To Fractional String(number=w2847, width (-)=i16 1) -> (F-format string=w2845:string)  [unwired: 2 in]
            n1261 = Concatenate Strings("!autocolor:" ("data in"), w2845) -> (w2843:string)
            n1262 = call "TCP_WriteRead.vi"("error in (no error)"=w2851, "data in"=w2843, "connectin ID in"=w2852) -> ("error out"=w2850:errorcluster)  [unwired: 4 in, 2 out]
          }
        }
        n1263 = call <vilib>:"Add State(s) to Queue__JKI_lib_State_Machine.vi"("State(s) in (\"\")"=w2841) -> ("States Out"=w2840:string)  [unwired: 14 in]
      }
      frame "TCP: sendScaleMaxMin" {
        # "Send scale bar max and min to AB PC\n(You can make a copy of, or modify, this frame)"
        n1264 = Unbundle By Name(w2857) -> ("System Status.TCP/IP"=w2854:bool, "VideoConfig.Scale Low"=w2856:dbl, "VideoConfig.Scale High"=w2855:dbl)
        n1265 = case shown="False" w2854 {
          tunnel: [w2863 w2876] -> w2859
          tunnel: w2858 -> [w2863 w2875]
          tunnel: w2856 -> [_ w2874]
          tunnel: w2855 -> [_ w2865]
          frame False {
          }
          frame True {
            n1266 = call "TcpIDFGV.vi"("Error In"=w2875, "action"=enum16{"write", "read"}."read") -> ("Error Out"=w2877:errorcluster, "connection ID out"=w2878:refnum<k5>)  [unwired: 8 in]
            n1267 = Number To Fractional String(number=w2874, width (-)=i16 4, precision (6)=i16 2) -> (F-format string=w2870:string)  [unwired: 1 in]
            n1268 = Number To Fractional String(number=w2865, width (-)=i16 4, precision (6)=i16 2) -> (F-format string=w2866:string)  [unwired: 1 in]
            n1269 = Concatenate Strings("!color:" ("string"), w2870, ";" ("string"), w2866) -> (w2864:string)
            n1270 = call "TCP_WriteRead.vi"("error in (no error)"=w2877, "data in"=w2864, "connectin ID in"=w2878) -> ("error out"=w2876:errorcluster)  [unwired: 4 in, 2 out]
          }
        }
        n1271 = call <vilib>:"Add State(s) to Queue__JKI_lib_State_Machine.vi"("State(s) in (\"\")"=w2862) -> ("States Out"=w2861:string)  [unwired: 14 in]
      }
      frame "TCP: sendDeconChannel" {
        # "Send Decon channel\n(You can make a copy of, or modify, this frame)"
        n1272 = Unbundle By Name(w2881) -> ("System Status.TCP/IP"=w2880:bool)
        n1273 = case shown="False" w2880 {
          tunnel: [w2887 w2892] -> w2883
          tunnel: w2882 -> [w2887 w2891]
          frame False {
          }
          frame True {
            n1274 = local read "Radio Buttons"() -> (w2890:enum32{"No Selection", "Ch1", "Ch2", "Ch3"})
            n1275 = Increment(x=w2890) -> (x+1=w2889:enum32{"No Selection", "Ch1", "Ch2", "Ch3"})
            n1276 = Number To Decimal String(number=w2889) -> (decimal integer string=w2888:string)  [unwired: 1 in]
            n1277 = call "TcpIDFGV.vi"("Error In"=w2891, "action"=enum16{"write", "read"}."read") -> ("Error Out"=w2893:errorcluster, "connection ID out"=w2896:refnum<k5>)  [unwired: 8 in]
            n1278 = Concatenate Strings("!channel:", w2888) -> (w2894:string)
            n1279 = call "TCP_WriteRead.vi"("error in (no error)"=w2893, "data in"=w2894, "connectin ID in"=w2896) -> ("error out"=w2892:errorcluster)  [unwired: 4 in, 2 out]
          }
        }
        n1280 = call <vilib>:"Add State(s) to Queue__JKI_lib_State_Machine.vi"("State(s) in (\"\")"=w2886) -> ("States Out"=w2885:string)  [unwired: 14 in]
      }
      frame "TCP: sendANSI" {
        # "Template Separator\n(You can make a copy of, or modify, this frame)"
        n1281 = Unbundle By Name(w2900) -> ("System Status.TCP/IP"=w2898:bool, "VideoConfig.ANSI"=w2899:dbl)
        n1282 = case shown="False" w2898 {
          tunnel: [w2906 w2912] -> w2902
          tunnel: w2901 -> [w2906 w2911]
          tunnel: w2899 -> [_ w2910]
          frame False {
          }
          frame True {
            n1283 = Number To Fractional String(number=w2910) -> (F-format string=w2908:string)  [unwired: 3 in]
            n1284 = call "TcpIDFGV.vi"("Error In"=w2911, "action"=enum16{"write", "read"}."read") -> ("Error Out"=w2913:errorcluster, "connection ID out"=w2914:refnum<k5>)  [unwired: 8 in]
            n1285 = Concatenate Strings("!ansi:" ("data in"), w2908) -> (w2907:string)
            n1286 = call "TCP_WriteRead.vi"("error in (no error)"=w2913, "data in"=w2907, "connectin ID in"=w2914) -> ("error out"=w2912:errorcluster)  [unwired: 4 in, 2 out]
          }
        }
        n1287 = call <vilib>:"Add State(s) to Queue__JKI_lib_State_Machine.vi"("State(s) in (\"\")"=w2905) -> ("States Out"=w2904:string)  [unwired: 14 in]
      }
      frame "TCP: sendRadius" {
        # "Send drawing radius to AB PC\n(You can make a copy of, or modify, this frame)"
        n1288 = Unbundle By Name(w2918) -> ("System Status.TCP/IP"=w2916:bool, "VideoConfig.Radius"=w2917:dbl)
        n1289 = case shown="False" w2916 {
          tunnel: [w2924 w2930] -> w2920
          tunnel: w2919 -> [w2924 w2929]
          tunnel: w2917 -> [_ w2928]
          frame False {
          }
          frame True {
            n1290 = Number To Fractional String(number=w2928) -> (F-format string=w2927:string)  [unwired: 3 in]
            n1291 = Concatenate Strings("!radius:" ("data in"), w2927) -> (w2925:string)
            n1292 = call "TcpIDFGV.vi"("Error In"=w2929, "action"=enum16{"write", "read"}."read") -> ("Error Out"=w2931:errorcluster, "connection ID out"=w2932:refnum<k5>)  [unwired: 8 in]
            n1293 = call "TCP_WriteRead.vi"("error in (no error)"=w2931, "data in"=w2925, "connectin ID in"=w2932) -> ("error out"=w2930:errorcluster)  [unwired: 4 in, 2 out]
          }
        }
        n1294 = call <vilib>:"Add State(s) to Queue__JKI_lib_State_Machine.vi"("State(s) in (\"\")"=w2923) -> ("States Out"=w2922:string)  [unwired: 14 in]
      }
      frame "TCP: send3Dsetting" {
        # "Send 3D setting to AB computer\n(You can make a copy of, or modify, this frame)"
        n1295 = Unbundle By Name(w2936) -> ("System Status.TCP/IP"=w2934:bool, "VideoConfig.3D?"=w2935:bool)
        n1296 = case shown="True" w2934 {
          tunnel: [w2942 w2949] -> w2938
          tunnel: w2937 -> [w2942 w2948]
          tunnel: w2935 -> [_ w2947]
          frame False {
          }
          frame True {
            n1297 = Boolean To (0,1)(Boolean=w2947) -> (0, 1=w2946:i16)
            n1298 = Number To Fractional String(number=w2946) -> (F-format string=w2945:string)  [unwired: 3 in]
            n1299 = call "TcpIDFGV.vi"("Error In"=w2948, "action"=enum16{"write", "read"}."read") -> ("Error Out"=w2950:errorcluster, "connection ID out"=w2951:refnum<k5>)  [unwired: 8 in]
            n1300 = Concatenate Strings("!3dset:" ("data in"), w2945) -> (w2943:string)
            n1301 = call "TCP_WriteRead.vi"("error in (no error)"=w2950, "data in"=w2943, "connectin ID in"=w2951) -> ("error out"=w2949:errorcluster)  [unwired: 4 in, 2 out]
          }
        }
        n1302 = call <vilib>:"Add State(s) to Queue__JKI_lib_State_Machine.vi"("State(s) in (\"\")"=w2941) -> ("States Out"=w2940:string)  [unwired: 14 in]
      }
      frame "TCP: sendFirefly" {
        # "Template Separator\n(You can make a copy of, or modify, this frame)"
        n1303 = Unbundle By Name(w2954) -> ("System Status.TCP/IP"=w2953:bool)
        n1304 = case shown="False" w2953 {
          tunnel: [w2960 w2962] -> w2956
          tunnel: w2955 -> [w2960 w2961]
          frame False {
          }
          frame True {
            n1305 = call "TcpIDFGV.vi"("Error In"=w2961, "action"=enum16{"write", "read"}."read") -> ("Error Out"=w2963:errorcluster, "connection ID out"=w2965:refnum<k5>)  [unwired: 8 in]
            n1306 = call "TCP_WriteRead.vi"("error in (no error)"=w2963, "data in"="!firefly:0", "connectin ID in"=w2965) -> ("error out"=w2962:errorcluster)  [unwired: 4 in, 2 out]
          }
        }
        n1307 = call <vilib>:"Add State(s) to Queue__JKI_lib_State_Machine.vi"("State(s) in (\"\")"=w2959) -> ("States Out"=w2958:string)  [unwired: 14 in]
      }
      frame "TCP: sendPentero" {
        # "Send Pentero setting to AB computer\n(You can make a copy of, or modify, this frame)"
        n1308 = Unbundle By Name(w2968) -> ("System Status.TCP/IP"=w2967:bool)
        n1309 = case shown="False" w2967 {
          tunnel: [w2974 w2976] -> w2970
          tunnel: w2969 -> [w2974 w2975]
          frame False {
          }
          frame True {
            n1310 = call "TcpIDFGV.vi"("Error In"=w2975, "action"=enum16{"write", "read"}."read") -> ("Error Out"=w2977:errorcluster, "connection ID out"=w2979:refnum<k5>)  [unwired: 8 in]
            n1311 = call "TCP_WriteRead.vi"("error in (no error)"=w2977, "data in"="!pentero:0", "connectin ID in"=w2979) -> ("error out"=w2976:errorcluster)  [unwired: 4 in, 2 out]
          }
        }
        n1312 = call <vilib>:"Add State(s) to Queue__JKI_lib_State_Machine.vi"("State(s) in (\"\")"=w2973) -> ("States Out"=w2972:string)  [unwired: 14 in]
      }
      frame "TCP: startCam" {
        # "Send Pentero setting to AB computer\n(You can make a copy of, or modify, this frame)"
        n1313 = Unbundle By Name(w2982) -> ("System Status.TCP/IP"=w2981:bool)
        n1314 = case shown="False" w2981 {
          tunnel: [w2988 w2990] -> w2984
          tunnel: w2983 -> [w2988 w2989]
          frame False {
          }
          frame True {
            n1315 = call "TcpIDFGV.vi"("Error In"=w2989, "action"=enum16{"write", "read"}."read") -> ("Error Out"=w2991:errorcluster, "connection ID out"=w2993:refnum<k5>)  [unwired: 8 in]
            n1316 = call "TCP_WriteRead.vi"("error in (no error)"=w2991, "data in"="!focus:1", "connectin ID in"=w2993) -> ("error out"=w2990:errorcluster)  [unwired: 4 in, 2 out]
          }
        }
        n1317 = call <vilib>:"Add State(s) to Queue__JKI_lib_State_Machine.vi"("State(s) in (\"\")"=w2987) -> ("States Out"=w2986:string)  [unwired: 14 in]
      }
      frame "TCP: stopCam" {
        # "Send Pentero setting to AB computer\n(You can make a copy of, or modify, this frame)"
        n1318 = Unbundle By Name(w2996) -> ("System Status.TCP/IP"=w2995:bool)
        n1319 = case shown="True" w2995 {
          tunnel: [w3002 w3004] -> w2998
          tunnel: w2997 -> [w3002 w3003]
          frame False {
          }
          frame True {
            n1320 = call "TcpIDFGV.vi"("Error In"=w3003, "action"=enum16{"write", "read"}."read") -> ("Error Out"=w3005:errorcluster, "connection ID out"=w3007:refnum<k5>)  [unwired: 8 in]
            n1321 = call "TCP_WriteRead.vi"("error in (no error)"=w3005, "data in"="!focus:0", "connectin ID in"=w3007) -> ("error out"=w3004:errorcluster)  [unwired: 4 in, 2 out]
          }
        }
        n1322 = call <vilib>:"Add State(s) to Queue__JKI_lib_State_Machine.vi"("State(s) in (\"\")"=w3001) -> ("States Out"=w3000:string)  [unwired: 14 in]
      }
      frame "---------- PID ----------" {
        # "Template Separator\n(You can make a copy of, or modify, this frame)"
        n1323 = call <vilib>:"Add State(s) to Queue__JKI_lib_State_Machine.vi"("State(s) in (\"\")"=w3013) -> ("States Out"=w3012:string)  [unwired: 14 in]
      }
      frame "PID: loadPID" {
        # "Template Separator\n(You can make a copy of, or modify, this frame)"
        n1324 = call "readPIDSetting.vi"("Error In"=w3017) -> ("Error Out"=w3018:errorcluster, "Ch3 PID out"=w3014:T7, "Ch2 PID out"=w3015:T7, "Ch1 PID out"=w3016:T7)  [unwired: 7 in]
        n1325 = local write "Ch3 PID gains"(w3014) -> ()
        n1326 = local write "Ch1 PID gains"(w3016) -> ()
        n1327 = local write "Ch2 PID gains"(w3015) -> ()
        n1328 = call <vilib>:"Add State(s) to Queue__JKI_lib_State_Machine.vi"("State(s) in (\"\")"=w3022) -> ("States Out"=w3021:string)  [unwired: 14 in]
      }
      frame "---------- Temp ----------" {
        # "Template Separator\n(You can make a copy of, or modify, this frame)"
        n1329 = call <vilib>:"Add State(s) to Queue__JKI_lib_State_Machine.vi"("State(s) in (\"\")"=w3027) -> ("States Out"=w3026:string)  [unwired: 14 in]
      }
    }
    n1330 = Not(x=w69) -> (.not. x?=w68:bool)
    n1331 = local write "ML?"(w68) -> ()
    "ML?" <- TRUE ("main loop running?")
  }
  n1332 = while {
    tunnel: w6 -> [w3063]
    tunnel: w5 -> [w3055]
    tunnel: [w3054] -> w4
    tunnel: w3 -> [w3044]
    tunnel: [w3043] -> w2
    shift-right: [w3035] -> _
    shift-left: _ -> [w3036]
    i -> [w3053]
    stop <- w3031 stop-if-true
    # "Read data from notifier and deconvolve it and send to Aiming Beam computer"
    n1333 = call <vilib>:"High Resolution Relative Seconds.vi"() -> ("relative seconds"=w3035:dbl)
    n1334 = Wait on Notification(notifier=w3063, ignore previous (F)=TRUE) -> (notification=w3062:T11, error out=w3047:errorcluster)  [unwired: 2 in, 2 out]
    n1335 = Subtract(x=w3035, y=w3036) -> (x-y=w3038:dbl)
    n1336 = Unbundle(w3062) -> ("CH1&2"=w3061:dbl[][], "CH3"=w3060:dbl[][], "V cluster"=w3039:cluster{"V1":dbl, "V2":dbl, "V3":dbl})  [unwired: 1 out]
    n1337 = call "SeperateChanData.vi"("Input (Ch1&2)"=w3060) -> ("Ch1"=w3057:dbl[][])  [unwired: 1 out]
    n1338 = call "SeperateChanData.vi"("Input (Ch1&2)"=w3061) -> ("Ch1"=w3059:dbl[][], "Ch2"=w3058:dbl[][])
    n1339 = Multiply(x=w3038, y=1000.0) -> (x*y=→"Decon Loop timing (ms)":dbl)
    n1340 = Index Array(array=w3059) -> (element=w3050:dbl[])  [unwired: 2 in]
    n1341 = Index Array(array=w3058) -> (element=w3049:dbl[])  [unwired: 2 in]
    n1342 = Index Array(array=w3057) -> (element=w3048:dbl[])  [unwired: 2 in]
    n1343 = case shown="\"No Selection\", Default" "Radio Buttons" {
      selector: "Radio Buttons" -> [_ w3072 w3084 w3097]
      tunnel: w3050 -> [w3071 w3080 w3090 w3102]
      tunnel: w3049 -> [w3069 w3077 w3092 w3100]
      tunnel: w3048 -> [w3067 w3075 w3087 w3105]
      tunnel: FALSE -> [_ w3083 w3095 w3107]
      tunnel: w3047 -> [w3065 w3082 w3094 w3096]
      tunnel: [w3065 w3081 w3093 w3106] -> w3031
      tunnel: [w3070 w3078 w3088 w3101] -> w3042
      tunnel: [w3068 w3076 w3089 w3099] -> w3041
      tunnel: [w3066 w3074 w3086 w3103] -> w3040
      tunnel: [0.0 ("lifetime (ns)") w3073 w3085 w3098] -> w3046
      frame "No Selection", Default {
        n1344 = Build Array(w3071) -> (w3070:dbl[][])
        n1345 = Build Array(w3069) -> (w3068:dbl[][])
        n1346 = Build Array(w3067) -> (w3066:dbl[][])
      }
      frame "Ch1" {
        n1347 = call "Deconvolution.vi"("DeconChannel"=w3072, "iRF align"=w3083, "error in (no error)"=w3082, "Waveform"=w3080) -> ("error out"=w3081:errorcluster, "lifetime (ns)"=w3073:dbl, "Fitting"=w3079:dbl[])  [unwired: 5 in]
        "Lifetime 1" <- w3073
        n1348 = Build Array(w3080, w3079) -> (w3078:dbl[][])
        n1349 = Build Array(w3077) -> (w3076:dbl[][])
        n1350 = Build Array(w3075) -> (w3074:dbl[][])
      }
      frame "Ch2" {
        n1351 = call "Deconvolution.vi"("DeconChannel"=w3084, "iRF align"=w3095, "error in (no error)"=w3094, "Waveform"=w3092) -> ("error out"=w3093:errorcluster, "lifetime (ns)"=w3085:dbl, "Fitting"=w3091:dbl[])  [unwired: 5 in]
        "Lifetime 2" <- w3085
        n1352 = Build Array(w3090) -> (w3088:dbl[][])
        n1353 = Build Array(w3092, w3091) -> (w3089:dbl[][])
        n1354 = Build Array(w3087) -> (w3086:dbl[][])
      }
      frame "Ch3" {
        n1355 = call "Deconvolution.vi"("DeconChannel"=w3097, "iRF align"=w3107, "error in (no error)"=w3096, "Waveform"=w3105) -> ("error out"=w3106:errorcluster, "lifetime (ns)"=w3098:dbl, "Fitting"=w3104:dbl[])  [unwired: 5 in]
        "Lifetime 3" <- w3098
        n1356 = Build Array(w3102) -> (w3101:dbl[][])
        n1357 = Build Array(w3100) -> (w3099:dbl[][])
        n1358 = Build Array(w3105, w3104) -> (w3103:dbl[][])
      }
    }
    n1359 = Wait Until Next ms Multiple(millisecond multiple=u32 33) -> ()  [unwired: 1 out]
    n1360 = Bundle(w3042, w3041, w3040, "V cluster"=w3039) -> (w3045:T45)  [unwired: 1 in]
    n1361 = Bundle(w3053, "lifetime (ns)"=w3046) -> (w3056:cluster{i32, "lifetime (ns)":dbl})  [unwired: 1 in]
    n1362 = Send Notification(notification=w3045, notifier=w3044, error in (no error)=w3031) -> (notifier out=w3043:refnum<notifier>, error out=w3030:errorcluster)
    n1363 = Send Notification(notification=w3056, notifier=w3055, error in (no error)=w3031) -> (notifier out=w3054:refnum<notifier>, error out=w3029:errorcluster)
    n1364 = Merge Errors(w3030, w3029) -> (→"decon error out":errorcluster)
  }
  n1365 = while {
    tunnel: w5 -> [w3118]
    shift-right: [w3111] -> _
    shift-left: u32 0 -> [w3112]
    stop <- w3109 stop-if-true
    # "Send data to AB computer here"
    # "if TCP ip is not open loop will run once and stop. To re-establish connection and start this loop. Reboot softwrae."
    # "Data communication loop"
    n1366 = Tick Count (ms)() -> (millisecond timer value=w3111:u32)
    n1367 = Wait on Notification(notifier=w3118, ignore previous (F)=FALSE) -> (notification=w3116:cluster{"idx":i32, "lifetime":dbl}, error out=w3110:errorcluster)  [unwired: 2 in, 2 out]
    n1368 = Unbundle(w3116) -> ("idx"=w3115:i32, "lifetime"=w3114:dbl)
    n1369 = global read "GlobalVariables.vi" "TCP connected?"() -> (w3108:bool)
    n1370 = Subtract(x=w3111, y=w3112) -> (x-y=→"Communication loop(ms)":u32)
    n1371 = case shown="True" w3108 {
      tunnel: w3115 -> [_ w3127]
      tunnel: w3114 -> [_ w3126]
      tunnel: w3110 -> [w3119 w3123]
      tunnel: [w3119 w3120] -> w3109
      frame False {
      }
      frame True {
        n1372 = Number To Decimal String(number=w3127) -> (decimal integer string=w3135:string)  [unwired: 1 in]
        n1373 = call "TcpIDFGV.vi"("Error In"=w3123, "action"=enum16{"write", "read"}."read") -> ("Error Out"=w3122:errorcluster, "connection ID out"=w3133:refnum<k5>)  [unwired: 8 in]
        n1374 = Concatenate Strings("!idx:", w3135) -> (w3136:string)
        n1375 = call "TCP_WriteRead.vi"("error in (no error)"=w3122, "data in"=w3136, "connectin ID in"=w3133) -> ("error out"=w3121:errorcluster, "connectin ID out"=w3134:refnum<k5>)  [unwired: 4 in, 1 out]
        n1376 = Number To Fractional String(number=w3126, precision (6)=i16 2) -> (F-format string=w3125:string)  [unwired: 2 in]
        n1377 = Concatenate Strings("!lifetime:", w3125) -> (w3132:string)
        n1378 = call "TCP_WriteRead.vi"("error in (no error)"=w3121, "data in"=w3132, "connectin ID in"=w3134) -> ("error out"=w3120:errorcluster, "data out"=→"data out(communcation loop)":string)  [unwired: 4 in, 1 out]
      }
    }
  }
  n1379 = while {
    tunnel: w3 -> [w3147]
    shift-right: [w3138] -> _
    shift-left: w1 -> [w3145]
    shift-right: [w3140] -> _
    shift-left: w1 -> [w3139]
    i -> [w3141]
    stop <- w3142 stop-if-true
    # "Data display loop(30Hz)"
    n1380 = Wait on Notification(notifier=w3147, ignore previous (F)=FALSE) -> (notification=w3143:T10, error out=w3142:errorcluster)  [unwired: 2 in, 2 out]
    n1381 = Tick Count (ms)() -> (millisecond timer value=w3138:u32)
    n1382 = Subtract(x=w3138, y=w3145) -> (x-y=→"display loop timing(ms)":u32)
    n1383 = case shown="No Error" w3142 {
      tunnel: w3143 -> [w3214 _]
      tunnel: w3139 -> [w3176 w3265]
      tunnel: [w3178 w3265] -> w3140
      tunnel: w3138 -> [w3175 _]
      frame No Error {
        w3211 = 0 ("index (row)")
        n1384 = Subtract(x=w3175, y=w3176) -> (x-y=w3177:u32)
        n1385 = Unbundle(w3214) -> ("CH1"=w3207:dbl[][], "CH2"=w3205:dbl[][], "CH3"=w3202:dbl[][], "Gain cluster"=w3181:cluster{"V1":dbl, "V2":dbl, "V3":dbl})
        n1386 = Unbundle By Name(w3181) -> ("V1"=w3165:dbl, "V2"=w3155:dbl, "V3"=w3151:dbl)
        n1387 = Index Array(array=w3207, index (row)=w3211) -> (element=w3171:dbl[])  [unwired: 1 in]
        n1388 = Index Array(array=w3205, index (row)=w3211) -> (element=w3169:dbl[])  [unwired: 1 in]
        n1389 = Index Array(array=w3202, index (row)=w3211) -> (element=w3167:dbl[])  [unwired: 1 in]
        n1390 = Array Max & Min(array=w3171) -> (max value=→"Peak1":dbl)  [unwired: 3 out]
        n1391 = Array Max & Min(array=w3169) -> (max value=→"Peak2":dbl)  [unwired: 3 out]
        n1392 = Array Max & Min(array=w3167) -> (max value=→"Peak3":dbl)  [unwired: 3 out]
        n1393 = Greater?(x=w3177, y=u32 200) -> (0:w3179:bool)
        n1394 = call "RemoveDCBG.vi"("Channel"=enum16{"DC Only", "Ch1", "Ch2", "Ch3"}."Ch2", "WF in"=w3169) -> ("DC"=w3204:dbl, "WF out"=w3173:dbl[])  [unwired: 7 in, 1 out]
        "DC2" <- w3204
        n1395 = call "RemoveDCBG.vi"("Channel"=enum16{"DC Only", "Ch1", "Ch2", "Ch3"}."Ch1", "WF in"=w3171) -> ("DC"=w3209:dbl, "WF out"=w3172:dbl[])  [unwired: 7 in, 1 out]
        "DC1" <- w3209
        n1396 = call "RemoveDCBG.vi"("Channel"=enum16{"DC Only", "Ch1", "Ch2", "Ch3"}."Ch3", "WF in"=w3167) -> ("DC"=w3201:dbl, "WF out"=w3174:dbl[])  [unwired: 7 in, 1 out]
        "DC3" <- w3201
        n1397 = call "CtrlVtoGain.vi"("CtrlV(V)"=w3165, "Channel"=enum16{"Ch1", "Ch2", "Ch3"}."Ch1") -> ("Gain"=w3162:dbl)  [unwired: 8 in, 1 out]
        n1398 = call "CtrlVtoGain.vi"("CtrlV(V)"=w3155, "Channel"=enum16{"Ch1", "Ch2", "Ch3"}."Ch2") -> ("Gain"=w3153:dbl)  [unwired: 8 in, 1 out]
        n1399 = call "CtrlVtoGain.vi"("CtrlV(V)"=w3151, "Channel"=enum16{"Ch1", "Ch2", "Ch3"}."Ch3") -> ("Gain"=w3149:dbl)  [unwired: 8 in, 1 out]
        n1400 = case shown="True" w3179 {
          tunnel: w3172 -> [_ w3229]
          tunnel: w3173 -> [_ w3233]
          tunnel: w3174 -> [_ w3232]
          tunnel: w3175 -> [_ w3249]
          tunnel: [w3221 w3249] -> w3178
          tunnel: w3176 -> [w3221 _]
          tunnel: w3162 -> [_ w3224]
          tunnel: w3153 -> [_ w3223]
          tunnel: w3149 -> [_ w3222]
          frame False {
          }
          frame True {
            # "update at 5Hz"
            n1401 = call "GetSNR(SubVI).vi"("Waveform"=w3229) -> ("SNR"=→"SNR1":dbl)  [unwired: 10 in]
            n1402 = Array Size(array=w3229) -> (size(s)=w3231:i32)
            n1403 = call "GetSNR(SubVI).vi"("Waveform"=w3233) -> ("SNR"=→"SNR2":dbl)  [unwired: 10 in]
            n1404 = call "GetSNR(SubVI).vi"("Waveform"=w3232) -> ("SNR"=→"SNR3":dbl)  [unwired: 10 in]
            n1405 = global read "GlobalVariables.vi" "BG Idx2"() -> (w3230:i32)
            n1406 = Subtract(x=w3231, y=w3230) -> (x-y=w3228:i32)
            n1407 = Array Subset(array=w3229, index=w3230, length=w3228) -> (w3237:dbl[])
            n1408 = Array Subset(array=w3233, index=w3230, length=w3228) -> (w3239:dbl[])
            n1409 = Array Subset(array=w3232, index=w3230, length=w3228) -> (w3241:dbl[])
            n1410 = Add Array Elements(numeric array=w3237) -> (sum=w3238:dbl)
            n1411 = Add Array Elements(numeric array=w3239) -> (sum=w3240:dbl)
            n1412 = Add Array Elements(numeric array=w3241) -> (sum=w3242:dbl)
            n1413 = Divide(x=w3238, y=w3224) -> (x/y=w3243:dbl)
            n1414 = Divide(x=w3240, y=w3223) -> (x/y=w3244:dbl)
            n1415 = Divide(x=w3242, y=w3222) -> (x/y=w3245:dbl)
            n1416 = Build Array(w3243, w3244, w3245) -> (w3246:dbl[])
            n1417 = Add Array Elements(numeric array=w3246) -> (sum=w3247:dbl)
            n1418 = Divide(x=w3246, y=w3247) -> (x/y=w3248:dbl[])
            n1419 = Index Array(array=w3248, index=2) -> (element=→"IntR3":dbl)
            n1420 = Index Array(array=w3248, index=1) -> (element=→"IntR2":dbl)
            n1421 = Index Array(array=w3248, index=0) -> (element=→"IntR1":dbl)
          }
        }
        n1422 = Add(x=w3174, y=w3201) -> (x+y=w3200:dbl[])
        n1423 = Add(x=w3172, y=w3209) -> (x+y=w3206:dbl[])
        n1424 = Add(x=w3173, y=w3204) -> (x+y=w3203:dbl[])
        n1425 = Less?(x=w3162, y=1.2 ("x")) -> (x < y?=w3161:bool)
        n1426 = Less?(x=w3149, y=1.2 ("x")) -> (x < y?=w3156:bool)
        n1427 = Less?(x=w3153, y=1.2 ("x")) -> (x < y?=w3158:bool)
        n1428 = case shown="False" w3156 {
          tunnel: [u32 16448250 ("Plot.Plot Color") u32 16711680 ("Plot.Plot Color")] -> w3148
          frame False {
          }
          frame True {
          }
        }
        n1429 = case shown="True" "Show BG removed?" {
          tunnel: w3207 -> [w3255 w3264]
          tunnel: w3206 -> [_ w3263]
          tunnel: [w3255 w3262] -> w3199
          tunnel: w3205 -> [w3254 w3261]
          tunnel: [w3254 w3260] -> w3193
          tunnel: w3203 -> [_ w3259]
          tunnel: w3202 -> [w3253 w3258]
          tunnel: [w3253 w3257] -> w3186
          tunnel: w3200 -> [_ w3256]
          frame False {
          }
          frame True {
            n1430 = Build Array (concatenate)(w3258, w3256) -> (w3257:dbl[][])
            n1431 = Build Array (concatenate)(w3264, w3263) -> (w3262:dbl[][])
            n1432 = Build Array (concatenate)(w3261, w3259) -> (w3260:dbl[][])
          }
        }
        "Channel 1" <- w3199
        "Channel 2" <- w3193
        "Channel 3" <- w3186
        n1433 = case shown="False" w3161 {
          tunnel: [u32 16448250 ("Plot.Plot Color") u32 16711680 ("Plot.Plot Color")] -> w3160
          frame False {
          }
          frame True {
          }
        }
        n1434 = case shown="False" w3158 {
          tunnel: [u32 16448250 ("Plot.Plot Color") u32 16711680 ("Plot.Plot Color")] -> w3152
          frame False {
          }
          frame True {
          }
        }
        n1435 = Array Size(array=w3186) -> (size(s)=w3187:i32[])
        n1436 = Array Size(array=w3199) -> (size(s)=w3198:i32[])
        n1437 = Array Size(array=w3193) -> (size(s)=w3192:i32[])
        n1438 = Index Array(array=w3187) -> (element=w3185:i32)  [unwired: 1 in]
        n1439 = Index Array(array=w3198) -> (element=w3197:i32)  [unwired: 1 in]
        n1440 = Index Array(array=w3192) -> (element=w3191:i32)  [unwired: 1 in]
        n1441 = property on="Channel 3" class="WFGraph (strict)"("Active Plot"=w3185, "Plot.Plot Color"=u32 16741120, "Plot.Line Style"=u8 1, "Plot.Line Width"=u8 2, "BG Color"=w3148) -> ()  [unwired: 2 in, 2 out]
        n1442 = property on="Channel 1" class="WFGraph (strict)"("Active Plot"=w3197, "Plot.Plot Color"=u32 16741120, "Plot.Line Style"=u8 1, "Plot.Line Width"=u8 2, "BG Color"=w3160) -> ()  [unwired: 2 in, 2 out]
        n1443 = property on="Channel 2" class="WFGraph (strict)"("Active Plot"=w3191, "Plot.Plot Color"=u32 16741120, "Plot.Line Style"=u8 1, "Plot.Line Width"=u8 2, "BG Color"=w3152) -> ()  [unwired: 2 in, 2 out]
      }
      frame Error {
      }
    }
    n1444 = Wait Until Next ms Multiple(millisecond multiple=u32 33) -> ()  [unwired: 1 out]
    "DisplayLoop" <- w3141
  }
  n1445 = while {
    tunnel: w6 -> [w3302]
    shift-right: [w3275] -> _
    shift-left: _ -> [w3297]
    i -> [w3274]
    stop <- w3287 stop-if-true
    # "Channel 3"
    # "Channel 2"
    # "Channel 1"
    # "use FGV for gain value"
    # "stop on error"
    # "Gain adjustment and Data processing"
    n1446 = Tick Count (ms)() -> (millisecond timer value=w3275:u32)
    n1447 = Wait on Notification(notifier=w3302, ignore previous (F)=TRUE) -> (notification=w3301:T11, error out=w3273:errorcluster)  [unwired: 2 in, 2 out]
    n1448 = Subtract(x=w3275, y=w3297) -> (x-y=→"PID loop timing(ms)":u32)
    n1449 = Unbundle(w3301) -> ("CH1&2"=w3289:dbl[][], "CH3"=w3288:dbl[][])  [unwired: 2 out]
    n1450 = call "SeperateChanData.vi"("Input (Ch1&2)"=w3289) -> ("Ch1"=w3283:dbl[][], "Ch2"=w3281:dbl[][])
    n1451 = call "SeperateChanData.vi"("Input (Ch1&2)"=w3288) -> ("Ch1"=w3276:dbl[][])  [unwired: 1 out]
    n1452 = call "AvgArrayTimeCritical.vi"("2D array"=w3283) -> ("1D Avg"=w3282:dbl[])  [unwired: 10 in]
    n1453 = call "AvgArrayTimeCritical.vi"("2D array"=w3281) -> ("1D Avg"=w3295:dbl[])  [unwired: 10 in]
    n1454 = call "AvgArrayTimeCritical.vi"("2D array"=w3276) -> ("1D Avg"=w3290:dbl[])  [unwired: 10 in]
    n1455 = Array Max & Min(array=w3282) -> (max value=w3280:dbl)  [unwired: 3 out]
    n1456 = Array Max & Min(array=w3295) -> (max value=w3279:dbl)  [unwired: 3 out]
    n1457 = Array Max & Min(array=w3290) -> (max value=w3277:dbl)  [unwired: 3 out]
    n1458 = local read "Auto gain ch3"() -> (w3284:bool)
    n1459 = local read "Auto gain ch2"() -> (w3285:bool)
    n1460 = local read "Auto gain ch1"() -> (w3286:bool)
    n1461 = case shown="True" w3284 {
      tunnel: w3277 -> [_ w3374]
      tunnel: "V target(1.0)" -> [_ w3372]
      tunnel: [FALSE w3367] -> w3272
      tunnel: [0.0 ("CtrlV") w3365] -> w3271
      frame False {
        # "Manual control"
      }
      frame True {
        # "PID control"
        n1462 = case shown="True" "Modulation?" {
          tunnel: w3374 -> [w3378 _]
          tunnel: w3372 -> [w3376 _]
          tunnel: [w3375 w3384] -> w3371
          frame False {
            n1463 = global read "GlobalVariables.vi" "Ch3GainLim(Log)"() -> (w3379:cluster{"GainMax":dbl, "GainMin":dbl})
            n1464 = call-poly <vilib>:"PID.vi"("output range"=w3379, "PID gains"="Ch3 PID gains", "process variable"=w3378, "setpoint"=w3376) -> ("output"=w3377:dbl)  [unwired: 6 in, 1 out]
            n1465 = Power Of 10(x=w3377) -> (10^x=w3375:dbl)
          }
          frame True {
            n1466 = Tick Count (ms)() -> (millisecond timer value=w3390:u32)
            n1467 = Divide(x=w3390, y=u32 1000) -> (x/y=w3385:dbl)
            n1468 = Multiply(x=6.283185307179586, y="f (Hz)") -> (x*y=w3386:dbl)
            n1469 = local read "Square Wave?"() -> (w3381:bool)
            n1470 = Multiply(x=w3386, y=w3385) -> (x*y=w3393:dbl)
            n1471 = Sine(x=w3393) -> (sin(x)=w3383:dbl)
            n1472 = case shown="True" w3381 {
              tunnel: w3383 -> [w3398 w3400]
              tunnel: [w3398 w3399] -> w3382
              frame False {
              }
              frame True {
                n1473 = Sign(1:w3400) -> (0:w3399:dbl)
              }
            }
            n1474 = Divide(x="aimplitude", y=0.69) -> (x/y=w3396:dbl)
            n1475 = Multiply(x=w3396, y=w3382) -> (x*y=w3392:dbl)
            n1476 = Increment(x=w3392) -> (x+1=w3391:dbl)
            n1477 = Multiply(x="Gain DC 3", y=w3391) -> (x*y=w3384:dbl)
          }
        }
        "Gain3" <- w3371
        n1478 = call "GainToCtrlV.vi"("Gain"=w3371, "Channel"=enum16{"Ch1", "Ch2", "Ch3"}."Ch3") -> ("CtrlV"=w3365:dbl)  [unwired: 8 in, 1 out]
        n1479 = call "V3FGV.vi"("action(write)"=enum16{"write", "read"}."read") -> ("Error Out"=w3366:errorcluster, "V3 out"=w3368:dbl)  [unwired: 9 in]
        n1480 = local write "V 3"(w3365) -> ()
        n1481 = Not Equal?(x=w3365, y=w3368) -> (x != y?=w3367:bool)
        n1482 = call "V3FGV.vi"("Error In"=w3366, "V3 in"=w3365) -> ()  [unwired: 8 in, 2 out]
      }
    }
    n1483 = case shown="True" w3285 {
      tunnel: w3279 -> [_ w3411]
      tunnel: "V target(1.0)" -> [_ w3412]
      tunnel: [FALSE w3405] -> w3270
      tunnel: [0.0 ("CtrlV") w3403] -> w3269
      frame False {
        # "Manual control"
      }
      frame True {
        # "PID control"
        n1484 = case shown="True" "Modulation?" {
          tunnel: w3412 -> [w3418 _]
          tunnel: w3411 -> [w3417 _]
          tunnel: [w3413 w3422] -> w3409
          frame False {
            n1485 = global read "GlobalVariables.vi" "Ch2GainLim(Log)"() -> (w3415:cluster{"GainMax":dbl, "GainMin":dbl})
            n1486 = call-poly <vilib>:"PID.vi"("output range"=w3415, "PID gains"="Ch2 PID gains", "process variable"=w3417, "setpoint"=w3418) -> ("output"=w3414:dbl)  [unwired: 6 in, 1 out]
            n1487 = Power Of 10(x=w3414) -> (10^x=w3413:dbl)
          }
          frame True {
            n1488 = Tick Count (ms)() -> (millisecond timer value=w3428:u32)
            n1489 = Divide(x=w3428, y=u32 1000) -> (x/y=w3423:dbl)
            n1490 = Multiply(x=6.283185307179586, y="f (Hz)") -> (x*y=w3424:dbl)
            n1491 = local read "Square Wave?"() -> (w3419:bool)
            n1492 = Multiply(x=w3424, y=w3423) -> (x*y=w3431:dbl)
            n1493 = Sine(x=w3431) -> (sin(x)=w3421:dbl)
            n1494 = case shown="True" w3419 {
              tunnel: w3421 -> [w3436 w3438]
              tunnel: [w3436 w3437] -> w3420
              frame False {
              }
              frame True {
                n1495 = Sign(1:w3438) -> (0:w3437:dbl)
              }
            }
            n1496 = Divide(x="aplitude", y=0.65) -> (x/y=w3434:dbl)
            n1497 = Multiply(x=w3434, y=w3420) -> (x*y=w3430:dbl)
            n1498 = Increment(x=w3430) -> (x+1=w3429:dbl)
            n1499 = Multiply(x="Gain DC", y=w3429) -> (x*y=w3422:dbl)
          }
        }
        "Gain2" <- w3409
        n1500 = call "GainToCtrlV.vi"("Gain"=w3409, "Channel"=enum16{"Ch1", "Ch2", "Ch3"}."Ch2") -> ("CtrlV"=w3403:dbl)  [unwired: 8 in, 1 out]
        n1501 = call "V2FGV.vi"("action(write)"=enum16{"write", "read"}."read") -> ("Error Out"=w3404:errorcluster, "V2 out"=w3406:dbl)  [unwired: 9 in]
        n1502 = local write "V 2"(w3403) -> ()
        n1503 = Not Equal?(x=w3403, y=w3406) -> (x != y?=w3405:bool)
        n1504 = call "V2FGV.vi"("Error In"=w3404, "V2 in"=w3403) -> ()  [unwired: 8 in, 2 out]
      }
    }
    n1505 = case shown="True" w3286 {
      tunnel: "V target(1.0)" -> [_ w3314]
      tunnel: w3280 -> [_ w3312]
      tunnel: [FALSE w3307] -> w3268
      tunnel: [0.0 ("CtrlV") w3306] -> w3267
      frame False {
        # "Manual control"
      }
      frame True {
        # "PID control"
        n1506 = case shown="True" "Modulation?" {
          tunnel: w3314 -> [w3320 _]
          tunnel: w3312 -> [w3318 _]
          tunnel: [w3315 w3333] -> w3311
          frame False {
            n1507 = global read "GlobalVariables.vi" "Ch1GainLim(Log)"() -> (w3317:cluster{"GainMax":dbl, "GainMin":dbl})
            n1508 = call-poly <vilib>:"PID.vi"("output range"=w3317, "PID gains"="Ch1 PID gains", "process variable"=w3318, "setpoint"=w3320) -> ("output"=w3316:dbl)  [unwired: 6 in, 1 out]
            n1509 = Power Of 10(x=w3316) -> (10^x=w3315:dbl)
          }
          frame True {
            n1510 = Tick Count (ms)() -> (millisecond timer value=w3330:u32)
            n1511 = Divide(x=w3330, y=u32 1000) -> (x/y=w3325:dbl)
            n1512 = Multiply(x=6.283185307179586, y="f (Hz)") -> (x*y=w3326:dbl)
            n1513 = Multiply(x=w3326, y=w3325) -> (x*y=w3334:dbl)
            n1514 = Sine(x=w3334) -> (sin(x)=w3323:dbl)
            n1515 = case shown="True" "Square Wave?" {
              tunnel: w3323 -> [w3338 w3340]
              tunnel: [w3338 w3339] -> w3322
              frame False {
              }
              frame True {
                n1516 = Sign(1:w3340) -> (0:w3339:dbl)
              }
            }
            n1517 = Divide(x="amplitude", y=0.67) -> (x/y=w3336:dbl)
            n1518 = Multiply(x=w3336, y=w3322) -> (x*y=w3332:dbl)
            n1519 = Increment(x=w3332) -> (x+1=w3331:dbl)
            n1520 = Multiply(x="Gain DC", y=w3331) -> (x*y=w3333:dbl)
          }
        }
        "Gain1" <- w3311
        n1521 = call "GainToCtrlV.vi"("Gain"=w3311, "Channel"=enum16{"Ch1", "Ch2", "Ch3"}."Ch1") -> ("CtrlV"=w3306:dbl)  [unwired: 8 in, 1 out]
        n1522 = call "V1FGV.vi"("action (write)"=enum16{"write", "read"}."read") -> ("Error Out"=w3305:errorcluster, "V1 out"=w3308:dbl)  [unwired: 9 in]
        n1523 = local write "V 1"(w3306) -> ()
        n1524 = Not Equal?(x=w3306, y=w3308) -> (x != y?=w3307:bool)
        n1525 = call "V1FGV.vi"("Error In"=w3305, "V1 in"=w3306) -> ()  [unwired: 8 in, 2 out]
      }
    }
    n1526 = call "LabJack_FGV.vi"("Operation(Read)"=enum16{"Write", "Read"}."Read" ("Operation"), "error in (no error)"=w3273) -> ("error out"=w3300:errorcluster, "Read data"=w3299:i32)  [unwired: 8 in]
    n1527 = case "Channel 1" shown="True" w3268 {
      tunnel: w3300 -> [w3356 w3362]
      tunnel: w3299 -> [w3355 w3361]
      tunnel: [w3356 w3357] -> w3294
      tunnel: [w3355 w3360] -> w3292
      tunnel: w3267 -> [_ w3358]
      frame False {
        # "Do nothing"
      }
      frame True {
        # "request V"
        n1528 = global read "GlobalVariables.vi" "Ch1 LJ pin"() -> (w3359:string)
        n1529 = call "LJM_eWriteName.vi"("Handle In"=w3361, "Name"=w3359, "Value"=w3358, "error in"=w3362) -> ("Handle Out"=w3360:i32, "error out"=w3357:errorcluster)  [unwired: 10 in]
      }
    }
    n1530 = case "Channel 2" shown="True" w3270 {
      tunnel: w3294 -> [w3347 w3354]
      tunnel: [w3347 w3349] -> w3293
      tunnel: w3292 -> [w3348 w3353]
      tunnel: [w3348 w3352] -> w3291
      tunnel: w3269 -> [_ w3350]
      frame False {
        # "Do nothing"
      }
      frame True {
        # "request V"
        n1531 = global read "GlobalVariables.vi" "Ch2 LJ pin"() -> (w3351:string)
        n1532 = call "LJM_eWriteName.vi"("Handle In"=w3353, "Name"=w3351, "Value"=w3350, "error in"=w3354) -> ("Handle Out"=w3352:i32, "error out"=w3349:errorcluster)  [unwired: 10 in]
      }
    }
    n1533 = case "Channel 3" shown="True" w3272 {
      tunnel: w3293 -> [w3341 w3346]
      tunnel: [w3341 w3342] -> w3287
      tunnel: w3291 -> [_ w3345]
      tunnel: w3271 -> [_ w3343]
      frame False {
        # "Do nothing"
      }
      frame True {
        # "request V"
        n1534 = global read "GlobalVariables.vi" "Ch3 LJ pin"() -> (w3344:string)
        n1535 = call "LJM_eWriteName.vi"("Handle In"=w3345, "Name"=w3344, "Value"=w3343, "error in"=w3346) -> ("error out"=w3342:errorcluster)  [unwired: 10 in, 1 out]
      }
    }
    "PID loop error out" <- w3287
    "PID loop" <- w3274
  }
  n1536 = disable-structure "Diagram Disable Structure" shown="Disabled" {
    frame Disabled {
      w3439 = T46 {"Horizontal"=500, "Vertical"=100}  # Top Left Corner
      n1537 = Control Help Window(0:w3439, 1:TRUE ("Show")) -> ()
    }
    frame Enabled {
    }
  }
  n1538 = while {
    tunnel: w55 -> [w3453]
    tunnel: w45 -> [w3452]
    tunnel: [w3451] -> w53
    tunnel: w6 -> [w3450]
    tunnel: [w3449] -> w49
    tunnel: w27 -> [w3447]
    tunnel: w36 -> [w3446]
    tunnel: w23 -> [w3441]
    stop <- w3444 stop-if-true
    # "acquire data and send it to processing loop"
    # "Data Aquisition Loop"
    n1539 = event shown="[1] <Start digitizer>: User Event" {
      selector: w3452 -> [_ _]
      dyn-events: [_ _] -> w3451
      timeout: 20 -> [_ _]
      tunnel: w3453 -> [w3459 w3468]
      tunnel: [w3454 _] -> w3444
      tunnel: w3450 -> [w3458 w3475]
      tunnel: [w3458 w3474] -> w3449
      tunnel: w3447 -> [_ w3472]
      tunnel: w3446 -> [w3457 w3467]
      tunnel: w3441 -> [_ w3465]
      event Timeout {
        # "use queue to stop data loop\nwhen queue ref is released, error will stop this loop"
        n1540 = event-data() -> ()  [unwired: 1 in, 3 out]
        n1541 = Get Queue Status(queue=w3459) -> (error out=w3456:errorcluster)  [unwired: 2 in, 7 out]
        n1542 = Get Queue Status(queue=w3457) -> (error out=w3455:errorcluster)  [unwired: 2 in, 7 out]
        n1543 = Merge Errors(w3456, w3455) -> (w3454:errorcluster)
      }
      event User Event {
        w3473 = enum16{"Write", "Read"}."Read" ("Operation")
        n1544 = event-data() -> ()  [unwired: 1 in, 4 out]
        n1545 = call "FLImDAQ_FGV.vi"() -> ("Read data"=w3470:T5)  [unwired: 10 in, 1 out]
        n1546 = call "Digitizer1_FGV.vi"("Operation (Read)"=w3473) -> ("Read data"=w3464:refnum<k15>)  [unwired: 9 in, 1 out]
        n1547 = call "Digitizer2_FGV.vi"("Operation (Read)"=w3473) -> ("Read data"=w3471:refnum<k15>)  [unwired: 9 in, 1 out]
        n1548 = Unbundle By Name(w3470) -> ("Waveform to Avg"=w3469:i16)
        n1549 = property on="Property Node" class="niScope"(reference=w3464) -> (reference out=w3463:refnum<k15>, "Vertical Range"=w3462:dbl, "Vertical Offset"=w3461:dbl)  [unwired: 1 in, 1 out]
        n1550 = Tick Count (ms)() -> (millisecond timer value=w3460:u32)
        n1551 = while {
          tunnel: w3475 -> [w3530]
          tunnel: [w3529] -> w3474
          tunnel: w3471 -> [w3523]
          tunnel: w3463 -> [w3522]
          tunnel: w3472 -> [w3521]
          shift-right: [w3485] -> _
          shift-left: u32 0 ("millisecond timer value") -> [w3515]
          tunnel: w3469 -> [w3512]
          tunnel: w3468 -> [w3509]
          tunnel: w3467 -> [w3507]
          tunnel: w3465 -> [w3499]
          tunnel: w3462 -> [w3496]
          tunnel: w3461 -> [w3497]
          shift-right: [w3491] -> _
          shift-left: w3460 -> [w3490]
          i -> [w3511]
          stop <- w3488 stop-if-true
          w3503 = enum16{"write", "read"}."read" ("action")
          w3516 = 65536
          # "enqueue ch34 data"
          # "enqueue V"
          # "acquire ch1&2"
          # "acquire ch3"
          # "enqueue ch12 data"
          # "send data for processing"
          n1552 = Multiply(x=w3512, y=w3511) -> (x*y=w3498:i32)
          "Fetch Record #" <- w3498
          n1553 = property on="Property Node" class="niScope"(reference=w3522, "Fetch Record Number"=w3498) -> (reference out=w3534:refnum<k15>, error out=w3533:errorcluster, "Records Done"=w3479:i32)  [unwired: 1 in]
          n1554 = Subtract(x=w3479, y=w3498) -> (x-y=→"Record Backlog":i32)
          n1555 = call-poly <instrlib>:"niScope Fetch (poly).vi"("timeout"=0.25, "error in"=w3533, "channels"="0,1", "instrument handle"=w3534) -> ("error out"=w3482:errorcluster, "wfm"=w3513:i16[][], "wfm info"=w3495:T47)  [unwired: 4 in, 1 out]
          n1556 = property on="Property Node" class="niScope"(reference=w3523, error in=w3482, "Fetch Record Number"=w3498) -> (reference out=w3527:refnum<k15>, error out=w3524:errorcluster)
          n1557 = Divide(x=w3513, y=w3516) -> (x/y=w3484:dbl[][])
          n1558 = Multiply(x=w3484, y=w3496) -> (x*y=w3520:dbl[][])
          n1559 = Tick Count (ms)() -> (millisecond timer value=w3485:u32)
          n1560 = Subtract(x=w3485, y=w3490) -> (x-y=w3494:u32)
          n1561 = Subtract(x=w3485, y=w3515) -> (x-y=→"Aquisition loop timing(ms)":u32)
          n1562 = call-poly <instrlib>:"niScope Fetch (poly).vi"("timeout"=0.25, "error in"=w3524, "channels"="0,1", "instrument handle"=w3527) -> ("error out"=w3478:errorcluster, "wfm"=w3517:i16[][])  [unwired: 4 in, 2 out]
          n1563 = Greater?(x=w3494, y=u32 1000) -> (0:w3492:bool)
          n1564 = case shown="True" w3492 {
            tunnel: w3495 -> [_ w3543]
            tunnel: w3485 -> [_ w3542]
            tunnel: [w3536 w3542] -> w3491
            tunnel: w3490 -> [w3536 _]
            tunnel: [errorcluster {"status"=FALSE, "code"=0, "source"=""} ("error constant") w3539] -> w3486
            frame False {
            }
            frame True {
              # "[Covers: REQ29]"
              n1565 = call "CheckFrequency(SubVI).vi"("wfm info"=w3543) -> ("f (Hz)"=w3541:dbl)  [unwired: 10 in]
              "Laser f (Hz)" <- w3541
              n1566 = local read "Laser Rep Rate"() -> (w3538:dbl)
              n1567 = Increment(x=w3538) -> (x+1=w3537:dbl)
              n1568 = Greater?(x=w3541, y=w3537) -> (0:w3540:bool)
              n1569 = case shown="True" w3540 {
                tunnel: [errorcluster {"status"=FALSE, "code"=0, "source"=""} ("error constant") errorcluster {"status"=TRUE, "code"=0, "source"=""} ("error constant")] -> w3539
                frame False {
                }
                frame True {
                }
              }
            }
          }
          n1570 = Add(x=w3520, y=w3497) -> (x+y=w3508:dbl[][])
          n1571 = Divide(x=w3517, y=w3516) -> (x/y=w3519:dbl[][])
          n1572 = Enqueue Element(queue=w3509, element=w3508, error in (no error)=w3478) -> (error out=w3489:errorcluster)  [unwired: 1 in, 2 out]
          n1573 = Multiply(x=w3519, y=w3496) -> (x*y=w3518:dbl[][])
          n1574 = Add(x=w3518, y=w3497) -> (x+y=w3506:dbl[][])
          n1575 = Enqueue Element(queue=w3507, element=w3506, error in (no error)=w3489) -> (error out=w3477:errorcluster)  [unwired: 1 in, 2 out]
          n1576 = call "V1FGV.vi"("Error In"=w3477, "action (write)"=w3503) -> ("Error Out"=w3505:errorcluster, "V1 out"=w3502:dbl)  [unwired: 8 in]
          n1577 = call "V2FGV.vi"("Error In"=w3505, "action(write)"=w3503) -> ("Error Out"=w3504:errorcluster, "V2 out"=w3501:dbl)  [unwired: 8 in]
          n1578 = call "V3FGV.vi"("Error In"=w3504, "action(write)"=w3503) -> ("Error Out"=w3480:errorcluster, "V3 out"=w3500:dbl)  [unwired: 8 in]
          n1579 = Bundle("V1 out"=w3502, "V2 out"=w3501, "V3 out"=w3500) -> (w3483:T48)  [unwired: 1 in]
          n1580 = Enqueue Element(queue=w3499, element=w3483, error in (no error)=w3480) -> (error out=w3476:errorcluster)  [unwired: 1 in, 2 out]
          n1581 = Bundle(w3511, w3508, w3506, w3483) -> (w3510:T49)  [unwired: 1 in]
          n1582 = Send Notification(notification=w3510, notifier=w3530, error in (no error)=w3476) -> (notifier out=w3529:refnum<notifier>, error out=w3487:errorcluster)
          n1583 = Merge Errors(w3486, w3487) -> (w3481:errorcluster)
          n1584 = case shown="Error .." w3481 {
            selector: w3481 -> [w3546 w3547]
            tunnel: w3521 -> [_ w3550]
            tunnel: [w3546 w3547] -> w3488
            frame No Error {
            }
            frame Error {
              # "Send user event to signal aquisition has stoped"
              n1585 = Generate User Event(priority (normal)=usereventprio."high priority", user event=w3550, event data cluster=TRUE ("event data")) -> ()  [unwired: 1 in, 2 out]
            }
          }
          "aquisition loop Error Out" <- w3488
        }
      }
    }
    n1586 = Unbundle By Name(w3444) -> ("status"=w3443:bool)
    n1587 = Not(x=w3443) -> (.not. x?=w3442:bool)
    n1588 = local write "Aq Loop?"(w3442) -> ()
    "Aq Loop?" <- TRUE ("Aq L?")
  }
  n1589 = Release Notifier(notifier=w2, error in (no error)=w37) -> (error out=w38:errorcluster)  [unwired: 1 in, 2 out]
  n1590 = Release Notifier(notifier=w4, error in (no error)=w26) -> (error out=w31:errorcluster)  [unwired: 1 in, 2 out]
  n1591 = call <vilib>:"Simple Error Handler.vi"("error in (no error)"=w38) -> ()  [unwired: 4 in, 5 out]
  n1592 = call <vilib>:"Simple Error Handler.vi"("error in (no error)"=w31) -> ()  [unwired: 4 in, 5 out]
  n1593 = Unregister For Events(event registration refnum=w34, error in=w41) -> (error out=w42:errorcluster)
  n1594 = Destroy User Event(user event=w27, error in=w42) -> ()  [unwired: 1 out]
  n1595 = Close File(refnum=w9, error in=w8) -> ()  [unwired: 2 out]
  n1596 = Release Notifier(notifier=w49, error in (no error)=w48) -> (error out=w47:errorcluster)  [unwired: 1 in, 2 out]
  n1597 = Unregister For Events(event registration refnum=w53, error in=w51) -> (error out=w52:errorcluster)
  n1598 = call <vilib>:"Simple Error Handler.vi"("error in (no error)"=w47) -> ()  [unwired: 4 in, 5 out]
  n1599 = Destroy User Event(user event=w43, error in=w52) -> ()  [unwired: 1 out]
